vi "Main.vi"() -> ()   [LabVIEW 2018]
uses:
  <vilib>/picture/picture.llb/imagedata.ctl
  <vilib>/Utility/miscctls.llb/LVPoint32TypeDef.ctl
  <vilib>/Utility/miscctls.llb/LVMouseTypeDef.ctl
  <vilib>/Utility/miscctls.llb/LVPositionTypeDef.ctl
  <vilib>/Utility/miscctls.llb/LVPointTypeDef.ctl
  <vilib>/Utility/miscctls.llb/LVRectTypeDef.ctl
  Shared Variables/Alarm Cluster (UI).ctl
  Shared Variables/Alarm Cluster.ctl
  Drag and Drop/State Cluster.ctl
  support/Message Queue/Message Cluster.ctl
  Drag and Drop/Thumbnail Cluster.ctl
  Drag and Drop/Object Cluster.ctl
  Drag and Drop/Object Type Enum.ctl
  Config Module/Controls/Main Config Cluster.ctl
  OPC/OPC Module Config.ctl
  Scale Module Folder/Measure Instrument/State Enum.ctl
  OPC/OPC Settings.ctl
  OPC/Variable Data Cluster.ctl
  <vilib>/OPCUA/controls/NodeId.ctl
  <vilib>/OPCUA/controls/OPC UA StatusCode.ctl
  <vilib>/OPCUA/controls/Subscription ID.ctl
  <vilib>/OPCUA/controls/OPC UA Client Refnum.ctl
  <vilib>/OPCUA/controls/Subscription Data Change.ctl
  <vilib>/OPCUA/controls/Data Type.ctl
  OPC/OPC Tag Data.ctl
  Feed Module/Controls/Feed Module Config Cluster.ctl
  Feed Module/Controls/Feed Module Settings Cluster.ctl
  Ismatec ISM 831C/Controls/Ismatech ISM831C Settings Cluster.ctl
  Masterflex 7550-30/Controls/Settings Cluster.ctl
  Mettler Toledo/Controls/Settings Cluster.ctl
  Bronkhorst M13 Flow Meter/Settings Cluster.ctl
  Measure Instrument/PID 2 Parameters Cluster.ctl
  Measure Instrument/PID Input Enum.ctl
  Measure Instrument/PID 2 Output Enum.ctl
  Tacmina QI/Tacmina QI DAQ Setting.ctl
  KNF Pump/Settings Cluster plus SIMDOS.ctl
  ASIA Pump/Pump Settings.ctl
  VICI M50 Party Mode/Settings Cluster.ctl
  FLOM Pump/Settings Cluster.ctl
  SSI PR Class/SSI PR or LD Settings Cluster.ctl
  Masterflex 75211/Masterflex 75211 DAQ Setting.ctl
  SSI PR Class/SSI P40 Settings Cluster.ctl
  Ismatec 78001/Ismatec 4083.ctl
  Bronkhorst M14 Flow Meter/Settings Cluster.ctl
  TT Module/Controls/TT Module Config Cluster.ctl
  Tag VIs/Numeric Alarm Settings Cluster.ctl
  Acquisition/Hardware Configuration.ctl
  Acquisition/Task Cluster.ctl
  PT Module/Controls/PT Module Config Cluster.ctl
  Scale Module Folder/Feed Module/Controls/Scale Module Config Cluster.ctl
  Scale Module Folder/Feed Module/Controls/Scale Module Settings Cluster.ctl
  Pump Module Folder/Pump Module Config Cluster.ctl
  Pump Module Folder/Pump Module Settings Cluster.ctl
  LabJack Module/Controls/U3 Module Config Cluster.ctl
  Decoration Module/Decoration Module Config Cluster.ctl
  Flow Module Folder/Feed Module/Controls/Flow Module Config Cluster.ctl
  Flow Module Folder/Feed Module/Controls/Flow Module Settings Cluster.ctl
  TCU Module/TCU Module Folder/TCU Module Config Cluster.ctl
  TCU Module/TCU Module Folder/TCU Module Settings Cluster.ctl
  TCU Module/TCU Module Folder/Measure Instrument/Output Devices.ctl
  Huber TCU/Huber Settings.ctl
  Lauda Integral XT-150 TCU/Lauda Settings.ctl
  Julabo Type 1 TCU/Julabo Type 1 TCU Folder/Julabo FP-50 Settings.ctl
  Huber Unistat 410 TCU/Huber Unistat 410 RS485 Settings.ctl
  D-O Module Folder/Not Sure Where this is Used.ctl
  Sequencing/Squence Control.ctl
  D-O Module Folder/D-O Module Config Cluster.ctl
  D-O Module Folder/Valve Clusters.ctl
  D-O Module Folder/D-O Module Settings Cluster.ctl
  D-O Module Folder/D-O Device Settings Cluster.ctl
  VICI Electronic Actuator/VICI Electronic Actuator Settings.ctl
  Pressure Regulator Control Module/Pressure Regulator/Controls/4-20mA Module Config Cluster.ctl
  Pressure Regulator Control Module/Pressure Regulator/Controls/4-20mA Module Settings Cluster.ctl
  Pressure Transmitter/Pressure Transmitter Device Settings.ctl
  Pressure Reg Module/Pressure Regulator Device Settings.ctl
  Sonicator Module Folder/Feed Module/Controls/Sonicator Module Config Cluster.ctl
  Sonicator Module Folder/Feed Module/Controls/Sonicator Module Settings Cluster.ctl
  Tag VIs/Tag FGV Operation Enum.ctl
  Shared Variables/Alarm Log Operation Enum.ctl
  Drag and Drop/Drop Parameters Cluster.ctl
  Drag and Drop/Module Instance Number Operation Enum.ctl
  Drag and Drop/Module Type Enum.ctl
  <vilib>/Utility/error.llb/DialogType.ctl
  Config Module/Controls/Config File Operation Enum.ctl
  Waveform Loop/Start Params Cluster.ctl
  Ismatec 78001/Ismatec 4083 Global.ctl
  Ismatec 78001/Ismatec 4083 Global Element.ctl
  Pump Calibration Program/Pump Calibration Config.ctl
  support/Message Queue/Enqueue Message (Single).vi
  <vilib>/Utility/cursorutil.llb/Set Cursor (Icon Pict).vi
  Main/Main Globals.vi
  LabJack Module/U3 (Main).vit
  D-O Module Folder/D-O Module (Main).vi
  TCU Module/TCU Module Folder/TCU Module (Main).vi
  Flow Module Folder/Flow Module (Main).vi
  Sonicator Module Folder/Sonicator Module (Main).vi
  <vilib>/Utility/cursorutil.llb/Set Cursor (Cursor ID).vi
  support/Message Queue/Message Queue.lvlib
  support/User Event - Stop/User Event - Stop.lvlib
  support/Support Library.lvlib
  Drag and Drop/Drag and Drop.lvlib
  Feed Module/Feed Module.lvlib
  TT Module/TT Module.lvlib
  History Graph/History Graph.lvlib
  Waveform Loop/Waveform Loop.lvlib
  CSV Log/CSV Log.lvlib
  TDMS Log/TDMS Log.lvlib
  Shared Variables/Dynamic Shared Variables.lvlib
  DAQ/DAQ.lvlib
  Config Module/Config Module.lvlib
  Bronkhorst M13 Flow Meter/Bronkhorst M13 Flow Meter.lvlib
  Mettler Toledo/Mettler Toledo.lvlib
  Masterflex 7550-30/Masterflex 7550-30.lvlib
  Ismatec ISM 831C/Ismatec ISM 831C.lvlib
  PT Module/PT Module.lvlib
  Scale Module Folder/Scale Module.lvlib
  Pump Module Folder/Pump Module.lvlib
  <vilib>/lvdsc/NI_DSC.lvlib
  LabJack Module/U3 Module.lvlib
  Flow Module Folder/Flow Module.lvlib
  Tacmina QI/Tacmina QI.lvlib
  KNF Pump/KNF SIMDOS.lvlib
  Huber TCU/Huber Ministat 230 TCU.lvlib
  TCU Module/TCU Module Folder/TCU Module.lvlib
  Lauda Integral XT-150 TCU/Lauda TCU.lvlib
  Julabo Type 1 TCU/Julabo Type 1 TCU Folder/Julabo Type FP-50 TCU.lvlib
  ASIA Pump.lvlib
  Sequencing/Sequencing Library.lvlib
  VICI M50 Party Mode/VICI M6 M50 Party Mode.lvlib
  D-O Module Folder/D-O Module.lvlib
  Pressure Regulator Control Module/Pressure Regulator/4-20mA Module.lvlib
  Pressure Reg Module/Pressure Regulator Library.lvlib
  Pressure Transmitter/Pressure Transmitter Library.lvlib
  FLOM Pump/FLOM Pump.lvlib
  support/Command Log VIs/Command Logging.lvlib
  Calibration VIs/Calibration.lvlib
  Lauda Integral XT-150 TCU/TCP Library.lvlib
  SSI PR Class/SSI PR or LD Pump.lvlib
  Scale Module Folder/Measure Instrument/Scale Module Engine.lvlib
  OPC/OPC UA.lvlib
  D-O Module Folder/DIO Valve/VICI Electronic Actuator.lvlib
  subVIs/Main SubVIs.lvlib
  Masterflex 75211/Masterflex 75211.lvlib
  SSI PR Class/SSI P40 Pump.lvlib
  Huber Unistat 410 TCU/Huber Unistat 410 TCU.lvlib
  Ismatec 78001/Ismatec 4308.lvlib
  Bronkhorst M14 Flow Meter/Bronkhorst M14 Flow Meter.lvlib
  Sonicator Module Folder/Sonicator Module.lvlib
panel:
  out "Cluster":T1 {"Main Config"."PR Module Configs"."Settings"."PID 2 Parameters"."output range"."output low" format="%.2f"; "Main Config"."PR Module Configs"."Settings"."PID 2 Parameters"."output range"."output high" min=0.0 max=100.0 format="%.2f"; "Main Config"."PR Module Configs"."Settings"."PID 2 Parameters"."PID gains"."derivative time (Td, min)" format="%.3f"; "Main Config"."PR Module Configs"."Settings"."PID 2 Parameters"."PID gains"."integral time (Ti, min)" format="%.3f"; "Main Config"."PR Module Configs"."Settings"."PID 2 Parameters"."PID gains"."proportional gain (Kc)" format="%.3f"; "Main Config"."Steps"."Control" items=["Pump %", "Setpoint"]; "Main Config"."TCU Module Configs"."Settings"."Huber Unistat 410 Settings"."Address" min=0 max=99 format="%02.0f"; "Main Config"."TCU Module Configs"."Settings"."Julabo FP-50 Settings"."Pump Power" min=0 max=8 step=1; "Main Config"."TCU Module Configs"."Settings"."Lauda Settings"."Pump Power" min=0 max=8 step=1; "Main Config"."Flow Module Configs"."Settings"."Bronkhorst M14 Settings"."Smoothing Steps" min=1 step=1; "Main Config"."Flow Module Configs"."Settings"."Bronkhorst M13 Settings"."Smoothing Steps" min=1 step=1; "Main Config"."Pump Module Configs"."Settings"."Ismatech 3 Channel Settings"."Channel Number" min=0 max=3; "Main Config"."Pump Module Configs"."Settings"."Ismatech 3 Channel Settings"."Pump Number" min=1; "Main Config"."Pump Module Configs"."Settings"."ASIA Pump C"."channel" min=0 max=1 step=1; "Main Config"."Pump Module Configs"."Settings"."Masterflex"."Pump Number" min=1.0 max=20.0 step=1.0; "Main Config"."Pump Module Configs"."Settings"."Ismatech"."Pump Number" min=1.0 max=20.0 step=1.0; "Main Config"."Feed Module Configs"."Settings"."Bronkhorst M14 Settings"."Smoothing Steps" min=1 step=1; "Main Config"."Feed Module Configs"."Settings"."Ismatech 3 Channel Settings"."Channel Number" min=0 max=3; "Main Config"."Feed Module Configs"."Settings"."Ismatech 3 Channel Settings"."Pump Number" min=1; "Main Config"."Feed Module Configs"."Settings"."output range"."output low" min=0.0 max=100.0 format="%.2f"; "Main Config"."Feed Module Configs"."Settings"."output range"."output high" format="%.2f"; "Main Config"."Feed Module Configs"."Settings"."PID 2 Parameters"."PID gains"."derivative time (Td, min)" format="%.3f"; "Main Config"."Feed Module Configs"."Settings"."PID 2 Parameters"."PID gains"."integral time (Ti, min)" format="%.3f"; "Main Config"."Feed Module Configs"."Settings"."PID 2 Parameters"."PID gains"."proportional gain (Kc)" format="%.3f"; "Main Config"."Feed Module Configs"."Settings"."Bronkhorst M13 Flow Meter"."Smoothing Steps" min=1 step=1; "Main Config"."Feed Module Configs"."Settings"."ASIA Pump C"."channel" min=0 max=1 step=1; "Main Config"."Feed Module Configs"."Settings"."Ismatech"."Pump Number" min=1.0 max=20.0 step=1.0; "Main Config"."Feed Module Configs"."Settings"."Masterflex"."Pump Number" min=1.0 max=20.0 step=1.0}
  in  "Alarm History Button":bool
  out "Alarm Model":T70[](array[typedef]) {"Alarm"."value" format="%.2f"; "Alarm"."setpoint" format="%.2f"; "Alarm"."clear time" format="%<%X\n%x>T"; "Alarm"."ack time" format="%<%X\n%x>T"; "Alarm"."set time" format="%<%X\n%x>T"}
  in  "UI Alarms":T71[](array[typedef])
  out "Message Data":variant
  out "data":errorcluster
  in  "End Program":bool
  out "CSV Log File":path
  out "error out":errorcluster
  in  "E-Stop":bool
  out "x-y":T4
  out "Front Panel Window:Panel Bounds":T4
  out "Drop Offset":T6
  out "Origin":T72
  out "Position":T6
  out "output cluster":cluster{"Coords":T10, "Mouse":T73}
  out "Mouse Position":cluster{"X":i32, "Y":i32}
  out "Path":path
  out "index of element":i32
  out "image data":T74
  in  "Notebook":string="Test"
  in  "Exit":bool
  in  "Settings":bool
  in  "Pause Log Button":bool
  in  "Force Trigger":bool
  in  "Start Log":bool
  out "Canvas":picture
  out "Palette":picture
  in  "?":T1 {"Main Config"."PR Module Configs"."Settings"."PID 2 Parameters"."output range"."output low" format="%.2f"; "Main Config"."PR Module Configs"."Settings"."PID 2 Parameters"."output range"."output high" min=0.0 max=100.0 format="%.2f"; "Main Config"."PR Module Configs"."Settings"."PID 2 Parameters"."PID gains"."derivative time (Td, min)" format="%.3f"; "Main Config"."PR Module Configs"."Settings"."PID 2 Parameters"."PID gains"."integral time (Ti, min)" format="%.3f"; "Main Config"."PR Module Configs"."Settings"."PID 2 Parameters"."PID gains"."proportional gain (Kc)" format="%.3f"; "Main Config"."Steps"."Control" items=["Pump %", "Setpoint"]; "Main Config"."TCU Module Configs"."Settings"."Huber Unistat 410 Settings"."Address" min=0 max=99 format="%02.0f"; "Main Config"."TCU Module Configs"."Settings"."Julabo FP-50 Settings"."Pump Power" min=0 max=8 step=1; "Main Config"."TCU Module Configs"."Settings"."Lauda Settings"."Pump Power" min=0 max=8 step=1; "Main Config"."Flow Module Configs"."Settings"."Bronkhorst M14 Settings"."Smoothing Steps" min=1 step=1; "Main Config"."Flow Module Configs"."Settings"."Bronkhorst M13 Settings"."Smoothing Steps" min=1 step=1; "Main Config"."Pump Module Configs"."Settings"."Ismatech 3 Channel Settings"."Channel Number" min=0 max=3; "Main Config"."Pump Module Configs"."Settings"."Ismatech 3 Channel Settings"."Pump Number" min=1; "Main Config"."Pump Module Configs"."Settings"."ASIA Pump C"."channel" min=0 max=1 step=1; "Main Config"."Pump Module Configs"."Settings"."Masterflex"."Pump Number" min=1.0 max=20.0 step=1.0; "Main Config"."Pump Module Configs"."Settings"."Ismatech"."Pump Number" min=1.0 max=20.0 step=1.0; "Main Config"."Feed Module Configs"."Settings"."Bronkhorst M14 Settings"."Smoothing Steps" min=1 step=1; "Main Config"."Feed Module Configs"."Settings"."Ismatech 3 Channel Settings"."Channel Number" min=0 max=3; "Main Config"."Feed Module Configs"."Settings"."Ismatech 3 Channel Settings"."Pump Number" min=1; "Main Config"."Feed Module Configs"."Settings"."output range"."output low" min=0.0 max=100.0 format="%.2f"; "Main Config"."Feed Module Configs"."Settings"."output range"."output high" format="%.2f"; "Main Config"."Feed Module Configs"."Settings"."PID 2 Parameters"."PID gains"."derivative time (Td, min)" format="%.3f"; "Main Config"."Feed Module Configs"."Settings"."PID 2 Parameters"."PID gains"."integral time (Ti, min)" format="%.3f"; "Main Config"."Feed Module Configs"."Settings"."PID 2 Parameters"."PID gains"."proportional gain (Kc)" format="%.3f"; "Main Config"."Feed Module Configs"."Settings"."Bronkhorst M13 Flow Meter"."Smoothing Steps" min=1 step=1; "Main Config"."Feed Module Configs"."Settings"."ASIA Pump C"."channel" min=0 max=1 step=1; "Main Config"."Feed Module Configs"."Settings"."Ismatech"."Pump Number" min=1.0 max=20.0 step=1.0; "Main Config"."Feed Module Configs"."Settings"."Masterflex"."Pump Number" min=1.0 max=20.0 step=1.0}
  # "little pump\ncentrifigual pump\nflow rate\npressure\nS or P to the left\nsolvent or process"
  # "Question: how do we make the live VI, such as the feed module graphic\nsized right for the picture that is loaded?\n\nProbably should standarize each module size. Then the  flow sheet\ndrawings will all just match the size and we don't have to worry about\nscale."
  # "Tasks\n1. Load graphic\n2. Drag and drop onto picture control\n3. Picture control draws hot spot\n4. If drag and drop on picture control, then resize and redraw the nearest hotspot\n5. When operator turns \"ON\" the system, then the hotspots are replaced with actual VIs."
  # "vertical or horizontal lines\nextendable"
  # "as much drawing room as possible"
  # "Scale Settings"
  # "Instrument Settings"
  # "Instrument Settings"
  # "Output Instruments"
  # "Flow Meter Settings"
  # "Output Instruments"
  # "Scale Settings"
  # "Output Instruments"
  # "Input Instruments"
  # "Scale Settings"
  # "Instrument Settings"
  # "Instrument Settings"
  # "Output Instruments"
  # "Flow Meter Settings"
  # "Output Instruments"
  # "Scale Settings"
  # "Output Instruments"
  # "Input Instruments"
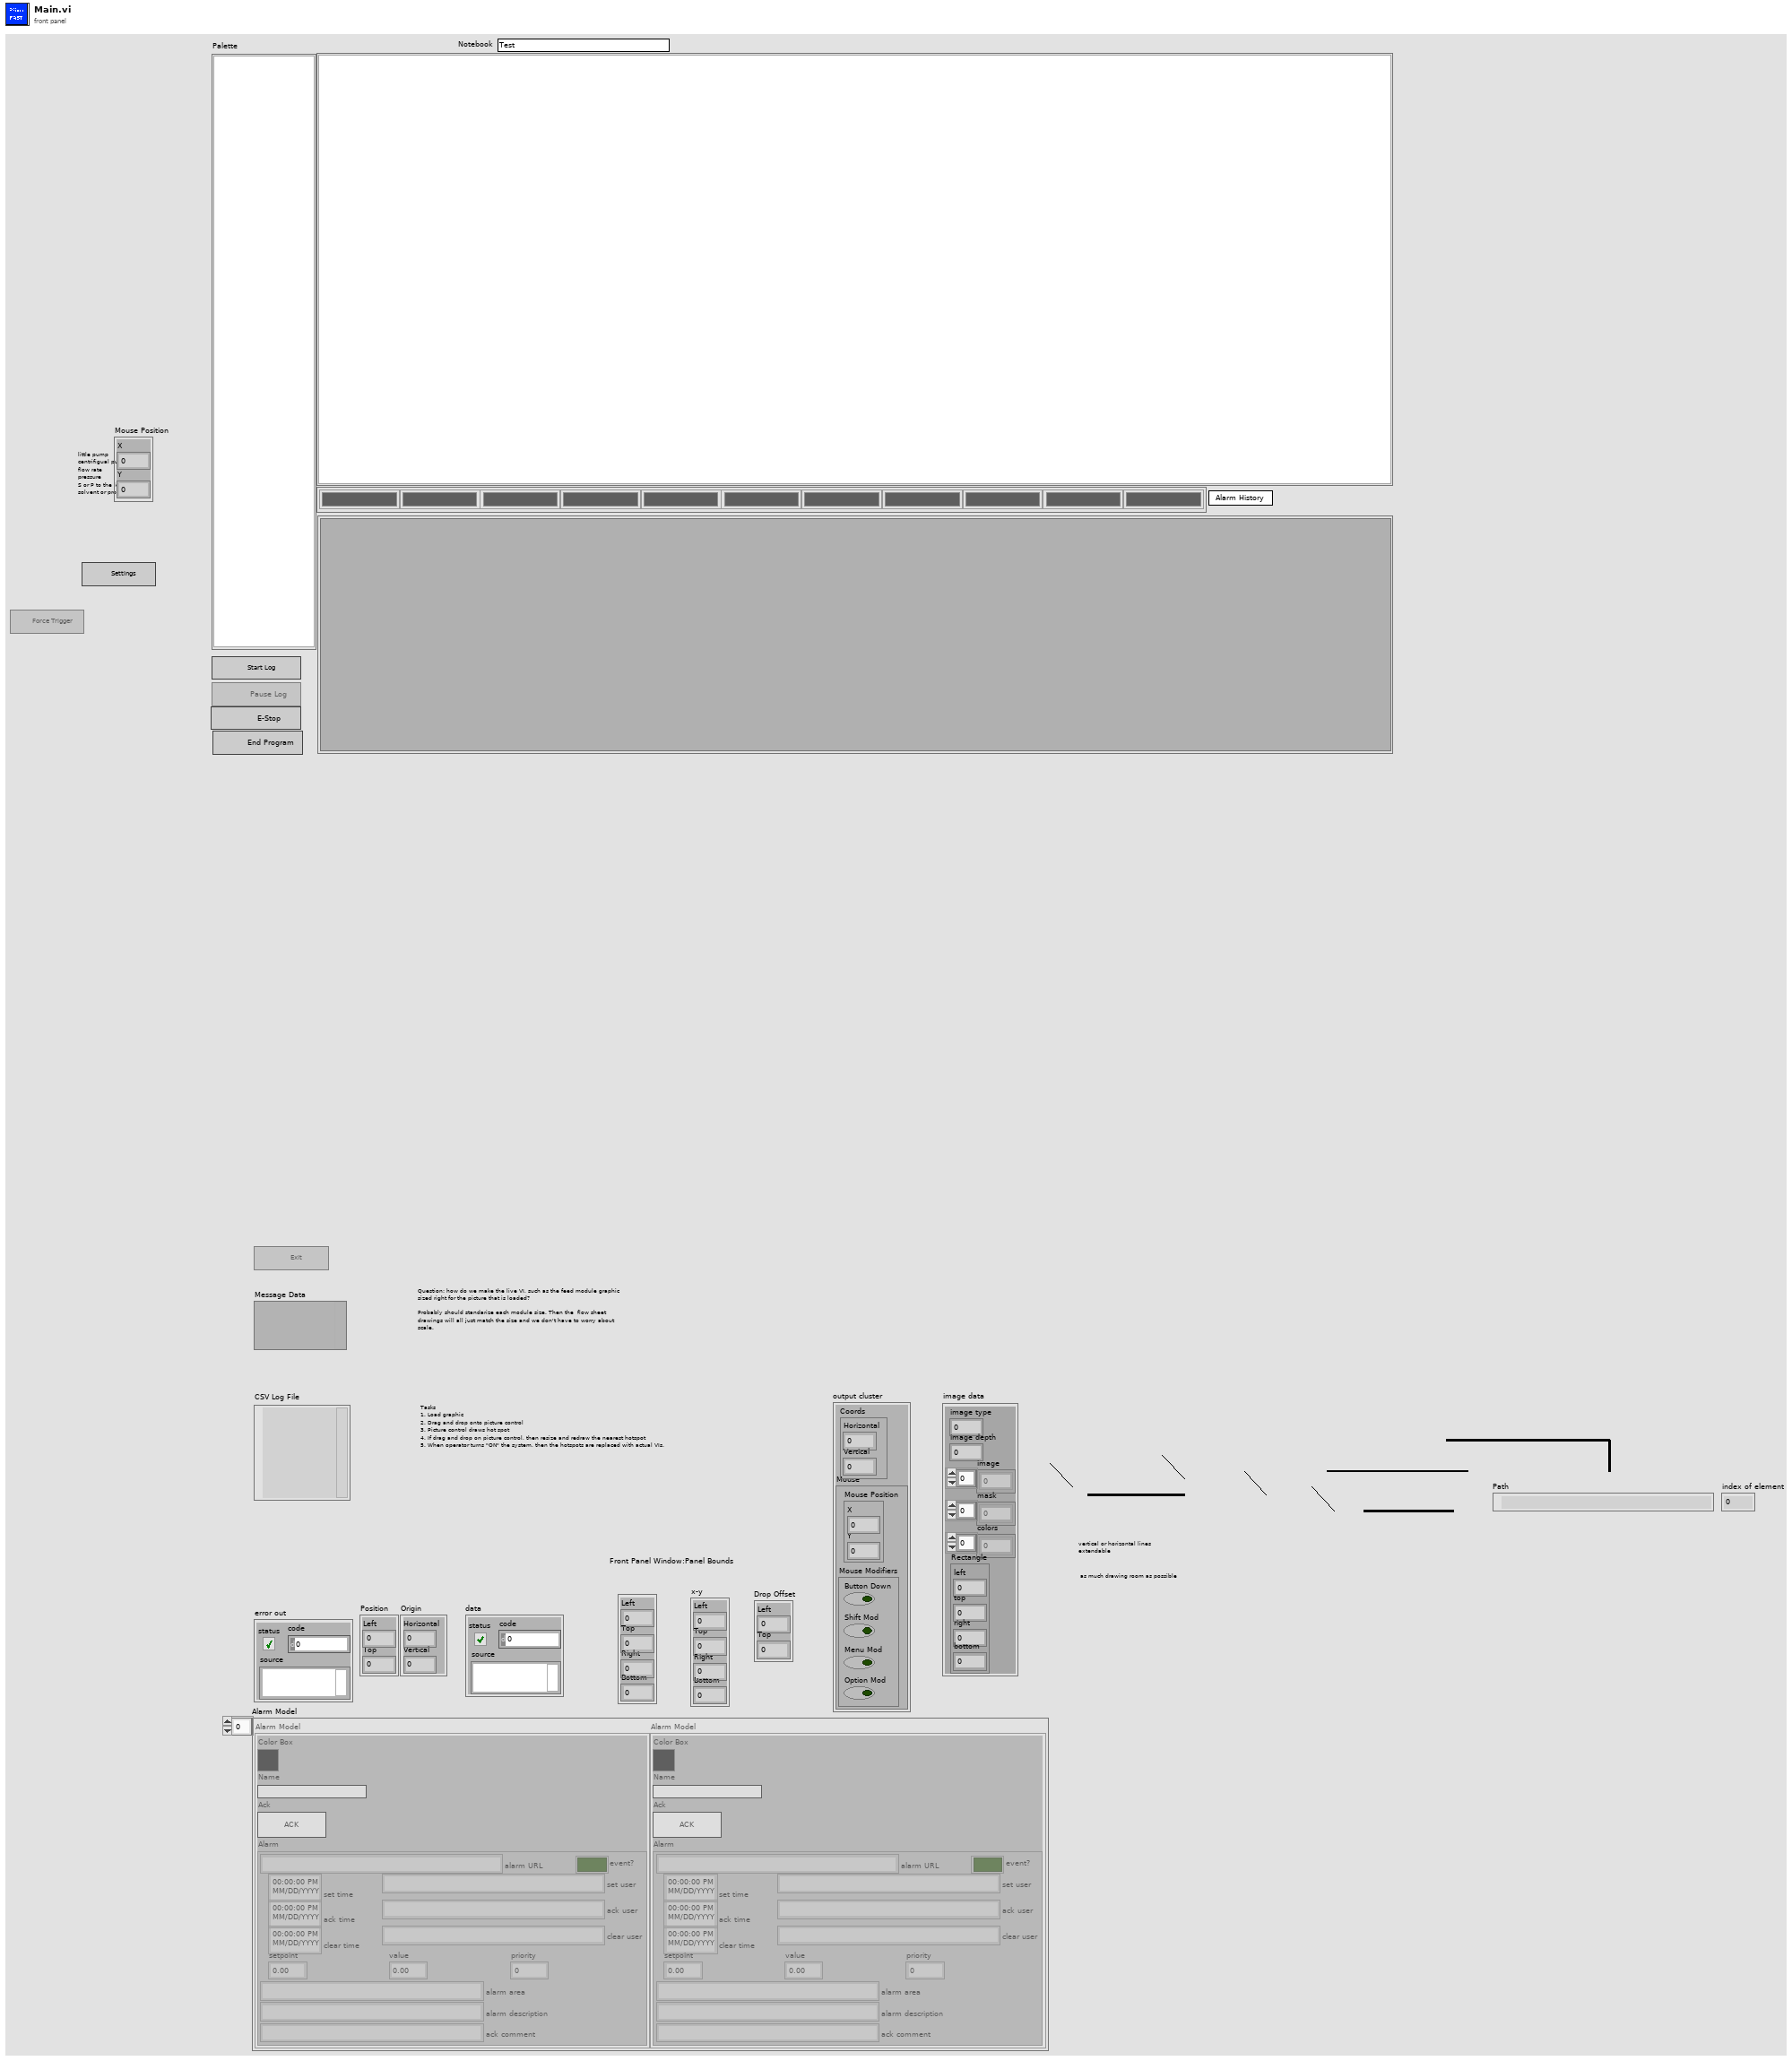
[diagram p1: front panel]
types:
  T1 = typedef "Drag and Drop.lvlib/State Cluster.ctl" = cluster{"VI refs":refnum<vi>[], "Queues":refnum<queue>[], "[Thumbnails]":T2[], "Drag Object Idx":i32, "[Objects]":T3[], "Active Object":i32, "Drop Offset":T6, "Process Name":string, "Main Config":T7, "Campaign Filepath":path, "Config Changed?":bool}
  T2 = typedef "Thumbnail Cluster.ctl" = cluster{"Path":path, "Rectangle":cluster{"left":i16, "top":i16, "right":i16, "bottom":i16}}
  T3 = typedef "Object Cluster.ctl" = cluster{"BMP Path":path, "Anchor Position":cluster{"X":i32, "Y":i32}, "Hot Spot":T4, "Type":T5, "Parameters":variant}
  T4 = typedef "LVRectTypeDef.ctl" = cluster{"Left":i16, "Top":i16, "Right":i16, "Bottom":i16}
  T5 = typedef "Object Type Enum.ctl" = enum16{"Icon", "Line", "Text", "Feed Module"}
  T6 = typedef "LVPositionTypeDef.ctl" = cluster{"Left":i32, "Top":i32}
  T7 = typedef "Config Module.lvlib/Main Config Cluster.ctl" = cluster{"Notebook":string, "OPC Module Configs":T8[], "Feed Module Configs":T18[], "Log File Path":path, "TT Module Configs":T37[], "DAQ Config":T39, "PT Module Configs":T41[], "Scale Module Configs":T42[], "Pump Module Configs":T44[], "U3 Module Configs":T46[], "Decoration Module Configs":T47[], "Flow Module Configs":T48[], "TCU Module Configs":T50[], "Steps":T57, "Abort":bool, "DO Module Configs":T59[], "PR Module Configs":T64[], "SC Module Configs":T68[], "Cycle Period":dbl}
  T8 = typedef "OPC UA.lvlib/OPC Module Config.ctl" = cluster{"State":T9, "GUID":string, "Drop Coords":T10, "Configuration":T11, "First Iteration":bool, "Data":cluster{"Object Name":string, "Variable Array":T12[]}[], "Process Name":string, "Load Count":i32, "Log Started":bool, "subscription ID out":T15, "OPC UA client refnum out":T16, "Event Registration Refnum":refnum<event-registration>, "Start Time":timestamp, "Current Time":timestamp, "Tag Data":T17[]}
  T9 = typedef "Scale Module.lvlib/Scale Module Engine.lvlib/State Enum.ctl" = enum16{"Measuring", "Idle"}
  T10 = typedef "LVPoint32TypeDef.ctl" = cluster{"Horizontal":i32, "Vertical":i32}
  T11 = typedef "OPC UA.lvlib/OPC Settings.ctl" = cluster{"Cycle Period":dbl, "server endpoint URL":string, "security policy":cluster{"message mode":enum16{"None", "Sign", "Sign and Encrypt"}, "security":enum16{"Basic256", "Basic128Rsa15"}}, "Trust Any Server":bool}
  T12 = typedef "OPC UA.lvlib/Variable Data Cluster.ctl" = cluster{"node ID":T13, "browse name":string, "status":T14, "timestamp":timestamp, "value ":variant}
  T13 = typedef "NodeId.ctl" = string
  T14 = typedef "OPC UA StatusCode.ctl" = u32
  T15 = typedef "Subscription ID.ctl" = u32
  T16 = typedef "OPC UA Client Refnum.ctl" = refnum<k21>
  T17 = typedef "OPC UA.lvlib/OPC Tag Data.ctl" = cluster{"Include this Device":bool, "Device Name":string, "OPC Tag Data":cluster{"Tag":string, "Value":variant, "Time Stamp":timestamp}[]}
  T18 = typedef "Feed Module.lvlib/Feed Module Config Cluster.ctl" = cluster{"GUID":string, "Drop Coords":T10, "Process Name":string, "Queue Name":string, "Settings":T19, "Settings Load Count":i32, "OP Load Count":i32}
  T19 = typedef "Feed Module.lvlib/Feed Module Settings Cluster.ctl" = cluster{"Cycle Period":dbl, "Ismatech":T20, "Masterflex":T21, "Mettler":T22, "Bronkhorst M13 Flow Meter":T23, "PID 2 Parameters":T24, "Manual Entry":dbl, "Auto?":bool, "output range":cluster{"output high":dbl, "output low":dbl}, "Tacmina Settings":T27, "KNF SIMDOS Settings":T28, "ASIA Pump C":T29, "VICI Settings":T30, "FLOM Settings":T31, "SSI PR/LD Settings":T32, "Masterflex 75211 Settings":T33, "SSI P40 Settings":T34, "Ismatech 3 Channel Settings":T35, "Bronkhorst M14 Settings":T36}
  T20 = typedef "Ismatec ISM 831C.lvlib/Ismatech ISM831C Settings Cluster.ctl" = cluster{"VISA resource name":refnum<visa-resource-name>, "Simulated?":bool, "Pump Number":dbl, "Reverse?":bool}
  T21 = typedef "Masterflex 7550-30.lvlib/Settings Cluster.ctl" = cluster{"VISA resource name":refnum<visa-resource-name>, "Simulated?":bool, "Pump Number":dbl, "Reverse?":bool}
  T22 = typedef "Mettler Toledo.lvlib/Settings Cluster.ctl" = cluster{"VISA resource name":refnum<visa-resource-name>, "Simulated?":bool}
  T23 = typedef "Bronkhorst M13 Flow Meter.lvlib/Settings Cluster.ctl" = cluster{"VISA resource name":refnum<visa-resource-name>, "Simulated?":bool, "Smoothing Steps":i32}
  T24 = typedef "PID 2 Parameters Cluster.ctl" = cluster{"Input Device":T25, "Output Device":T26, "Setpoint":dbl, "PID gains":cluster{"proportional gain (Kc)":dbl, "integral time (Ti, min)":dbl, "derivative time (Td, min)":dbl}}
  T25 = typedef "PID Input Enum.ctl" = enum16{"Default", "Bronkhorst M13", "Bronkhorst M14", "Scale Rate of Change"}
  T26 = typedef "PID 2 Output Enum.ctl" = enum16{"Default", "Ismatec ISM 4308", "Ismatec ISM 831C", "Masterflex 7550-30", "VICI", "Tacmina QI", "KNF SIMDOS", "ASIA Type C", "FLOM UI-22-11", "SSI PR/LD", "SSI P40", "Masterflex 75211-70"}
  T27 = typedef "Tacmina QI.lvlib/Tacmina QI DAQ Setting.ctl" = cluster{"Analog DAQ Task":refnum<k21>, "Digital DAQ Task":refnum<k21>}
  T28 = typedef "KNF SIMDOS.lvlib/Settings Cluster plus SIMDOS.ctl" = cluster{"VISA resource name":refnum<visa-resource-name>, "Simulated?":bool}
  T29 = typedef "ASIA Pump.lvlib/Pump Settings.ctl" = cluster{"ASIA Pump #":i32, "channel":i32, "Simulated":bool}
  T30 = typedef "VICI M6 M50 Party Mode.lvlib/Settings Cluster.ctl" = cluster{"VISA resource name":refnum<visa-resource-name>, "Simulated?":bool, "Pump Letter":string, "Reverse?":bool}
  T31 = typedef "FLOM Pump.lvlib/Settings Cluster.ctl" = cluster{"VISA resource name":refnum<visa-resource-name>, "Simulated?":bool, "Pump Number":dbl}
  T32 = typedef "SSI PR or LD Pump.lvlib/SSI PR or LD Settings Cluster.ctl" = cluster{"VISA resource name":refnum<visa-resource-name>, "Simulated?":bool}
  T33 = typedef "Masterflex 75211.lvlib/Masterflex 75211 DAQ Setting.ctl" = cluster{"Analog DAQ Task":refnum<k21>, "Digital DAQ Task":refnum<k21>}
  T34 = typedef "SSI P40 Pump.lvlib/SSI P40 Settings Cluster.ctl" = cluster{"VISA resource name":refnum<visa-resource-name>, "Simulated?":bool}
  T35 = typedef "Ismatec 4308.lvlib/Ismatec 4083.ctl" = cluster{"VISA resource name":refnum<visa-resource-name>, "Pump Number":i16, "Channel Number":i16, "Simulated?":bool, "Reverse?":bool}
  T36 = typedef "Bronkhorst M14 Flow Meter.lvlib/Settings Cluster.ctl" = cluster{"VISA resource name":refnum<visa-resource-name>, "Simulated?":bool, "Smoothing Steps":i32}
  T37 = typedef "TT Module.lvlib/TT Module Config Cluster.ctl" = cluster{"GUID":string, "Drop Coords":T10, "Input Channel Tag Name ":string, "Process Name":string, "Queue Name":string, "Input Channel Numeric Alarm Settings":T38[]}
  T38 = typedef "Numeric Alarm Settings Cluster.ctl" = cluster{"enable? (F)":bool, "name":string, "alarm type":enum16{"HI_HI", "HI", "LO", "LO_LO"}, "level/change":dbl, "deadband/time":dbl, "alarm delay":dbl, "priority":u32, "ack type":enum16{"Auto", "User", "None", "Each Occurrence"}, "area":string, "description":string, "log? (T)":bool}
  T39 = typedef "DAQ.lvlib/Hardware Configuration.ctl" = cluster{"Tasks":T40[]}
  T40 = typedef "Task Cluster.ctl" = cluster{"DAQmx Task":refnum<k21>, "Read-Write Radio":enum32{"Read", "Write"}}
  T41 = typedef "PT Module.lvlib/PT Module Config Cluster.ctl" = cluster{"GUID":string, "Drop Coords":T10, "Input Channel Tag Name ":string, "Process Name":string, "Queue Name":string, "Input Channel Numeric Alarm Settings":T38[]}
  T42 = typedef "Scale Module.lvlib/Scale Module Config Cluster.ctl" = cluster{"GUID":string, "Drop Coords":T10, "Process Name":string, "Queue Name":string, "Settings":T43, "Load Count":i32}
  T43 = typedef "Scale Module.lvlib/Scale Module Settings Cluster.ctl" = cluster{"Cycle Period":dbl, "Mettler":T22, "Scale Type":string}
  T44 = typedef "Pump Module.lvlib/Pump Module Config Cluster.ctl" = cluster{"GUID":string, "Drop Coords":T10, "Process Name":string, "Queue Name":string, "Settings":T45, "Load Count":i32}
  T45 = typedef "Pump Module.lvlib/Pump Module Settings Cluster.ctl" = cluster{"Cycle Period":dbl, "Manual Entry":dbl, "Output Device":T26, "Ismatech":T20, "Ismatech 3 Channel Settings":T35, "Masterflex":T21, "VICI Settings":T30, "Tacmina Settings":T27, "KNF SIMDOS Settings":T28, "ASIA Pump C":T29, "FLOM Settings":T31, "SSI PR/LD Settings":T32, "SSI P40 Settings":T32, "Masterflex 75211 Settings":T33, "Pump Calibration File":path, "Calibration Slope":dbl, "Calibration Y Intercept":dbl, "Pump Cal Enum":u16}
  T46 = typedef "U3 Module.lvlib/U3 Module Config Cluster.ctl" = cluster{"GUID":string, "Drop Coords":T10, "AI Channel Number":enum16{"Default", "AI0", "AI1", "AI2", "AI3", "AI4", "AI5", "AI6", "AI7"}, "Process Name":string, "Queue Name":string, "Input Channel Numeric Alarm Settings":T38[]}
  T47 = typedef "Decoration Module Config Cluster.ctl" = cluster{"GUID":string, "Drop Coords":T10, "Decoration Filepath":path}
  T48 = typedef "Flow Module.lvlib/Flow Module Config Cluster.ctl" = cluster{"GUID":string, "Drop Coords":T10, "Process Name":string, "Queue Name":string, "Settings":T49, "Load Count":i32}
  T49 = typedef "Flow Module.lvlib/Flow Module Settings Cluster.ctl" = cluster{"Cycle Period":dbl, "Flow Meter Type":string, "Bronkhorst M13 Settings":T23, "Bronkhorst M14 Settings":T36}
  T50 = typedef "TCU Module.lvlib/TCU Module Config Cluster.ctl" = cluster{"GUID":string, "Drop Coords":T10, "Process Name":string, "Queue Name":string, "Settings":T51, "Load Count":i32, "Power Level Changed":bool}
  T51 = typedef "TCU Module.lvlib/TCU Module Settings Cluster.ctl" = cluster{"Cycle Period":dbl, "Setpoint Entry":dbl, "Output Device":T52, "Huber Ministat 230 Settings":T53, "Lauda Settings":T54, "Julabo FP-50 Settings":T55, "Internal Control?":bool, "Huber Unistat 410 Settings":T56}
  T52 = typedef "Output Devices.ctl" = enum16{"Default", "Huber Ministat 230", "Huber Unistat 410", "Lauda XT-150", "Julabo FP-50"}
  T53 = typedef "Huber Ministat 230 TCU.lvlib/Huber Settings.ctl" = cluster{"VISA resource name":refnum<visa-resource-name>, "Simulated?":bool}
  T54 = typedef "Lauda TCU.lvlib/Lauda Settings.ctl" = cluster{"VISA resource name":refnum<visa-resource-name>, "Simulated?":bool, "Pump Power":i32}
  T55 = typedef "Julabo Type FP-50 TCU.lvlib/Julabo FP-50 Settings.ctl" = cluster{"VISA resource name":refnum<visa-resource-name>, "Simulated?":bool, "Pump Power":i32}
  T56 = typedef "Huber Unistat 410 TCU.lvlib/Huber Unistat 410 RS485 Settings.ctl" = cluster{"VISA resource name":refnum<visa-resource-name>, "Address":i8, "Simulated?":bool}
  T57 = typedef "Not Sure Where this is Used.ctl" = T58[]
  T58 = typedef "Sequencing Library.lvlib/Squence Control.ctl" = cluster{"Module":string, "Control":u16, "Value":dbl, "Wait (sec)":dbl}
  T59 = typedef "D-O Module.lvlib/D-O Module Config Cluster.ctl" = cluster{"GUID":string, "Drop Coords":T10, "Process Name":string, "Queue Name":string, "Settings":T60, "Load Count":i32}
  T60 = typedef "D-O Module.lvlib/Valve Clusters.ctl" = cluster{"Valve Settings":T61, "Valve Type":enum16{"Default", "Digital Output Valve", "VICI Electronic Actuator"}, "Time On (Sec)":dbl, "Time Off (Sec)":dbl, "Run?":bool}
  T61 = typedef "D-O Module.lvlib/D-O Module Settings Cluster.ctl" = cluster{"D-O Settings":T62, "VICI Electronic Actuator":T63}
  T62 = typedef "D-O Module.lvlib/D-O Device Settings Cluster.ctl" = cluster{"DAQmx Task Name":refnum<k21>, "Output Channel":u16, "Output Channel Names":string[]}
  T63 = typedef "VICI Electronic Actuator.lvlib/VICI Electronic Actuator Settings.ctl" = cluster{"VISA resource name":refnum<visa-resource-name>, "Mode":enum16{"Two Positions With Stops", "Two Positions Without Stops", "Mutiposition"}, "Simulated":bool}
  T64 = typedef "4-20mA Module.lvlib/4-20mA Module Config Cluster.ctl" = cluster{"GUID":string, "Drop Coords":T10, "Process Name":string, "Queue Name":string, "Settings":T65, "Settings Load Count":i32}
  T65 = typedef "4-20mA Module.lvlib/4-20mA Module Settings Cluster.ctl" = cluster{"Cycle Period":dbl, "PID 2 Parameters":cluster{"Input Device":enum16{"Default", "4-20mA"}, "Output Device":enum16{"Default", "Equilibar Pressure Reg", "Flow Regulator"}, "Setpoint":dbl, "PID gains":cluster{"proportional gain (Kc)":dbl, "integral time (Ti, min)":dbl, "derivative time (Td, min)":dbl}, "output range":cluster{"output low":dbl, "output high":dbl}}, "Manual Entry":dbl, "Auto?":bool, "4-20mA Input Settings":T66, "4-20mA Out Settings":T67, "Input Channel Tag Name ":string}
  T66 = typedef "Pressure Transmitter Library.lvlib/Pressure Transmitter Device Settings.ctl" = cluster{"Input Channel ":u16}
  T67 = typedef "Pressure Regulator Library.lvlib/Pressure Regulator Device Settings.ctl" = cluster{"Output DAQ Task":refnum<k21>}
  T68 = typedef "Sonicator Module.lvlib/Sonicator Module Config Cluster.ctl" = cluster{"GUID":string, "Drop Coords":T10, "Process Name":string, "Queue Name":string, "Settings":T69, "Load Count":i32}
  T69 = typedef "Sonicator Module.lvlib/Sonicator Module Settings Cluster.ctl" = cluster{"Cycle Period":dbl, "Mettler":T22, "Scale Type":string}
  T70 = typedef "Dynamic Shared Variables.lvlib/Alarm Cluster.ctl" = cluster{"Color Box":u32, "Name":string, "Ack":bool, "Alarm":cluster{"alarm URL":string, "set time":timestamp, "set user":string, "ack time":timestamp, "ack user":string, "clear time":timestamp, "clear user":string, "setpoint":dbl, "value":dbl, "priority":u32, "alarm area":string, "alarm description":string, "ack comment":string, "event?":bool, "Refnum":u64}}
  T71 = typedef "Dynamic Shared Variables.lvlib/Alarm Cluster (UI).ctl" = cluster{"Color Box":u32, "Name":string, "Ack":bool}
  T72 = typedef "LVPointTypeDef.ctl" = cluster{"Horizontal":i16, "Vertical":i16}
  T73 = typedef "LVMouseTypeDef.ctl" = cluster{"Mouse Position":cluster{"X":i32, "Y":i32}, "Mouse Modifiers":cluster{"Button Down":bool, "Shift Mod":bool, "Menu Mod":bool, "Option Mod":bool}}
  T74 = typedef "imagedata.ctl" = cluster{"image type":i32, "image depth":i32, "image":u8[], "mask":u8[], "colors":u32[], "Rectangle":cluster{"left":i16, "top":i16, "right":i16, "bottom":i16}}
  T75 = typedef "Tag FGV Operation Enum.ctl" = enum16{"Init", "Set Notification Queue", "Create Tag", "Commit", "Write Tag (Numeric)", "Write Tag (Boolean)", "Read All Tags", "Read One Tag", "Delete Tag Category", "Set Alarm Parameters (Numeric)", "Set Alarm Parameters (Boolean)", "Enable All Alarms", "Disable All Alarms", "Delete All Tags", "Read Alarms", "Ack Alarm", "Read Alarm Parameters (Numeric)", "Read Alarm Parameters (Boolean)"}
  T76 = cluster{"Down":bool, "Mouse":T73, "Drag":bool, "Canvas":bool}
  T77 = cluster{"Busy":bool, "PumpCnt":dbl, "RemoteEntered":bool, "OverpressureSet":bool}[]
  T78 = typedef "Main Queue Cluster.ctl" = cluster{"UI":refnum<queue>, "Waveform Loop":refnum<queue>, "CSV Log":refnum<queue>, "TDMS Log":refnum<queue>, "Graphs":refnum<queue>[], "DAQ":refnum<queue>, "Sequence":refnum<queue>, "TCP Write":refnum<queue>, "Sequence UI":refnum<queue>, "OPC UA Log":refnum<queue>, "TCP Read":refnum<queue>}
  T79 = cluster{"Event Registration Refnum":refnum<event-registration>, "Stop Event Registration Refnum":refnum<event-registration>}
  T80 = typedef "Drag and Drop.lvlib/Module Type Enum.ctl" = enum16{"<unknown module>", "Feed", "TT", "PT", "Scale", "Flow", "Pump", "U3", "TCU", "DO", "PR", "OPC", "SC"}
  T81 = typedef "Module Instance Number Operation Enum.ctl" = enum16{"Init", "Next Instance Number"}
  T82 = typedef "Drop Parameters Cluster.ctl" = cluster{"Module VI Filepath":path, "Process Name":string, "Main UI Message Queue":refnum<queue>, "Drop Coords":T10, "Module Parameters":variant, "Name of Parent Window":string}
  T83 = enum8{"Enabled", "Disabled", "Disabled and Grayed Out"}
  T84 = typedef "Config Module.lvlib/Config File Operation Enum.ctl" = enum16{"Read", "Write"}
  T85 = typedef "Alarm Log Operation Enum.ctl" = enum16{"Create Log", "Log Alarm", "Close Log"}
  T86 = typedef "Waveform Loop.lvlib/Start Params Cluster.ctl" = cluster{"dt (seconds)":dbl, "CSV Logfile path":path, "TDMS Logfile path":path}
  T87 = typedef "Ismatec 4308.lvlib/Ismatec 4083 Global.ctl" = T88[]
  T88 = typedef "Ismatec 4308.lvlib/Ismatec 4083 Global Element.ctl" = cluster{"Busy":bool, "ChannelCnt":dbl, "Initialized":bool, "Current Channel":dbl, "Initialized Channels":dbl[]}
  T89 = typedef "Calibration.lvlib/Pump Calibration Config.ctl" = cluster{"Settings":cluster{"Cycle Period":dbl, "Ismatech":T20, "Masterflex":T21, "Bronkhorst M13 Settings":T23, "PID 2 Parameters":cluster{"Input Device":T25, "Output Device":T26}, "Tacmina Settings":T27, "KNF SIMDOS Settings":T28, "VICI M50 Settings":T30, "FLOM Settings":T31, "Calibration Limits":cluster{"Minimum (ml/min)":dbl, "Maximum (ml/min)":dbl, "Steps":dbl}, "SSI PR Settings":T32, "Ismatech 4308 Settings":T35, "Bronkhorst M14 Settings":T36}, "Flowmeter Output":dbl, "Density":dbl, "FL Temp":dbl, "Speed %":dbl, "File Refnum":refnum<file>, "Pump On?":enum16{"Off", "On", "Not Initialized"}}
  T90 = typedef "DialogType.ctl" = u16
  T91 = enum32{"Invalid", "Standard", "Closed", "Hidden", "Minimized", "Maximized"}
  T92 = cluster{"alarm URL":string, "set time":timestamp, "set user":string, "ack time":timestamp, "ack user":string, "clear time":timestamp, "clear user":string, "setpoint":dbl, "value":dbl, "priority":u32, "alarm area":string, "alarm description":string, "ack comment":string, "event?":bool, "Refnum":u64}[]
  T93 = cluster{"alarm URL":string, "set time":timestamp, "set user":string, "ack time":timestamp, "ack user":string, "clear time":timestamp, "clear user":string, "setpoint":dbl, "value":dbl, "priority":u32, "alarm area":string, "alarm description":string, "ack comment":string, "event?":bool, "Refnum":u64}
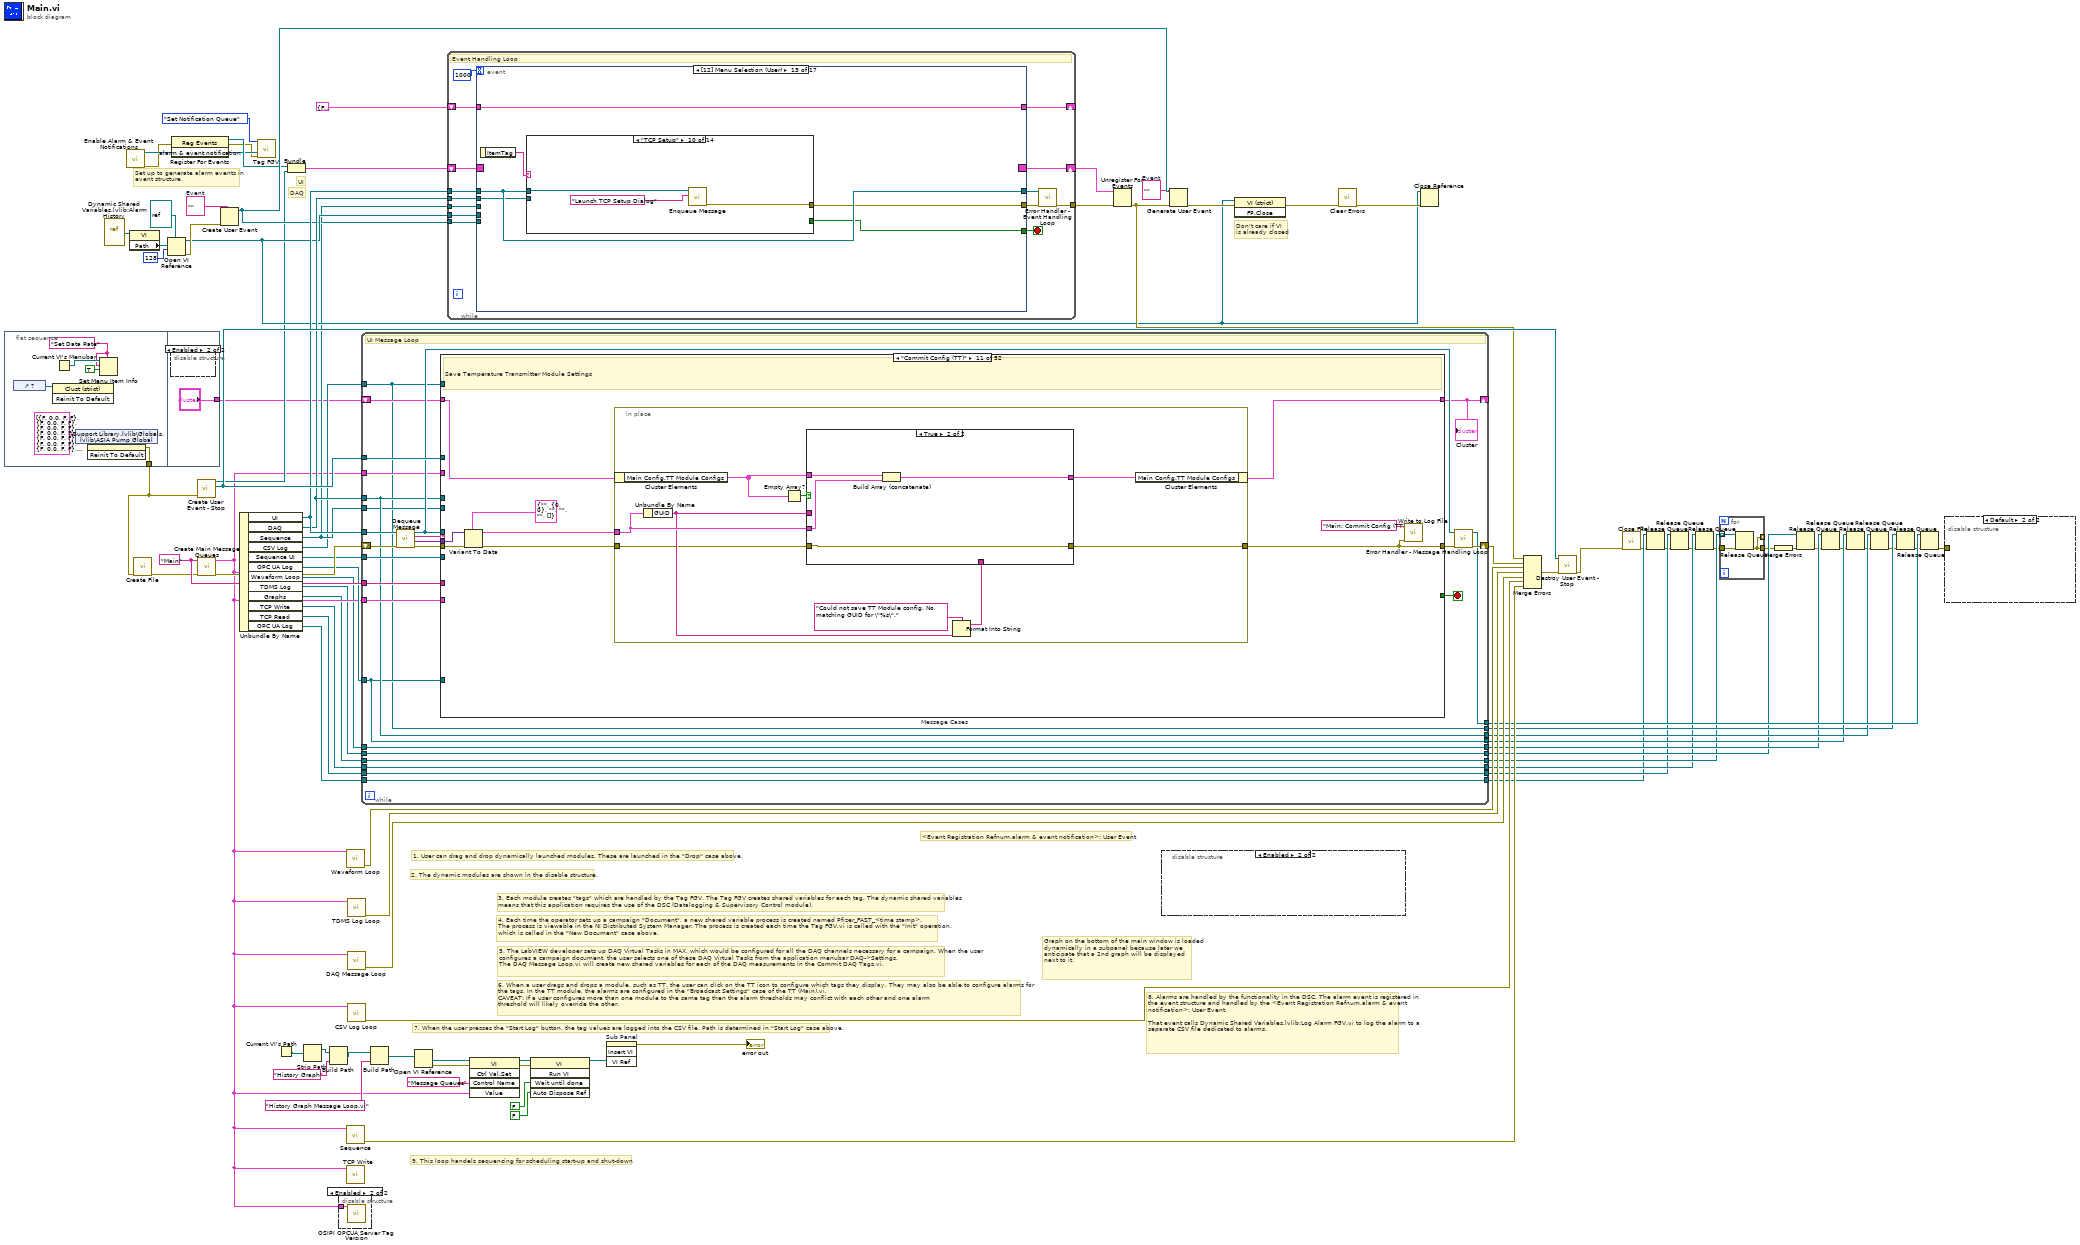
[diagram p0: block diagram]
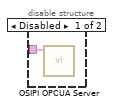
[diagram p2: hidden frame]
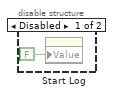
[diagram p3: hidden frame]
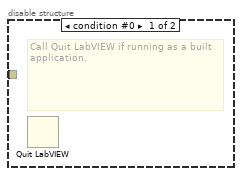
[diagram p4: hidden frame]
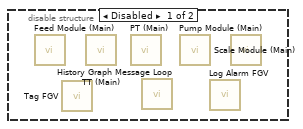
[diagram p5: hidden frame]
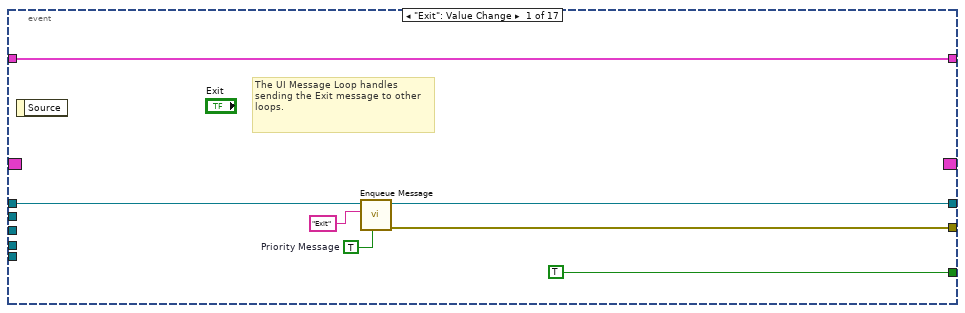
[diagram p6: hidden frame]
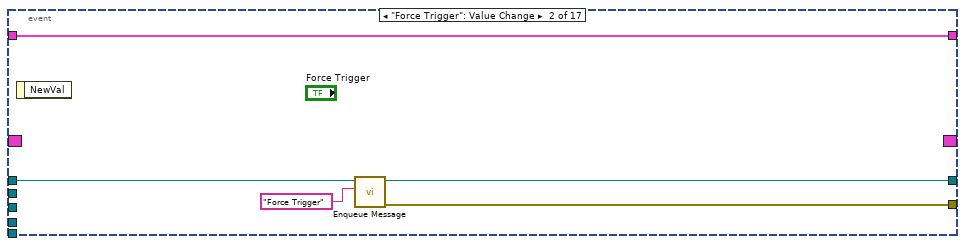
[diagram p7: hidden frame]
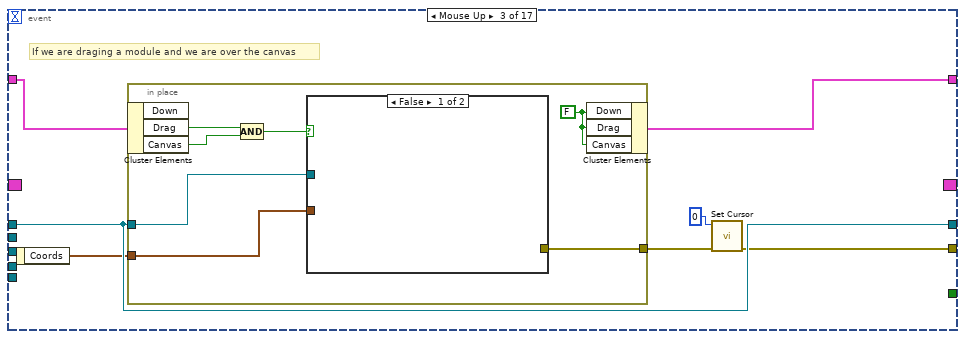
[diagram p8: hidden frame]
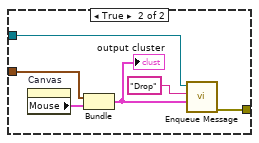
[diagram p9: hidden frame]
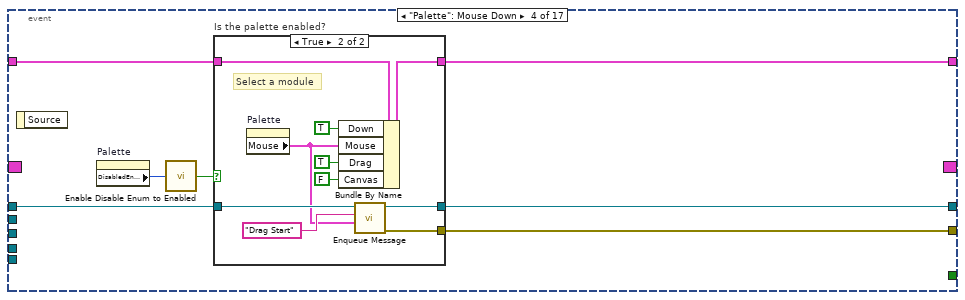
[diagram p10: hidden frame]
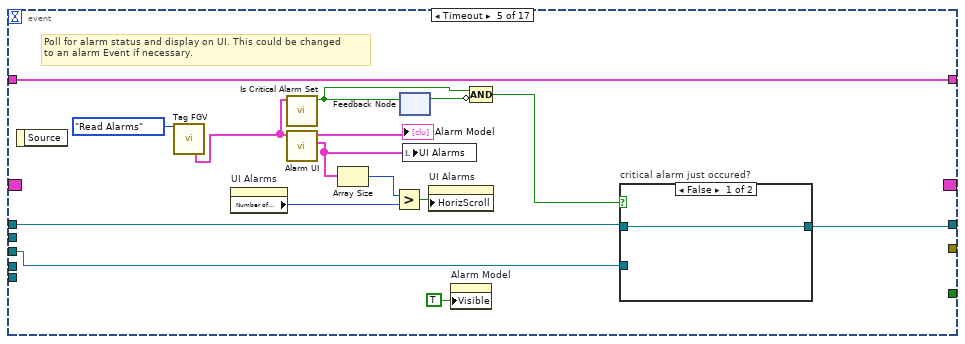
[diagram p12: hidden frame]
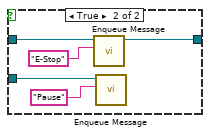
[diagram p13: hidden frame]
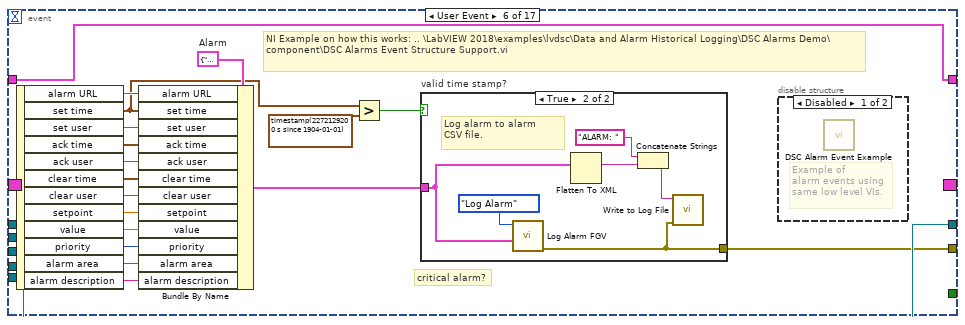
[diagram p14: hidden frame]
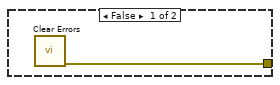
[diagram p16: hidden frame]
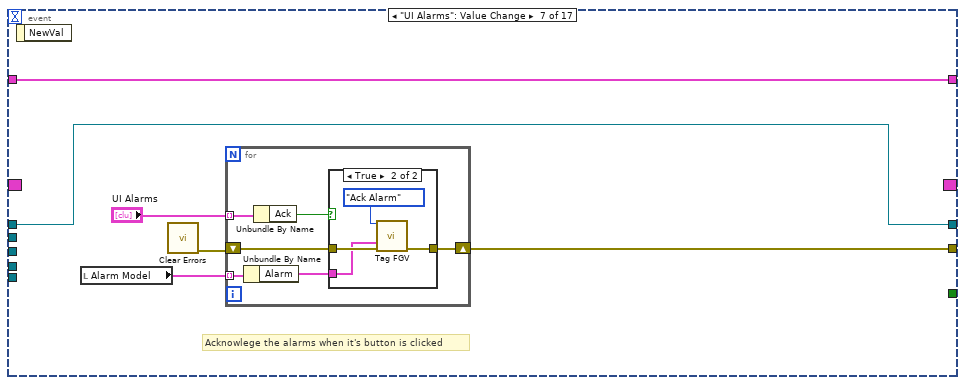
[diagram p17: hidden frame]
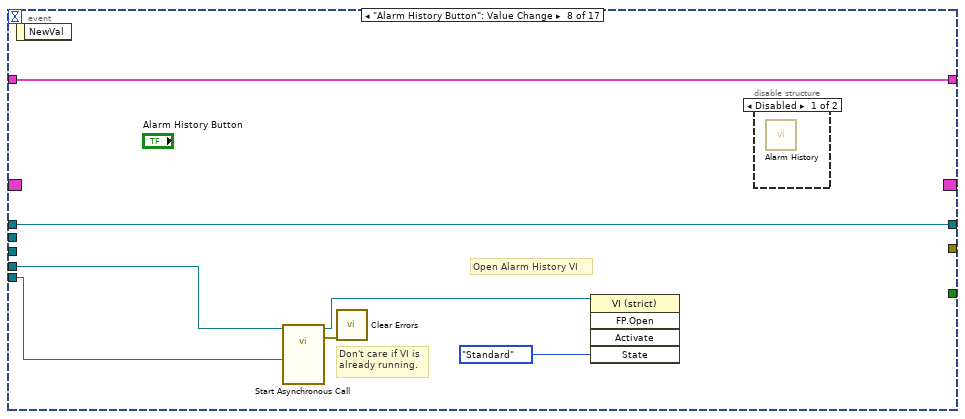
[diagram p19: hidden frame]
diagram:
  w50 = ""  # Event
  w57 = ""  # Event
  w80 = "Main" ("Process Name")
  # "<Event Registration Refnum.alarm & event notification>: User Event"
  # "9. This loop handels sequencing for scheduling start-up and shut-down"
  # "6. When a user drags and drops a module, such as TT, the user can click on the TT icon to configure which tags they display. They may also be able to configure alarms for\nthe tags. In the TT module, the alarms are configured in the \"Broadcast Settings\" case of the TT (Main).vi.\nCAVEAT: If a user configures more than one module to the same tag then the alarm thresholds may conflict with each other and one alarm\nthreshold will likely override the other."
  # "8. Alarms are handled by the functionality in the DSC. The alarm event is registered in the event structure and handled by the <Event Registration Refnum.alarm & event notification>: User Event.\n\nThat event calls Dynamic Shared Variables.lvlib:Log Alarm FGV.vi to log the alarm to a separate CSV file dedicated to alarms."
  # "Graph on the bottom of the main window is loaded dynamically in a subpanel because later we anticipate that a 2nd graph will be displayed\nnext to it."
  # "7. When the user presses the \"Start Log\" button, the tag values are logged into the CSV file. Path is determined in \"Start Log\" case above."
  # "5. The LabVIEW developer sets up DAQ Virtual Tasks in MAX, which would be configured for all the DAQ channels necessary for a campaign. When the user configures a campaign document, the user selects one of these DAQ Virtual Tasks from the application menubar DAQ->Settings.\nThe DAQ Message Loop.vi will create new shared variables for each of the DAQ measurements in the Commit DAQ Tags.vi."
  # "4. Each time the operator sets up a campaign \"Document\", a new shared variable process is created named Pfizer_FAST_<time stamp>.\nThe process is viewable in the NI Distributed System Manager. The process is created each time the Tag FGV.vi is called with the \"Init\" operation,\nwhich is called in the \"New Document\" case above."
  # "3. Each module creates \"tags\" which are handled by the Tag FGV. The Tag FGV creates shared variables for each tag. The dynamic shared variables\nmeans that this application requires the use of the DSC (Datalogging & Supervisory Control module)."
  # "2. The dynamic modules are shown in the disable structure."
  # "1. User can drag and drop dynamically launched modules. These are launched in the \"Drop\" case above."
  # "Set up to generate alarm events in\nevent structure."
  # "Don't care if VI\nis already closed"
  # "DAQ"
  # "UI"
  n1 = flat-sequence {
    tunnel: [w91] -> w39
    tunnel: ["?"] -> w40
    frame #0 {
      w89 = "Set Data Rate" ("item tag")
      n2 = control-ref of="?"() -> (w93:refnum<vi>)
      n3 = invoke class="Clust (strict)" method="Reinit To Default"(reference=w93) -> ()  [unwired: 2 in, 3 out]
      n4 = Current VI's Menubar() -> (w90:refnum<k9>)
      n5 = shared-variable ".\\Support Library.lvlib\\Globals.lvlib\\ASIA Pump Global"(T77 [{"Busy"=FALSE, "PumpCnt"=0.0, "RemoteEntered"=FALSE, "OverpressureSet"=FALSE}, {"Busy"=FALSE, "PumpCnt"=0.0, "RemoteEntered"=FALSE, "OverpressureSet"=FALSE}, {"Busy"=FALSE, "PumpCnt"=0.0, "RemoteEntered"=FALSE, "OverpressureSet"=FALSE}, {"Busy"=FALSE, "PumpCnt"=0.0, "RemoteEntered"=FALSE, "OverpressureSet"=FALSE}, {"Busy"=FALSE, "PumpCnt"=0.0, "RemoteEntered"=FALSE, "OverpressureSet"=FALSE}, {"Busy"=FALSE, "PumpCnt"=0.0, "RemoteEntered"=FALSE, "OverpressureSet"=FALSE}, {"Busy"=FALSE, "PumpCnt"=0.0, "RemoteEntered"=FALSE, "OverpressureSet"=FALSE}, {"Busy"=FALSE, "PumpCnt"=0.0, "RemoteEntered"=FALSE, "OverpressureSet"=FALSE}, {"Busy"=FALSE, "PumpCnt"=0.0, "RemoteEntered"=FALSE, "OverpressureSet"=FALSE}, {"Busy"=FALSE, "PumpCnt"=0.0, "RemoteEntered"=FALSE, "OverpressureSet"=FALSE}, {"Busy"=FALSE, "PumpCnt"=0.0, "RemoteEntered"=FALSE, "OverpressureSet"=FALSE}] ("ASIA Pump Global")) -> ()  [unwired: 1 in, 1 out]
      n6 = invoke class="Clust (strict)" method="Reinit To Default"() -> (error out=w91:errorcluster)  [unwired: 3 in, 2 out]
      n7 = Set Menu Item Info(7:w89, 9:TRUE ("enabled"), 10:w89, 11:w90) -> ()  [unwired: 3 in, 2 out]
    }
    frame #1 {
      n8 = disable-structure shown="Enabled" {
        frame Disabled {
          n9 = property on="Start Log" class="Bool"("Value"=FALSE) -> ()  [unwired: 2 in, 2 out]
        }
        frame Enabled {
        }
      }
    }
  }
  n10 = vi-ref "Dynamic Shared Variables.lvlib:Alarm History.vi"() -> (w61:refnum<vi>)
  n11 = call <vilib>:"Enable Alarm & Event Notifications.vi"() -> ("error out"=w44:errorcluster, "alarm & event notification"=w45:refnum<user-event>)  [unwired: 10 in]
  n12 = property class="VI"(reference=w61) -> ("Path"=w62:path)  [unwired: 1 in, 2 out]
  n13 = call "Create File.vi"("error in"=w39) -> ("error out"=w37:errorcluster)  [unwired: 10 in]
  n14 = Open VI Reference(type specifier VI Refnum (for type only)=refnum<vi> refnum, vi path=w62, options=128) -> (vi reference=w52:refnum<vi>, error out=w58:errorcluster)  [unwired: 3 in]
  n15 = register-events(error in=w44, w45) -> (reference out=w49:refnum<event-registration>, error out=w43:errorcluster)  [unwired: 1 in]
  n16 = call "Create User Event - Stop.vi"("error in (no error)"=w39) -> ("User Event - Stop"=w84:refnum<user-event>, "Stop Event Registration Refnum"=w48:refnum<event-registration>)  [unwired: 8 in, 1 out]
  n17 = call "Create Main Message Queues.vi"("error in (no error)"=w37, "Process Name"=w80) -> ("error out"=w81:errorcluster, "Message Queues out"=w29:T78)  [unwired: 8 in]
  n18 = Create User Event(user event datatype=w57, error in=w58) -> (user event=w51:refnum<user-event>)  [unwired: 1 out]
  n19 = Unbundle By Name(w29) -> ("UI"=w82:refnum<queue>, "DAQ"=w64:refnum<queue>, "Sequence"=w42:refnum<queue>, "CSV Log"=w41:refnum<queue>, "Sequence UI"=w31:refnum<queue>, "OPC UA Log"=w30:refnum<queue>, "Waveform Loop"=w24:refnum<queue>, "TDMS Log"=w23:refnum<queue>, "Graphs"=w22:refnum<queue>[], "TCP Write"=w21:refnum<queue>, "TCP Read"=w20:refnum<queue>, "OPC UA Log"=w19:refnum<queue>)
  n20 = call "Tag FGV.vi"("Operation"=Tag_FGV_Operation_Enum."Set Notification Queue", "Data"=w45, "error in (no error)"=w43) -> ()  [unwired: 5 in, 8 out]
  n21 = Current VI's Path() -> (path=w78:path)
  n22 = Bundle("Event Registration Refnum"=w49, "Stop Event Registration Refnum"=w48) -> (w47:T79)  [unwired: 1 in]
  n23 = Strip Path(path=w78) -> (stripped path=w68:path)  [unwired: 1 out]
  n24 = Build Path(base path=w68, name or relative path="History Graph") -> (appended path=w66:path)
  n25 = disable-structure shown="Enabled" {
    disable-tunnel: w29 -> [w96 w97]
    frame Disabled {
      n26 = call "OSIPI OPCUA Server.vi"("Main Queue Cluster"=w96) -> ()  [unwired: 11 in]
    }
    frame Enabled {
      n27 = call "OSIPI OPCUA Server Tag Version.vi"("Main Queue Cluster"=w97) -> ()  [unwired: 11 in]
    }
  }
  n28 = call "Sequence.vi"("Message Queues in"=w29) -> ("error out"=w32:errorcluster)  [unwired: 10 in]
  n29 = call "Waveform Loop.vi"("Message Queues out"=w29) -> ("error out"=w36:errorcluster)  [unwired: 10 in]
  n30 = call "TCP Write.vi"("Message Queues out"=w29) -> ()  [unwired: 11 in]
  n31 = call "TDMS Log Loop.vi"("Message Queues"=w29) -> ("error out"=w35:errorcluster)  [unwired: 10 in]
  n32 = call "DAQ Message Loop.vi"("Message Queues"=w29) -> ("error out"=w34:errorcluster)  [unwired: 10 in]
  n33 = call "CSV Log Loop.vi"("Message Queues"=w29) -> ("error out"=w33:errorcluster)  [unwired: 10 in]
  n34 = while {
    tunnel: w82 -> [w118]
    tunnel: w84 -> [w123]
    shift-right: [w116] -> w87
    shift-left: w81 -> [w122]
    tunnel: w80 -> [w114]
    tunnel: w29 -> [w113]
    shift-right: [w111] -> _
    shift-left: w40 -> [w112]
    tunnel: w29 -> [w110]
    tunnel: w64 -> [w107]
    tunnel: w42 -> [w106]
    tunnel: w41 -> [w104]
    tunnel: w31 -> [w108]
    tunnel: w30 -> [w105]
    tunnel: [w109] -> w28
    tunnel: [w107] -> w27
    tunnel: [w105] -> w26
    tunnel: [w104] -> w25
    tunnel: w24 -> [w103]
    tunnel: w23 -> [w102]
    tunnel: w22 -> [w101]
    tunnel: w21 -> [w100]
    tunnel: w20 -> [w99]
    tunnel: w19 -> [w98]
    tunnel: [w103] -> w18
    tunnel: [w102] -> w17
    tunnel: [w101] -> w16
    tunnel: [w100] -> w15
    tunnel: [w99] -> w14
    tunnel: [w98] -> w13
    stop <- w124 stop-if-true
    # "UI Message Loop"
    n35 = call "Dequeue Message.vi"("error in (no error)"=w122, "Message Queue"=w118) -> ("error out"=w121:errorcluster, "Message Data"=w119:variant, "Message"=w120:string, "dup Message Queue"=w115:refnum<queue>)  [unwired: 6 in]
    n36 = case "Message Cases" shown="\"Commit Config (TT)\"" w120 {
      selector: w120 -> [_ _ _ _ _ _ _ _ _ _ _ _ _ _ _ _ _ _ _ _ _ _ _ _ _ _ _ _ _ _ _ _ _ _ _ _ _ _ _ _ w1269 _ _ _ _ _ _ _ _ _ w1483 _]
      tunnel: w115 -> [_ _ _ _ _ _ _ _ _ _ _ _ _ _ _ _ w694 w718 w742 w766 w790 w814 w838 w862 w886 w910 w934 w958 _ _ w1020 _ w1085 _ _ w1155 _ w1202 w1249 _ _ w1309 _ _ _ _ _ _ _ _ _ _]
      tunnel: w121 -> [w127 w135 w154 w199 w244 w289 w331 w374 w417 w460 w502 w545 w588 w632 w676 w686 w693 w717 w741 w765 w789 w813 w837 w861 w885 w909 w933 w957 w981 w1012 w1027 w1068 _ w1107 w1142 w1154 w1191 w1215 _ w1259 w1275 w1312 w1390 w1396 w1408 w1440 w1444 w1449 w1474 w1480 _ w1492]
      tunnel: [w126 w128 w146 w191 w236 w281 w326 w369 w412 w455 w498 w541 w584 w628 w670 w684 w691 w715 w739 w763 w787 w811 w835 w859 w883 w907 w931 w955 w979 w998 w1019 w1066 w1077 w1099 w1138 w1146 w1185 w1200 w1245 w1254 w1263 w1303 w1382 w1396 w1398 w1439 w1443 w1447 w1472 w1476 w1482 w1492] -> w117
      tunnel: [_ _ _ _ _ _ _ _ _ _ _ _ _ _ _ _ _ _ _ _ _ _ _ _ _ _ _ _ _ _ _ FALSE _ TRUE _ _ _ _ _ _ _ _ _ _ _ _ _ _ _ _ _ _] -> w124
      tunnel: w119 -> [_ w136 w155 w200 w245 w290 w332 w375 w418 w461 w503 w546 w589 w633 w677 _ _ _ _ _ _ _ _ _ _ _ _ _ _ w1011 w1029 _ w1087 _ _ _ _ _ _ _ _ _ _ _ _ _ _ _ _ _ _ _]
      tunnel: w123 -> [_ _ _ _ _ _ _ _ _ _ _ _ _ _ _ _ _ _ _ _ _ _ _ _ _ _ _ _ _ _ _ _ _ w1123 _ _ _ _ _ _ _ _ _ _ _ _ _ _ _ _ _ _]
      tunnel: w114 -> [_ _ _ _ _ _ _ _ _ _ _ _ _ _ _ _ _ _ _ _ _ _ _ _ _ _ _ _ _ _ _ _ _ _ _ _ _ _ _ _ _ _ _ _ _ _ _ _ _ _ _ _]
      tunnel: w113 -> [_ _ _ _ _ _ _ _ _ _ _ _ _ _ _ _ _ _ _ _ _ _ _ _ _ _ _ _ _ _ _ _ _ _ _ _ _ _ _ _ _ _ _ _ _ _ _ _ _ _ _ _]
      tunnel: w112 -> [w125 w133 w145 w190 w235 w280 w325 w368 w411 w454 w497 w540 w583 w627 w669 w688 w697 w721 w745 w769 w793 w817 w841 w865 w889 w913 w937 w961 w982 w1003 w1026 w1071 w1083 w1111 w1141 w1143 w1199 w1205 w1248 w1257 w1262 w1301 w1391 w1395 w1401 w1437 w1442 w1455 w1471 w1479 w1491 w1494]
      tunnel: [w125 w134 w144 w189 w234 w279 w324 w367 w410 w453 w496 w539 w582 w626 w668 w688 w698 w722 w746 w770 w794 w818 w842 w866 w890 w914 w938 w962 w982 w1004 w1014 w1070 w1083 w1093 w1137 w1177 w1199 w1206 w1248 w1258 w1270 w1301 w1391 w1395 w1405 w1438 w1442 w1455 w1471 w1479 w1491 w1494] -> w111
      tunnel: w110 -> [_ _ _ _ _ _ _ _ _ _ _ _ _ _ _ _ _ _ _ _ _ _ _ _ _ _ _ _ _ _ _ _ _ w1122 _ _ _ _ _ _ _ w1315 w1393 _ _ _ w1445 _ _ _ _ _]
      tunnel: w107 -> [_ _ _ _ _ _ _ _ _ _ _ _ _ _ _ w689 _ _ _ _ _ _ _ _ _ _ _ _ _ _ _ _ _ _ _ _ w1195 w1201 _ _ _ _ _ _ _ _ _ _ _ _ _ _]
      tunnel: w106 -> [_ _ _ _ _ _ _ _ _ _ _ _ _ _ _ _ _ _ _ _ _ _ _ _ _ _ _ _ _ _ _ _ _ _ _ _ _ _ _ _ _ _ _ _ w1403 _ _ _ _ _ _ _]
      tunnel: w104 -> [_ _ _ _ _ _ _ _ _ _ _ _ _ _ _ _ _ _ _ _ _ _ _ _ _ _ _ _ _ _ _ _ _ _ _ _ _ _ _ _ _ w1308 _ _ _ _ _ _ _ w1481 _ _]
      tunnel: w108 -> [_ _ _ _ _ _ _ _ _ _ _ _ _ _ _ _ _ _ _ _ _ _ _ _ _ _ _ _ _ _ _ _ _ _ _ _ _ _ _ _ _ _ _ _ w1397 _ _ _ _ _ _ _]
      tunnel: w105 -> [_ _ _ _ _ _ _ _ _ _ _ _ _ _ _ _ _ _ _ _ _ _ _ _ _ _ _ _ _ _ _ _ _ _ _ _ _ _ _ _ _ w1302 _ _ _ _ _ _ _ _ _ _]
      frame "---Copy This Frame---" {
        # "Duplicate this frame when creating new messages.  Change this comment in the duplicated frame to describe this message."
        n37 = Merge Errors(w127) -> (w126:errorcluster)
      }
      frame "Commit Config (DAQ)" {
        # "Save DAQ Settings"
        n38 = Unbundle By Name(w133) -> ("Main Config.DAQ Config"=w132:T39)
        n39 = Variant To Data(error in=w135, type=w132, Variant=w136) -> (data=w130:T39, error out=w131:errorcluster)
        n40 = case shown="No Error" w131 {
          selector: w131 -> [w137 w142]
          tunnel: [w141 w143] -> w134
          tunnel: w133 -> [w140 w143]
          tunnel: w130 -> [w139 _]
          tunnel: [w137 w142] -> w128
          frame No Error {
            n41 = Bundle By Name(cluster=w140, "Main Config.DAQ Config"=w139, "Config Changed?"=TRUE) -> (w141:T1)
          }
          frame Error {
          }
        }
        n42 = call "Write to Log File.vi"("error in"=w128, "text"="Main: Commit Config (DAQ)") -> ()  [unwired: 9 in, 1 out]
      }
      frame "Commit Config (Feed Module)" {
        # "Save Feed Module Settings"
        n43 = Variant To Data(error in=w154, type=T18 {"GUID"="", "Drop Coords"={"Horizontal"=0, "Vertical"=0}, "Process Name"="", "Queue Name"="", "Settings"={"Cycle Period"=500.0, "Ismatech"={"VISA resource name"="", "Simulated?"=TRUE, "Pump Number"=1.0, "Reverse?"=FALSE}, "Masterflex"={"VISA resource name"="", "Simulated?"=TRUE, "Pump Number"=1.0, "Reverse?"=FALSE}, "Mettler"={"VISA resource name"="", "Simulated?"=FALSE}, "Bronkhorst M13 Flow Meter"={"VISA resource name"="", "Simulated?"=TRUE, "Smoothing Steps"=1}, "PID 2 Parameters"={"Input Device"=enum."Default", "Output Device"=enum."Default", "Setpoint"=0.0, "PID gains"={"proportional gain (Kc)"=1.0, "integral time (Ti, min)"=0.01, "derivative time (Td, min)"=0.0}}, "Manual Entry"=0.0, "Auto?"=TRUE, "output range"={"output high"=100.0, "output low"=0.0}, "Tacmina Settings"={"Analog DAQ Task"="", "Digital DAQ Task"=""}, "KNF SIMDOS Settings"={"VISA resource name"="", "Simulated?"=TRUE}, "ASIA Pump C"={"ASIA Pump #"=0, "channel"=0, "Simulated"=FALSE}, "VICI Settings"={"VISA resource name"="", "Simulated?"=TRUE, "Pump Letter"="", "Reverse?"=FALSE}, "FLOM Settings"={"VISA resource name"="", "Simulated?"=TRUE, "Pump Number"=0.0}, "SSI PR/LD Settings"={"VISA resource name"="", "Simulated?"=FALSE}, "Masterflex 75211 Settings"={"Analog DAQ Task"="", "Digital DAQ Task"=""}, "SSI P40 Settings"={"VISA resource name"="", "Simulated?"=TRUE}, "Ismatech 3 Channel Settings"={"VISA resource name"="", "Pump Number"=1, "Channel Number"=0, "Simulated?"=TRUE, "Reverse?"=FALSE}, "Bronkhorst M14 Settings"={"VISA resource name"="", "Simulated?"=FALSE, "Smoothing Steps"=1}}, "Settings Load Count"=0, "OP Load Count"=0} ("Feed Module Config"), Variant=w155) -> (data=w153:T18, error out=w149:errorcluster)
        n44 = Unbundle By Name(w153) -> ("GUID"=w150:string)
        n45 = Format Into String(format string="Could not save Feed Module config. No matching GUID for \"%s\"." ("error message (\"\")"), w150) -> (resulting string=w151:string)  [unwired: 2 in, 1 out]
        n46 = in-place {
          in-place-border: w153 -> [w162]
          in-place-border: w151 -> [w161]
          in-place-border: w150 -> [w160]
          in-place-border: w149 -> [w159]
          in-place-border: [w158] -> w146
          n47 = in-place-cluster #1(w145) -> ("Main Config.Feed Module Configs"=w157:T18[])
          n48 = Empty Array?(array=w157) -> (empty?=w163:bool)
          n49 = case shown="True" w163 {
            tunnel: w160 -> [w171 _]
            tunnel: w157 -> [w169 w188]
            tunnel: w162 -> [w168 w187]
            tunnel: [w167 w186] -> w156
            tunnel: w161 -> [w166 _]
            tunnel: w159 -> [w165 w185]
            tunnel: [w164 w185] -> w158
            frame False {
              n50 = for {
                tunnel: w169 -> [w184] mode=indexing
                tunnel: [w183] -> w172 mode=indexing
                workers-P: _ -> [_]
                n51 = Unbundle By Name(w184) -> ("GUID"=w183:string)
              }
              n52 = Search 1D Array(1D array=w172, element=w171) -> (index of element=w170:i32)  [unwired: 1 in]
              n53 = case shown="0, Default" w170 {
                selector: w170 -> [w176 _]
                tunnel: w169 -> [w177 w182]
                tunnel: w168 -> [w175 _]
                tunnel: [w174 w182] -> w167
                tunnel: w166 -> [_ w180]
                tunnel: w165 -> [w173 w179]
                tunnel: [w173 w178] -> w164
                frame 0, Default {
                  n54 = Replace Array Subset(array=w177, new element=w175, index=w176) -> (w174:T18[])
                }
                frame -1 {
                  n55 = call <vilib>:"Error Cluster From Error Code.vi"("error in (no error)"=w179, "error message (\"\")"=w180, "error code (0)"=7004) -> ("error out"=w178:errorcluster)  [unwired: 6 in]
                }
              }
            }
            frame True {
              n56 = Build Array (concatenate)(w188, w187) -> (w186:T18[])
            }
          }
          n57 = in-place-cluster #1("Main Config.Feed Module Configs"=w156) -> (w144:T1)
        }
        n58 = call "Write to Log File.vi"("error in"=w146, "text"="Main: Commit Config (Feed Module)") -> ()  [unwired: 9 in, 1 out]
      }
      frame "Commit Config (OPC Module)" {
        # "Save Feed Module Settings"
        n59 = Variant To Data(error in=w199, type=T8 {"State"=enum."Idle", "GUID"="", "Drop Coords"={"Horizontal"=0, "Vertical"=0}, "Configuration"={"Cycle Period"=500.0, "server endpoint URL"="opc.tcp://10.131.1.22:4840", "security policy"={"message mode"=enum."Sign", "security"=enum."Basic256"}, "Trust Any Server"=FALSE}, "First Iteration"=FALSE, "Data"=[], "Process Name"="", "Load Count"=0, "Log Started"=FALSE, "subscription ID out"=0, "OPC UA client refnum out"="", "Event Registration Refnum"=refnum, "Start Time"=timestamp(0 s since 1904-01-01), "Current Time"=timestamp(0 s since 1904-01-01), "Tag Data"=[]} ("OPC Module Config"), Variant=w200) -> (data=w198:T8, error out=w194:errorcluster)
        n60 = Unbundle By Name(w198) -> ("GUID"=w195:string)
        n61 = Format Into String(format string="Could not save OPCUA Module config. No matching GUID for \"%s\"." ("error message (\"\")"), w195) -> (resulting string=w196:string)  [unwired: 2 in, 1 out]
        n62 = in-place {
          in-place-border: w198 -> [w207]
          in-place-border: w196 -> [w206]
          in-place-border: w195 -> [w205]
          in-place-border: w194 -> [w204]
          in-place-border: [w203] -> w191
          n63 = in-place-cluster #2(w190) -> ("Main Config.OPC Module Configs"=w202:T8[])
          n64 = Empty Array?(array=w202) -> (empty?=w208:bool)
          n65 = case shown="False" w208 {
            tunnel: w205 -> [w216 _]
            tunnel: w202 -> [w214 w233]
            tunnel: w207 -> [w213 w232]
            tunnel: [w212 w231] -> w201
            tunnel: w206 -> [w211 _]
            tunnel: w204 -> [w210 w230]
            tunnel: [w209 w230] -> w203
            frame False {
              n66 = for {
                tunnel: w214 -> [w229] mode=indexing
                tunnel: [w228] -> w217 mode=indexing
                workers-P: _ -> [_]
                n67 = Unbundle By Name(w229) -> ("GUID"=w228:string)
              }
              n68 = Search 1D Array(1D array=w217, element=w216) -> (index of element=w215:i32)  [unwired: 1 in]
              n69 = case shown="0, Default" w215 {
                selector: w215 -> [w221 _]
                tunnel: w214 -> [w222 w227]
                tunnel: w213 -> [w220 _]
                tunnel: [w219 w227] -> w212
                tunnel: w211 -> [_ w225]
                tunnel: w210 -> [w218 w224]
                tunnel: [w218 w223] -> w209
                frame 0, Default {
                  n70 = Replace Array Subset(array=w222, new element=w220, index=w221) -> (w219:T8[])
                }
                frame -1 {
                  n71 = call <vilib>:"Error Cluster From Error Code.vi"("error in (no error)"=w224, "error message (\"\")"=w225, "error code (0)"=7004) -> ("error out"=w223:errorcluster)  [unwired: 6 in]
                }
              }
            }
            frame True {
              n72 = Build Array (concatenate)(w233, w232) -> (w231:T8[])
            }
          }
          n73 = in-place-cluster #2("Main Config.OPC Module Configs"=w201) -> (w189:T1)
        }
        n74 = call "Write to Log File.vi"("error in"=w191, "text"="Main: Commit Config (Feed Module)") -> ()  [unwired: 9 in, 1 out]
      }
      frame "Commit Config (Pump Module)" {
        # "Save Pump Module Settings"
        n75 = Variant To Data(error in=w244, type=T44 {"GUID"="", "Drop Coords"={"Horizontal"=0, "Vertical"=0}, "Process Name"="", "Queue Name"="", "Settings"={"Cycle Period"=500.0, "Manual Entry"=0.0, "Output Device"=enum."Default", "Ismatech"={"VISA resource name"="", "Simulated?"=TRUE, "Pump Number"=1.0, "Reverse?"=FALSE}, "Ismatech 3 Channel Settings"={"VISA resource name"="", "Pump Number"=1, "Channel Number"=0, "Simulated?"=TRUE, "Reverse?"=FALSE}, "Masterflex"={"VISA resource name"="", "Simulated?"=TRUE, "Pump Number"=1.0, "Reverse?"=FALSE}, "VICI Settings"={"VISA resource name"="", "Simulated?"=TRUE, "Pump Letter"="", "Reverse?"=FALSE}, "Tacmina Settings"={"Analog DAQ Task"="", "Digital DAQ Task"=""}, "KNF SIMDOS Settings"={"VISA resource name"="", "Simulated?"=TRUE}, "ASIA Pump C"={"ASIA Pump #"=0, "channel"=0, "Simulated"=FALSE}, "FLOM Settings"={"VISA resource name"="", "Simulated?"=TRUE, "Pump Number"=0.0}, "SSI PR/LD Settings"={"VISA resource name"="", "Simulated?"=FALSE}, "SSI P40 Settings"={"VISA resource name"="", "Simulated?"=FALSE}, "Masterflex 75211 Settings"={"Analog DAQ Task"="", "Digital DAQ Task"=""}, "Pump Calibration File"=path "", "Calibration Slope"=0.0, "Calibration Y Intercept"=0.0, "Pump Cal Enum"=0}, "Load Count"=0} ("Pump Module Config"), Variant=w245) -> (data=w238:T44, error out=w240:errorcluster)
        n76 = Unbundle By Name(w238) -> ("GUID"=w241:string)
        n77 = Format Into String(format string="Could not save Pump Module config. No matching GUID for \"%s\"." ("error message (\"\")"), w241) -> (resulting string=w242:string)  [unwired: 2 in, 1 out]
        n78 = in-place {
          in-place-border: w242 -> [w252]
          in-place-border: w241 -> [w251]
          in-place-border: w240 -> [w250]
          in-place-border: w238 -> [w249]
          in-place-border: [w248] -> w236
          n79 = in-place-cluster #3(w235) -> ("Main Config.Pump Module Configs"=w247:T44[])
          n80 = Empty Array?(array=w247) -> (empty?=w253:bool)
          n81 = case shown="True" w253 {
            tunnel: w251 -> [w261 _]
            tunnel: w247 -> [w259 w278]
            tunnel: w249 -> [w258 w275]
            tunnel: [w257 w277] -> w246
            tunnel: w252 -> [w256 _]
            tunnel: w250 -> [w255 w276]
            tunnel: [w254 w276] -> w248
            frame False {
              n82 = for {
                tunnel: w259 -> [w274] mode=indexing
                tunnel: [w273] -> w262 mode=indexing
                workers-P: _ -> [_]
                n83 = Unbundle By Name(w274) -> ("GUID"=w273:string)
              }
              n84 = Search 1D Array(1D array=w262, element=w261) -> (index of element=w260:i32)  [unwired: 1 in]
              n85 = case shown="0, Default" w260 {
                selector: w260 -> [w266 _]
                tunnel: w259 -> [w267 w272]
                tunnel: w258 -> [w263 _]
                tunnel: [w265 w272] -> w257
                tunnel: w256 -> [_ w270]
                tunnel: w255 -> [w264 w269]
                tunnel: [w264 w268] -> w254
                frame 0, Default {
                  n86 = Replace Array Subset(array=w267, new element=w263, index=w266) -> (w265:T44[])
                }
                frame -1 {
                  n87 = call <vilib>:"Error Cluster From Error Code.vi"("error in (no error)"=w269, "error message (\"\")"=w270, "error code (0)"=7004) -> ("error out"=w268:errorcluster)  [unwired: 6 in]
                }
              }
            }
            frame True {
              n88 = Build Array (concatenate)(w278, w275) -> (w277:T44[])
            }
          }
          n89 = in-place-cluster #3("Main Config.Pump Module Configs"=w246) -> (w234:T1)
        }
        n90 = call "Write to Log File.vi"("error in"=w236, "text"="Main: Commit Config (Pump Module)") -> ()  [unwired: 9 in, 1 out]
      }
      frame "Commit Config (DO)" {
        # "Save Digital Output Module Settings"
        n91 = Variant To Data(error in=w289, type=T59 {"GUID"="", "Drop Coords"={"Horizontal"=0, "Vertical"=0}, "Process Name"="", "Queue Name"="", "Settings"={"Valve Settings"={"D-O Settings"={"DAQmx Task Name"="", "Output Channel"=0, "Output Channel Names"=[]}, "VICI Electronic Actuator"={"VISA resource name"="", "Mode"=enum."Two Positions With Stops", "Simulated"=FALSE}}, "Valve Type"=enum."Default", "Time On (Sec)"=0.0, "Time Off (Sec)"=0.0, "Run?"=FALSE}, "Load Count"=0} ("D-O Module Config"), Variant=w290) -> (data=w288:T59, error out=w284:errorcluster)
        n92 = Unbundle By Name(w288) -> ("GUID"=w285:string)
        n93 = Format Into String(format string="Could not save Digital Out Module config. No matching GUID for \"%s\"." ("error message (\"\")"), w285) -> (resulting string=w286:string)  [unwired: 2 in, 1 out]
        n94 = in-place {
          in-place-border: w288 -> [w297]
          in-place-border: w286 -> [w296]
          in-place-border: w285 -> [w295]
          in-place-border: w284 -> [w294]
          in-place-border: [w293] -> w281
          n95 = in-place-cluster #4(w280) -> ("Main Config.DO Module Configs"=w292:T59[])
          n96 = Empty Array?(array=w292) -> (empty?=w298:bool)
          n97 = case shown="False" w298 {
            tunnel: w295 -> [w306 _]
            tunnel: w292 -> [w304 w323]
            tunnel: w297 -> [w303 w322]
            tunnel: [w302 w321] -> w291
            tunnel: w296 -> [w301 _]
            tunnel: w294 -> [w300 w320]
            tunnel: [w299 w320] -> w293
            frame False {
              n98 = for {
                tunnel: w304 -> [w319] mode=indexing
                tunnel: [w318] -> w307 mode=indexing
                workers-P: _ -> [_]
                n99 = Unbundle By Name(w319) -> ("GUID"=w318:string)
              }
              n100 = Search 1D Array(1D array=w307, element=w306) -> (index of element=w305:i32)  [unwired: 1 in]
              n101 = case shown="0, Default" w305 {
                selector: w305 -> [w311 _]
                tunnel: w304 -> [w312 w317]
                tunnel: w303 -> [w310 _]
                tunnel: [w309 w317] -> w302
                tunnel: w301 -> [_ w315]
                tunnel: w300 -> [w308 w314]
                tunnel: [w308 w313] -> w299
                frame 0, Default {
                  n102 = Replace Array Subset(array=w312, new element=w310, index=w311) -> (w309:T59[])
                }
                frame -1 {
                  n103 = call <vilib>:"Error Cluster From Error Code.vi"("error in (no error)"=w314, "error message (\"\")"=w315, "error code (0)"=7004) -> ("error out"=w313:errorcluster)  [unwired: 6 in]
                }
              }
            }
            frame True {
              n104 = Build Array (concatenate)(w323, w322) -> (w321:T59[])
            }
          }
          n105 = in-place-cluster #4("Main Config.DO Module Configs"=w291) -> (w279:T1)
        }
        n106 = call "Write to Log File.vi"("error in"=w281, "text"="Main: Commit Config (DO)") -> ()  [unwired: 9 in, 1 out]
      }
      frame "Commit Config (PR Module)" {
        # "Save Pressure Regulator Module Settings"
        n107 = Variant To Data(error in=w331, type=T64 {"GUID"="", "Drop Coords"={"Horizontal"=0, "Vertical"=0}, "Process Name"="", "Queue Name"="", "Settings"={"Cycle Period"=500.0, "PID 2 Parameters"={"Input Device"=enum."Default", "Output Device"=enum."Default", "Setpoint"=0.0, "PID gains"={"proportional gain (Kc)"=1.0, "integral time (Ti, min)"=0.01, "derivative time (Td, min)"=0.0}, "output range"={"output low"=0.0, "output high"=100.0}}, "Manual Entry"=0.0, "Auto?"=TRUE, "4-20mA Input Settings"={"Input Channel "=0}, "4-20mA Out Settings"={"Output DAQ Task"=""}, "Input Channel Tag Name "=""}, "Settings Load Count"=0} ("Feed Module Config"), Variant=w332) -> (data=w330:T64, error out=w329:errorcluster)
        n108 = in-place {
          in-place-border: w330 -> [w340]
          in-place-border: w329 -> [w336]
          in-place-border: [w335] -> w326
          n109 = in-place-cluster #5(w325) -> ("Main Config.PR Module Configs"=w334:T64[])
          n110 = Unbundle By Name(w340) -> ("GUID"=w337:string)
          n111 = Empty Array?(array=w334) -> (empty?=w341:bool)
          n112 = Format Into String(format string="Could not save Digital Out Module config. No matching GUID for \"%s\"." ("error message (\"\")"), w337) -> (resulting string=w338:string)  [unwired: 2 in, 1 out]
          n113 = case shown="True" w341 {
            tunnel: w337 -> [w349 _]
            tunnel: w334 -> [w347 w366]
            tunnel: w340 -> [w346 w363]
            tunnel: [w345 w365] -> w333
            tunnel: w338 -> [w344 _]
            tunnel: w336 -> [w343 w364]
            tunnel: [w342 w364] -> w335
            frame False {
              n114 = for {
                tunnel: w347 -> [w362] mode=indexing
                tunnel: [w361] -> w350 mode=indexing
                workers-P: _ -> [_]
                n115 = Unbundle By Name(w362) -> ("GUID"=w361:string)
              }
              n116 = Search 1D Array(1D array=w350, element=w349) -> (index of element=w348:i32)  [unwired: 1 in]
              n117 = case shown="-1" w348 {
                selector: w348 -> [w354 _]
                tunnel: w347 -> [w355 w360]
                tunnel: w346 -> [w353 _]
                tunnel: [w352 w360] -> w345
                tunnel: w344 -> [_ w358]
                tunnel: w343 -> [w351 w357]
                tunnel: [w351 w356] -> w342
                frame 0, Default {
                  n118 = Replace Array Subset(array=w355, new element=w353, index=w354) -> (w352:T64[])
                }
                frame -1 {
                  n119 = call <vilib>:"Error Cluster From Error Code.vi"("error in (no error)"=w357, "error message (\"\")"=w358, "error code (0)"=7004) -> ("error out"=w356:errorcluster)  [unwired: 6 in]
                }
              }
            }
            frame True {
              n120 = Build Array (concatenate)(w366, w363) -> (w365:T64[])
            }
          }
          n121 = in-place-cluster #5("Main Config.PR Module Configs"=w333) -> (w324:T1)
        }
        n122 = call "Write to Log File.vi"("error in"=w326, "text"="Main: Commit Config (PR Module)") -> ()  [unwired: 9 in, 1 out]
      }
      frame "Commit Config (TCU Module)" {
        # "Save Temperature Control Unit Module Settings"
        n123 = Variant To Data(error in=w374, type=T50 {"GUID"="", "Drop Coords"={"Horizontal"=0, "Vertical"=0}, "Process Name"="", "Queue Name"="", "Settings"={"Cycle Period"=500.0, "Setpoint Entry"=0.0, "Output Device"=enum."Default", "Huber Ministat 230 Settings"={"VISA resource name"="", "Simulated?"=FALSE}, "Lauda Settings"={"VISA resource name"="", "Simulated?"=FALSE, "Pump Power"=2}, "Julabo FP-50 Settings"={"VISA resource name"="", "Simulated?"=FALSE, "Pump Power"=2}, "Internal Control?"=FALSE, "Huber Unistat 410 Settings"={"VISA resource name"="", "Address"=0, "Simulated?"=FALSE}}, "Load Count"=0, "Power Level Changed"=FALSE} ("TCU Module Config"), Variant=w375) -> (data=w373:T50, error out=w372:errorcluster)
        n124 = in-place {
          in-place-border: w373 -> [w383]
          in-place-border: w372 -> [w379]
          in-place-border: [w378] -> w369
          n125 = in-place-cluster #6(w368) -> ("Main Config.TCU Module Configs"=w377:T50[])
          n126 = Unbundle By Name(w383) -> ("GUID"=w380:string)
          n127 = Empty Array?(array=w377) -> (empty?=w384:bool)
          n128 = Format Into String(format string="Could not save TCU Module config. No matching GUID for \"%s\"." ("error message (\"\")"), w380) -> (resulting string=w381:string)  [unwired: 2 in, 1 out]
          n129 = case shown="False" w384 {
            tunnel: w380 -> [w392 _]
            tunnel: w377 -> [w390 w409]
            tunnel: w383 -> [w389 w408]
            tunnel: [w388 w407] -> w376
            tunnel: w381 -> [w387 _]
            tunnel: w379 -> [w386 w406]
            tunnel: [w385 w406] -> w378
            frame False {
              n130 = for {
                tunnel: w390 -> [w405] mode=indexing
                tunnel: [w404] -> w393 mode=indexing
                workers-P: _ -> [_]
                n131 = Unbundle By Name(w405) -> ("GUID"=w404:string)
              }
              n132 = Search 1D Array(1D array=w393, element=w392) -> (index of element=w391:i32)  [unwired: 1 in]
              n133 = case shown="0, Default" w391 {
                selector: w391 -> [w397 _]
                tunnel: w390 -> [w398 w403]
                tunnel: w389 -> [w396 _]
                tunnel: [w395 w403] -> w388
                tunnel: w387 -> [_ w401]
                tunnel: w386 -> [w394 w400]
                tunnel: [w394 w399] -> w385
                frame 0, Default {
                  n134 = Replace Array Subset(array=w398, new element=w396, index=w397) -> (w395:T50[])
                }
                frame -1 {
                  n135 = call <vilib>:"Error Cluster From Error Code.vi"("error in (no error)"=w400, "error message (\"\")"=w401, "error code (0)"=7004) -> ("error out"=w399:errorcluster)  [unwired: 6 in]
                }
              }
            }
            frame True {
              n136 = Build Array (concatenate)(w409, w408) -> (w407:T50[])
            }
          }
          n137 = in-place-cluster #6("Main Config.TCU Module Configs"=w376) -> (w367:T1)
        }
        n138 = call "Write to Log File.vi"("error in"=w369, "text"="Main: Commit Config (TCU)") -> ()  [unwired: 9 in, 1 out]
      }
      frame "Commit Config (Scale Module)" {
        w414 = T42 {"GUID"="", "Drop Coords"={"Horizontal"=0, "Vertical"=0}, "Process Name"="", "Queue Name"="", "Settings"={"Cycle Period"=500.0, "Mettler"={"VISA resource name"="", "Simulated?"=FALSE}, "Scale Type"=""}, "Load Count"=0}  # Scale Module Config
        # "Save Scale Module Settings"
        n139 = Variant To Data(error in=w417, type=w414, Variant=w418) -> (data=w416:T42, error out=w415:errorcluster)
        n140 = in-place {
          in-place-border: w416 -> [w426]
          in-place-border: w415 -> [w422]
          in-place-border: [w421] -> w412
          n141 = in-place-cluster #7(w411) -> ("Main Config.Scale Module Configs"=w420:T42[])
          n142 = Unbundle By Name(w426) -> ("GUID"=w423:string)
          n143 = Empty Array?(array=w420) -> (empty?=w427:bool)
          n144 = Format Into String(format string="Could not save Scale Module config. No matching GUID for \"%s\"." ("error message (\"\")"), w423) -> (resulting string=w424:string)  [unwired: 2 in, 1 out]
          n145 = case shown="True" w427 {
            tunnel: w423 -> [w435 _]
            tunnel: w420 -> [w433 w452]
            tunnel: w426 -> [w432 w451]
            tunnel: [w431 w450] -> w419
            tunnel: w424 -> [w430 _]
            tunnel: w422 -> [w429 w449]
            tunnel: [w428 w449] -> w421
            frame False {
              n146 = for {
                tunnel: w433 -> [w448] mode=indexing
                tunnel: [w447] -> w436 mode=indexing
                workers-P: _ -> [_]
                n147 = Unbundle By Name(w448) -> ("GUID"=w447:string)
              }
              n148 = Search 1D Array(1D array=w436, element=w435) -> (index of element=w434:i32)  [unwired: 1 in]
              n149 = case shown="0, Default" w434 {
                selector: w434 -> [w440 _]
                tunnel: w433 -> [w441 w446]
                tunnel: w432 -> [w439 _]
                tunnel: [w438 w446] -> w431
                tunnel: w430 -> [_ w444]
                tunnel: w429 -> [w437 w443]
                tunnel: [w437 w442] -> w428
                frame 0, Default {
                  n150 = Replace Array Subset(array=w441, new element=w439, index=w440) -> (w438:T42[])
                }
                frame -1 {
                  n151 = call <vilib>:"Error Cluster From Error Code.vi"("error in (no error)"=w443, "error message (\"\")"=w444, "error code (0)"=7004) -> ("error out"=w442:errorcluster)  [unwired: 6 in]
                }
              }
            }
            frame True {
              n152 = Build Array (concatenate)(w452, w451) -> (w450:T42[])
            }
          }
          n153 = in-place-cluster #7("Main Config.Scale Module Configs"=w419) -> (w410:T1)
        }
        n154 = call "Write to Log File.vi"("error in"=w412, "text"="Main: Commit Config (Scale Module)") -> ()  [unwired: 9 in, 1 out]
      }
      frame "Commit Config (Flow Module)" {
        w457 = T48 {"GUID"="", "Drop Coords"={"Horizontal"=0, "Vertical"=0}, "Process Name"="", "Queue Name"="", "Settings"={"Cycle Period"=500.0, "Flow Meter Type"="", "Bronkhorst M13 Settings"={"VISA resource name"="", "Simulated?"=FALSE, "Smoothing Steps"=1}, "Bronkhorst M14 Settings"={"VISA resource name"="", "Simulated?"=FALSE, "Smoothing Steps"=1}}, "Load Count"=0}  # Flow Module Config
        # "Save Flow Module Settings"
        n155 = Variant To Data(error in=w460, type=w457, Variant=w461) -> (data=w459:T48, error out=w458:errorcluster)
        n156 = in-place {
          in-place-border: w459 -> [w469]
          in-place-border: w458 -> [w465]
          in-place-border: [w464] -> w455
          n157 = in-place-cluster #8(w454) -> ("Main Config.Flow Module Configs"=w462:T48[])
          n158 = Unbundle By Name(w469) -> ("GUID"=w466:string)
          n159 = Empty Array?(array=w462) -> (empty?=w470:bool)
          n160 = Format Into String(format string="Could not save Scale Module config. No matching GUID for \"%s\"." ("error message (\"\")"), w466) -> (resulting string=w467:string)  [unwired: 2 in, 1 out]
          n161 = case shown="True" w470 {
            tunnel: w466 -> [w478 _]
            tunnel: w462 -> [w476 w495]
            tunnel: w469 -> [w475 w494]
            tunnel: [w474 w493] -> w463
            tunnel: w467 -> [w473 _]
            tunnel: w465 -> [w472 w492]
            tunnel: [w471 w492] -> w464
            frame False {
              n162 = for {
                tunnel: w476 -> [w491] mode=indexing
                tunnel: [w490] -> w479 mode=indexing
                workers-P: _ -> [_]
                n163 = Unbundle By Name(w491) -> ("GUID"=w490:string)
              }
              n164 = Search 1D Array(1D array=w479, element=w478) -> (index of element=w477:i32)  [unwired: 1 in]
              n165 = case shown="0, Default" w477 {
                selector: w477 -> [w483 _]
                tunnel: w476 -> [w484 w489]
                tunnel: w475 -> [w482 _]
                tunnel: [w481 w489] -> w474
                tunnel: w473 -> [_ w487]
                tunnel: w472 -> [w480 w486]
                tunnel: [w480 w485] -> w471
                frame 0, Default {
                  n166 = Replace Array Subset(array=w484, new element=w482, index=w483) -> (w481:T48[])
                }
                frame -1 {
                  n167 = call <vilib>:"Error Cluster From Error Code.vi"("error in (no error)"=w486, "error message (\"\")"=w487, "error code (0)"=7004) -> ("error out"=w485:errorcluster)  [unwired: 6 in]
                }
              }
            }
            frame True {
              n168 = Build Array (concatenate)(w495, w494) -> (w493:T48[])
            }
          }
          n169 = in-place-cluster #8("Main Config.Flow Module Configs"=w463) -> (w453:T1)
        }
        n170 = call "Write to Log File.vi"("error in"=w455, "text"="Main: Commit Config (Flow Module)") -> ()  [unwired: 9 in, 1 out]
      }
      frame "Commit Config (TT)" {
        # "Save Temperature Transmitter Module Settings"
        n171 = Variant To Data(error in=w502, type=T37 {"GUID"="", "Drop Coords"={"Horizontal"=0, "Vertical"=0}, "Input Channel Tag Name "="", "Process Name"="", "Queue Name"="", "Input Channel Numeric Alarm Settings"=[]} ("TT Module Config"), Variant=w503) -> (data=w501:T37, error out=w500:errorcluster)
        n172 = in-place {
          in-place-border: w501 -> [w512]
          in-place-border: w500 -> [w508]
          in-place-border: [w507] -> w498
          n173 = in-place-cluster #9(w497) -> ("Main Config.TT Module Configs"=w505:T37[])
          n174 = Unbundle By Name(w512) -> ("GUID"=w509:string)
          n175 = Empty Array?(array=w505) -> (empty?=w513:bool)
          n176 = Format Into String(format string="Could not save TT Module config. No matching GUID for \"%s\"." ("error message (\"\")"), w509) -> (resulting string=w510:string)  [unwired: 2 in, 1 out]
          n177 = case shown="True" w513 {
            tunnel: w509 -> [w521 _]
            tunnel: w505 -> [w519 w538]
            tunnel: w512 -> [w518 w537]
            tunnel: [w517 w536] -> w506
            tunnel: w510 -> [w516 _]
            tunnel: w508 -> [w515 w535]
            tunnel: [w514 w535] -> w507
            frame False {
              n178 = for {
                tunnel: w519 -> [w534] mode=indexing
                tunnel: [w533] -> w522 mode=indexing
                workers-P: _ -> [_]
                n179 = Unbundle By Name(w534) -> ("GUID"=w533:string)
              }
              n180 = Search 1D Array(1D array=w522, element=w521) -> (index of element=w520:i32)  [unwired: 1 in]
              n181 = case shown="0, Default" w520 {
                selector: w520 -> [w526 _]
                tunnel: w519 -> [w527 w532]
                tunnel: w518 -> [w525 _]
                tunnel: [w524 w532] -> w517
                tunnel: w516 -> [_ w530]
                tunnel: w515 -> [w523 w529]
                tunnel: [w523 w528] -> w514
                frame 0, Default {
                  n182 = Replace Array Subset(array=w527, new element=w525, index=w526) -> (w524:T37[])
                }
                frame -1 {
                  n183 = call <vilib>:"Error Cluster From Error Code.vi"("error in (no error)"=w529, "error message (\"\")"=w530, "error code (0)"=7003) -> ("error out"=w528:errorcluster)  [unwired: 6 in]
                }
              }
            }
            frame True {
              n184 = Build Array (concatenate)(w538, w537) -> (w536:T37[])
            }
          }
          n185 = in-place-cluster #9("Main Config.TT Module Configs"=w506) -> (w496:T1)
        }
        n186 = call "Write to Log File.vi"("error in"=w498, "text"="Main: Commit Config (TT)") -> ()  [unwired: 9 in, 1 out]
      }
      frame "Commit Config (PT)" {
        # "Save Pressure Transmitter Module Settings"
        n187 = Variant To Data(error in=w545, type=T41 {"GUID"="", "Drop Coords"={"Horizontal"=0, "Vertical"=0}, "Input Channel Tag Name "="", "Process Name"="", "Queue Name"="", "Input Channel Numeric Alarm Settings"=[]} ("TT Module Config"), Variant=w546) -> (data=w544:T41, error out=w543:errorcluster)
        n188 = in-place {
          in-place-border: w544 -> [w555]
          in-place-border: w543 -> [w551]
          in-place-border: [w550] -> w541
          n189 = in-place-cluster #10(w540) -> ("Main Config.PT Module Configs"=w549:T41[])
          n190 = Unbundle By Name(w555) -> ("GUID"=w552:string)
          n191 = Empty Array?(array=w549) -> (empty?=w556:bool)
          n192 = Format Into String(format string="Could not save PT Module config. No matching GUID for \"%s\"." ("error message (\"\")"), w552) -> (resulting string=w553:string)  [unwired: 2 in, 1 out]
          n193 = case shown="True" w556 {
            tunnel: w552 -> [w564 _]
            tunnel: w549 -> [w562 w581]
            tunnel: w555 -> [w561 w580]
            tunnel: [w560 w579] -> w548
            tunnel: w553 -> [w559 _]
            tunnel: w551 -> [w558 w578]
            tunnel: [w557 w578] -> w550
            frame False {
              n194 = for {
                tunnel: w562 -> [w577] mode=indexing
                tunnel: [w576] -> w565 mode=indexing
                workers-P: _ -> [_]
                n195 = Unbundle By Name(w577) -> ("GUID"=w576:string)
              }
              n196 = Search 1D Array(1D array=w565, element=w564) -> (index of element=w563:i32)  [unwired: 1 in]
              n197 = case shown="0, Default" w563 {
                selector: w563 -> [w569 _]
                tunnel: w562 -> [w570 w575]
                tunnel: w561 -> [w568 _]
                tunnel: [w567 w575] -> w560
                tunnel: w559 -> [_ w573]
                tunnel: w558 -> [w566 w572]
                tunnel: [w566 w571] -> w557
                frame 0, Default {
                  n198 = Replace Array Subset(array=w570, new element=w568, index=w569) -> (w567:T41[])
                }
                frame -1 {
                  n199 = call <vilib>:"Error Cluster From Error Code.vi"("error in (no error)"=w572, "error message (\"\")"=w573, "error code (0)"=7005) -> ("error out"=w571:errorcluster)  [unwired: 6 in]
                }
              }
            }
            frame True {
              n200 = Build Array (concatenate)(w581, w580) -> (w579:T41[])
            }
          }
          n201 = in-place-cluster #10("Main Config.PT Module Configs"=w548) -> (w539:T1)
        }
        n202 = call "Write to Log File.vi"("error in"=w541, "text"="Main: Commit Config (PT)") -> ()  [unwired: 9 in, 1 out]
      }
      frame "Commit Config (U3)" {
        # "Save LabJack U3 Module Settings"
        n203 = Variant To Data(error in=w588, type=T46 {"GUID"="", "Drop Coords"={"Horizontal"=0, "Vertical"=0}, "AI Channel Number"=enum."Default", "Process Name"="", "Queue Name"="", "Input Channel Numeric Alarm Settings"=[]} ("TT Module Config"), Variant=w589) -> (data=w587:T46, error out=w586:errorcluster)
        n204 = in-place {
          in-place-border: w587 -> [w598]
          in-place-border: w586 -> [w594]
          in-place-border: [w593] -> w584
          n205 = in-place-cluster #11(w583) -> ("Main Config.U3 Module Configs"=w592:T46[])
          n206 = Unbundle By Name(w598) -> ("GUID"=w595:string)
          n207 = Empty Array?(array=w592) -> (empty?=w599:bool)
          n208 = Format Into String(format string="Could not save U3 Module config. No matching GUID for \"%s\"." ("error message (\"\")"), w595) -> (resulting string=w596:string)  [unwired: 2 in, 1 out]
          n209 = case shown="True" w599 {
            tunnel: w595 -> [w607 _]
            tunnel: w592 -> [w605 w624]
            tunnel: w598 -> [w604 w623]
            tunnel: [w603 w622] -> w591
            tunnel: w596 -> [w602 _]
            tunnel: w594 -> [w601 w621]
            tunnel: [w600 w621] -> w593
            frame False {
              n210 = for {
                tunnel: w605 -> [w620] mode=indexing
                tunnel: [w619] -> w608 mode=indexing
                workers-P: _ -> [_]
                n211 = Unbundle By Name(w620) -> ("GUID"=w619:string)
              }
              n212 = Search 1D Array(1D array=w608, element=w607) -> (index of element=w606:i32)  [unwired: 1 in]
              n213 = case shown="-1" w606 {
                selector: w606 -> [w612 _]
                tunnel: w605 -> [w613 w618]
                tunnel: w604 -> [w611 _]
                tunnel: [w610 w618] -> w603
                tunnel: w602 -> [_ w616]
                tunnel: w601 -> [w609 w615]
                tunnel: [w609 w614] -> w600
                frame 0, Default {
                  n214 = Replace Array Subset(array=w613, new element=w611, index=w612) -> (w610:T46[])
                }
                frame -1 {
                  n215 = call <vilib>:"Error Cluster From Error Code.vi"("error in (no error)"=w615, "error message (\"\")"=w616, "error code (0)"=7005) -> ("error out"=w614:errorcluster)  [unwired: 6 in]
                }
              }
            }
            frame True {
              n216 = Build Array (concatenate)(w624, w623) -> (w622:T46[])
            }
          }
          n217 = in-place-cluster #11("Main Config.U3 Module Configs"=w591) -> (w582:T1)
        }
        n218 = call "Write to Log File.vi"("error in"=w584, "text"="Main: Commit Config (U3)") -> ()  [unwired: 9 in, 1 out]
      }
      frame "Commit Config (SC)" {
        # "Save LabJack U3 Module Settings"
        n219 = Variant To Data(error in=w632, type=T68 {"GUID"="", "Drop Coords"={"Horizontal"=0, "Vertical"=0}, "Process Name"="", "Queue Name"="", "Settings"={"Cycle Period"=500.0, "Mettler"={"VISA resource name"="", "Simulated?"=FALSE}, "Scale Type"=""}, "Load Count"=0} ("Scale Module Config"), Variant=w633) -> (data=w631:T68, error out=w630:errorcluster)
        n220 = in-place {
          in-place-border: w631 -> [w641]
          in-place-border: w630 -> [w637]
          in-place-border: [w636] -> w628
          n221 = in-place-cluster #12(w627) -> ("Main Config.SC Module Configs"=w635:T68[])
          n222 = Unbundle By Name(w641) -> ("GUID"=w638:string)
          n223 = Empty Array?(array=w635) -> (empty?=w642:bool)
          n224 = Format Into String(format string="Could not save SC Module config. No matching GUID for \"%s\"." ("error message (\"\")"), w638) -> (resulting string=w639:string)  [unwired: 2 in, 1 out]
          n225 = case shown="True" w642 {
            tunnel: w638 -> [w650 _]
            tunnel: w635 -> [w648 w667]
            tunnel: w641 -> [w647 w666]
            tunnel: [w646 w665] -> w634
            tunnel: w639 -> [w645 _]
            tunnel: w637 -> [w644 w664]
            tunnel: [w643 w664] -> w636
            frame False {
              n226 = for {
                tunnel: w648 -> [w663] mode=indexing
                tunnel: [w662] -> w651 mode=indexing
                workers-P: _ -> [_]
                n227 = Unbundle By Name(w663) -> ("GUID"=w662:string)
              }
              n228 = Search 1D Array(1D array=w651, element=w650) -> (index of element=w649:i32)  [unwired: 1 in]
              n229 = case shown="-1" w649 {
                selector: w649 -> [w655 _]
                tunnel: w648 -> [w656 w661]
                tunnel: w647 -> [w654 _]
                tunnel: [w653 w661] -> w646
                tunnel: w645 -> [_ w659]
                tunnel: w644 -> [w652 w658]
                tunnel: [w652 w657] -> w643
                frame 0, Default {
                  n230 = Replace Array Subset(array=w656, new element=w654, index=w655) -> (w653:T68[])
                }
                frame -1 {
                  n231 = call <vilib>:"Error Cluster From Error Code.vi"("error in (no error)"=w658, "error message (\"\")"=w659, "error code (0)"=7005) -> ("error out"=w657:errorcluster)  [unwired: 6 in]
                }
              }
            }
            frame True {
              n232 = Build Array (concatenate)(w667, w666) -> (w665:T68[])
            }
          }
          n233 = in-place-cluster #12("Main Config.SC Module Configs"=w634) -> (w626:T1)
        }
        n234 = call "Write to Log File.vi"("error in"=w628, "text"="Main: Commit Config (SC)") -> ()  [unwired: 9 in, 1 out]
      }
      frame "Delete Module" {
        w678 = ""  # GUID
        # "This message is called when a user deletes a module from the canvas. The GUID for the module is passed here and we delete it from the list."
        n235 = Variant To Data(error in=w676, type=w678, Variant=w677) -> (data=w673:string, error out=w675:errorcluster)
        n236 = in-place {
          in-place-border: w675 -> [w683]
          in-place-border: w673 -> [w682]
          in-place-border: [w681] -> w670
          n237 = in-place-cluster #13(w669) -> ("Main Config"=w680:T7)
          n238 = call "Delete GUID Module.vi"("error in (no error)"=w683, "GUID"=w682, "Main Config in"=w680) -> ("error out"=w681:errorcluster, "Main Config out"=w679:T7)  [unwired: 7 in]
          n239 = in-place-cluster #13("Main Config"=w679) -> (w668:T1)
        }
        n240 = Concatenate Strings("Main: GUID " ("string"), w673, " Deleted" ("string")) -> (w674:string)
        n241 = call "Write to Log File.vi"("error in"=w670, "text"=w674) -> ()  [unwired: 9 in, 1 out]
      }
      frame "Update Config (DAQ)" {
        n242 = Unbundle By Name(w688) -> ("Main Config.DAQ Config"=w687:T39)
        n243 = call-poly "Enqueue Message.vi"("error in (no error)"=w686, "Message Data"=w687, "Message"="DAQ-Update Settings", "Message Queue"=w689) -> ("error out"=w684:errorcluster)  [unwired: 6 in, 1 out]
        n244 = call "Write to Log File.vi"("error in"=w684, "text"="Main: Update Config (DAQ)") -> ()  [unwired: 9 in, 1 out]
      }
      frame "Update Config (TT)" {
        # "Create TT Modules and \"drop\" them on the Picture Control and assign configs"
        n245 = Unbundle By Name(w697) -> ("Main Config.TT Module Configs"=w696:T37[])
        n246 = property class="VI"() -> ("Front Panel.Title"=w695:string)  [unwired: 2 in, 2 out]
        n247 = for {
          shift-right: [w714] -> w698
          shift-left: w697 -> [w713]
          tunnel: w696 -> [w710] mode=indexing
          tunnel: w695 -> [w707]
          tunnel: w694 -> [w705]
          shift-right: [w704] -> w691
          shift-left: w693 -> [w703]
          # "TT (Main).vit"
          n248 = vi-ref "TT (Main).vi"() -> (w702:refnum<vi>)
          n249 = Unbundle By Name(w710) -> ("Process Name"=w709:string, "Drop Coords"=w706:T10)
          n250 = To Variant(anything=w710) -> (Variant=w711:variant)
          n251 = property class="VI"(reference=w702) -> ("Path"=w701:path)  [unwired: 1 in, 2 out]
          n252 = Bundle By Name(cluster=T82 {"Module VI Filepath"=path "", "Process Name"="", "Main UI Message Queue"=refnum, "Drop Coords"={"Horizontal"=0, "Vertical"=0}, "Module Parameters"=variant, "Name of Parent Window"=""} ("Drop Parameters"), "Module VI Filepath"=w701, "Module Parameters"=w711, "Process Name"=w709, "Main UI Message Queue"=w705, "Drop Coords"=w706, "Name of Parent Window"=w707) -> (w708:T82)
          n253 = call "Next Instance Number.vi"("Module Type"=Module_Type_Enum."TT", "Operation"=Module_Instance_Number_Operation_Enum."Next Instance Number") -> ()  [unwired: 8 in, 2 out]
          n254 = call "Drop Start VI.vi"("error in (no error)"=w703, "Drop Parameters"=w708, "State in"=w713) -> ("error out"=w704:errorcluster, "State out"=w714:T1)  [unwired: 7 in]
        }
        n255 = call "Write to Log File.vi"("error in"=w691, "text"="Main: Update Config (TT)") -> ()  [unwired: 9 in, 1 out]
      }
      frame "Update Config (PT)" {
        # "Create PT Modules and \"drop\" them on the Picture Control and assign configs"
        n256 = Unbundle By Name(w721) -> ("Main Config.PT Module Configs"=w720:T41[])
        n257 = property class="VI"() -> ("Front Panel.Title"=w719:string)  [unwired: 2 in, 2 out]
        n258 = for {
          shift-right: [w738] -> w722
          shift-left: w721 -> [w737]
          tunnel: w720 -> [w734] mode=indexing
          tunnel: w719 -> [w731]
          tunnel: w718 -> [w729]
          shift-right: [w728] -> w715
          shift-left: w717 -> [w727]
          n259 = vi-ref "PT (Main).vi"() -> (w726:refnum<vi>)
          n260 = To Variant(anything=w734) -> (Variant=w735:variant)
          n261 = Unbundle By Name(w734) -> ("Process Name"=w733:string, "Drop Coords"=w730:T10)
          n262 = property class="VI"(reference=w726) -> ("Path"=w725:path)  [unwired: 1 in, 2 out]
          n263 = Bundle By Name(cluster=T82 {"Module VI Filepath"=path "", "Process Name"="", "Main UI Message Queue"=refnum, "Drop Coords"={"Horizontal"=0, "Vertical"=0}, "Module Parameters"=variant, "Name of Parent Window"=""} ("Drop Parameters"), "Module VI Filepath"=w725, "Module Parameters"=w735, "Process Name"=w733, "Main UI Message Queue"=w729, "Drop Coords"=w730, "Name of Parent Window"=w731) -> (w732:T82)
          n264 = call "Drop Start VI.vi"("error in (no error)"=w727, "Drop Parameters"=w732, "State in"=w737) -> ("error out"=w728:errorcluster, "State out"=w738:T1)  [unwired: 7 in]
          n265 = call "Next Instance Number.vi"("Module Type"=Module_Type_Enum."PT", "Operation"=Module_Instance_Number_Operation_Enum."Next Instance Number") -> ()  [unwired: 8 in, 2 out]
        }
        n266 = call "Write to Log File.vi"("error in"=w715, "text"="Main: Update Config (PT)") -> ()  [unwired: 9 in, 1 out]
      }
      frame "Update Config (U3)" {
        # "Create U3 Modules and \"drop\" them on the Picture Control and assign configs"
        n267 = Unbundle By Name(w745) -> ("Main Config.U3 Module Configs"=w744:T46[])
        n268 = property class="VI"() -> ("Front Panel.Title"=w743:string)  [unwired: 2 in, 2 out]
        n269 = for {
          shift-right: [w762] -> w746
          shift-left: w745 -> [w761]
          tunnel: w744 -> [w758] mode=indexing
          tunnel: w743 -> [w755]
          tunnel: w742 -> [w753]
          shift-right: [w752] -> w739
          shift-left: w741 -> [w751]
          n270 = vi-ref "U3 Module.lvlib:U3 (Main).vit"() -> (w750:refnum<vi>)
          n271 = Unbundle By Name(w758) -> ("Process Name"=w757:string, "Drop Coords"=w754:T10)
          n272 = To Variant(anything=w758) -> (Variant=w759:variant)
          n273 = property class="VI"(reference=w750) -> ("Path"=w749:path)  [unwired: 1 in, 2 out]
          n274 = Bundle By Name(cluster=T82 {"Module VI Filepath"=path "", "Process Name"="", "Main UI Message Queue"=refnum, "Drop Coords"={"Horizontal"=0, "Vertical"=0}, "Module Parameters"=variant, "Name of Parent Window"=""} ("Drop Parameters"), "Module VI Filepath"=w749, "Module Parameters"=w759, "Process Name"=w757, "Main UI Message Queue"=w753, "Drop Coords"=w754, "Name of Parent Window"=w755) -> (w756:T82)
          n275 = call "Drop Start VI.vi"("error in (no error)"=w751, "Drop Parameters"=w756, "State in"=w761) -> ("error out"=w752:errorcluster, "State out"=w762:T1)  [unwired: 7 in]
          n276 = call "Next Instance Number.vi"("Module Type"=Module_Type_Enum."U3", "Operation"=Module_Instance_Number_Operation_Enum."Next Instance Number") -> ()  [unwired: 8 in, 2 out]
        }
        n277 = call "Write to Log File.vi"("error in"=w739, "text"="Main: Update Config (U3)") -> ()  [unwired: 9 in, 1 out]
      }
      frame "Update Config (Feed)" {
        # "Create Feed Modules and \"drop\" them on the Picture Control and assign configs"
        n278 = Unbundle By Name(w769) -> ("Main Config.Feed Module Configs"=w768:T18[])
        n279 = property class="VI"() -> ("Front Panel.Title"=w767:string)  [unwired: 2 in, 2 out]
        n280 = for {
          shift-right: [w786] -> w770
          shift-left: w769 -> [w785]
          tunnel: w768 -> [w782] mode=indexing
          tunnel: w767 -> [w779]
          tunnel: w766 -> [w777]
          shift-right: [w776] -> w763
          shift-left: w765 -> [w775]
          # "Feed Module (Main.vit"
          n281 = vi-ref "Feed Module (Main).vi"() -> (w774:refnum<vi>)
          n282 = To Variant(anything=w782) -> (Variant=w783:variant)
          n283 = Unbundle By Name(w782) -> ("Process Name"=w781:string, "Drop Coords"=w778:T10)
          n284 = property class="VI"(reference=w774) -> ("Path"=w773:path)  [unwired: 1 in, 2 out]
          n285 = Bundle By Name(cluster=T82 {"Module VI Filepath"=path "", "Process Name"="", "Main UI Message Queue"=refnum, "Drop Coords"={"Horizontal"=0, "Vertical"=0}, "Module Parameters"=variant, "Name of Parent Window"=""} ("Drop Parameters"), "Module VI Filepath"=w773, "Module Parameters"=w783, "Process Name"=w781, "Main UI Message Queue"=w777, "Drop Coords"=w778, "Name of Parent Window"=w779) -> (w780:T82)
          n286 = call "Drop Start VI.vi"("error in (no error)"=w775, "Drop Parameters"=w780, "State in"=w785) -> ("error out"=w776:errorcluster, "State out"=w786:T1)  [unwired: 7 in]
          n287 = call "Next Instance Number.vi"("Module Type"=Module_Type_Enum."Feed", "Operation"=Module_Instance_Number_Operation_Enum."Next Instance Number") -> ()  [unwired: 8 in, 2 out]
        }
        n288 = call "Write to Log File.vi"("error in"=w763, "text"="Main: Update Config (Feed)") -> ()  [unwired: 9 in, 1 out]
      }
      frame "Update Config (OPC)" {
        # "Create Feed Modules and \"drop\" them on the Picture Control and assign configs"
        n289 = Unbundle By Name(w793) -> ("Main Config.OPC Module Configs"=w792:T8[])
        n290 = property class="VI"() -> ("Front Panel.Title"=w791:string)  [unwired: 2 in, 2 out]
        n291 = for {
          shift-right: [w810] -> w794
          shift-left: w793 -> [w809]
          tunnel: w792 -> [w806] mode=indexing
          tunnel: w791 -> [w803]
          tunnel: w790 -> [w801]
          shift-right: [w800] -> w787
          shift-left: w789 -> [w799]
          # "OPC Module (Main).vit"
          n292 = vi-ref "OPC Main.vi"() -> (w798:refnum<vi>)
          n293 = To Variant(anything=w806) -> (Variant=w807:variant)
          n294 = Unbundle By Name(w806) -> ("Process Name"=w805:string, "Drop Coords"=w802:T10)
          n295 = property class="VI"(reference=w798) -> ("Path"=w797:path)  [unwired: 1 in, 2 out]
          n296 = Bundle By Name(cluster=T82 {"Module VI Filepath"=path "", "Process Name"="", "Main UI Message Queue"=refnum, "Drop Coords"={"Horizontal"=0, "Vertical"=0}, "Module Parameters"=variant, "Name of Parent Window"=""} ("Drop Parameters"), "Module VI Filepath"=w797, "Module Parameters"=w807, "Process Name"=w805, "Main UI Message Queue"=w801, "Drop Coords"=w802, "Name of Parent Window"=w803) -> (w804:T82)
          n297 = call "Drop Start VI.vi"("error in (no error)"=w799, "Drop Parameters"=w804, "State in"=w809) -> ("error out"=w800:errorcluster, "State out"=w810:T1)  [unwired: 7 in]
          n298 = call "Next Instance Number.vi"("Module Type"=Module_Type_Enum."OPC", "Operation"=Module_Instance_Number_Operation_Enum."Next Instance Number") -> ()  [unwired: 8 in, 2 out]
        }
        n299 = call "Write to Log File.vi"("error in"=w787, "text"="Main: Update Config (Feed)") -> ()  [unwired: 9 in, 1 out]
      }
      frame "Update Config (Pump)" {
        # "Create Pump Modules and \"drop\" them on the Picture Control and assign configs"
        n300 = Unbundle By Name(w817) -> ("Main Config.Pump Module Configs"=w816:T44[])
        n301 = property class="VI"() -> ("Front Panel.Title"=w815:string)  [unwired: 2 in, 2 out]
        n302 = for {
          shift-right: [w834] -> w818
          shift-left: w817 -> [w833]
          tunnel: w816 -> [w830] mode=indexing
          tunnel: w815 -> [w827]
          tunnel: w814 -> [w825]
          shift-right: [w824] -> w811
          shift-left: w813 -> [w823]
          # "Pump Module (Main).vit"
          n303 = vi-ref "Pump Module (Main).vi"() -> (w822:refnum<vi>)
          n304 = To Variant(anything=w830) -> (Variant=w831:variant)
          n305 = Unbundle By Name(w830) -> ("Process Name"=w829:string, "Drop Coords"=w826:T10)
          n306 = property class="VI"(reference=w822) -> ("Path"=w821:path)  [unwired: 1 in, 2 out]
          n307 = Bundle By Name(cluster=T82 {"Module VI Filepath"=path "", "Process Name"="", "Main UI Message Queue"=refnum, "Drop Coords"={"Horizontal"=0, "Vertical"=0}, "Module Parameters"=variant, "Name of Parent Window"=""} ("Drop Parameters"), "Module VI Filepath"=w821, "Module Parameters"=w831, "Process Name"=w829, "Main UI Message Queue"=w825, "Drop Coords"=w826, "Name of Parent Window"=w827) -> (w828:T82)
          n308 = call "Drop Start VI.vi"("error in (no error)"=w823, "Drop Parameters"=w828, "State in"=w833) -> ("error out"=w824:errorcluster, "State out"=w834:T1)  [unwired: 7 in]
          n309 = call "Next Instance Number.vi"("Module Type"=Module_Type_Enum."Pump", "Operation"=Module_Instance_Number_Operation_Enum."Next Instance Number") -> ()  [unwired: 8 in, 2 out]
        }
        n310 = call "Write to Log File.vi"("error in"=w811, "text"="Main: Update Config (Pump)") -> ()  [unwired: 9 in, 1 out]
      }
      frame "Update Config (DO)" {
        # "Create DO Modules and \"drop\" them on the Picture Control and assign configs"
        n311 = Unbundle By Name(w841) -> ("Main Config.DO Module Configs"=w840:T59[])
        n312 = property class="VI"() -> ("Front Panel.Title"=w839:string)  [unwired: 2 in, 2 out]
        n313 = for {
          shift-right: [w858] -> w842
          shift-left: w841 -> [w857]
          tunnel: w840 -> [w854] mode=indexing
          tunnel: w839 -> [w851]
          tunnel: w838 -> [w849]
          shift-right: [w848] -> w835
          shift-left: w837 -> [w847]
          # "DO Module (Main).vit"
          n314 = vi-ref "D-O Module.lvlib:D-O Module (Main).vi"() -> (w846:refnum<vi>)
          n315 = To Variant(anything=w854) -> (Variant=w855:variant)
          n316 = Unbundle By Name(w854) -> ("Process Name"=w853:string, "Drop Coords"=w850:T10)
          n317 = property class="VI"(reference=w846) -> ("Path"=w845:path)  [unwired: 1 in, 2 out]
          n318 = Bundle By Name(cluster=T82 {"Module VI Filepath"=path "", "Process Name"="", "Main UI Message Queue"=refnum, "Drop Coords"={"Horizontal"=0, "Vertical"=0}, "Module Parameters"=variant, "Name of Parent Window"=""} ("Drop Parameters"), "Module VI Filepath"=w845, "Module Parameters"=w855, "Process Name"=w853, "Main UI Message Queue"=w849, "Drop Coords"=w850, "Name of Parent Window"=w851) -> (w852:T82)
          n319 = call "Drop Start VI.vi"("error in (no error)"=w847, "Drop Parameters"=w852, "State in"=w857) -> ("error out"=w848:errorcluster, "State out"=w858:T1)  [unwired: 7 in]
          n320 = call "Next Instance Number.vi"("Module Type"=Module_Type_Enum."Pump", "Operation"=Module_Instance_Number_Operation_Enum."Next Instance Number") -> ()  [unwired: 8 in, 2 out]
        }
        n321 = call "Write to Log File.vi"("error in"=w835, "text"="Main: Update Config (DO)") -> ()  [unwired: 9 in, 1 out]
      }
      frame "Update Config (PR)" {
        # "Create Pressure Regulator Modules and \"drop\" them on the Picture Control and assign configs"
        n322 = Unbundle By Name(w865) -> ("Main Config.PR Module Configs"=w864:T64[])
        n323 = property class="VI"() -> ("Front Panel.Title"=w863:string)  [unwired: 2 in, 2 out]
        n324 = for {
          shift-right: [w882] -> w866
          shift-left: w865 -> [w881]
          tunnel: w864 -> [w878] mode=indexing
          tunnel: w863 -> [w875]
          tunnel: w862 -> [w873]
          shift-right: [w872] -> w859
          shift-left: w861 -> [w871]
          # "PR Module (Main).vit"
          n325 = vi-ref "4-20mA Module (Main).vi"() -> (w870:refnum<vi>)
          n326 = To Variant(anything=w878) -> (Variant=w879:variant)
          n327 = Unbundle By Name(w878) -> ("Process Name"=w877:string, "Drop Coords"=w874:T10)
          n328 = property class="VI"(reference=w870) -> ("Path"=w869:path)  [unwired: 1 in, 2 out]
          n329 = Bundle By Name(cluster=T82 {"Module VI Filepath"=path "", "Process Name"="", "Main UI Message Queue"=refnum, "Drop Coords"={"Horizontal"=0, "Vertical"=0}, "Module Parameters"=variant, "Name of Parent Window"=""} ("Drop Parameters"), "Module VI Filepath"=w869, "Module Parameters"=w879, "Process Name"=w877, "Main UI Message Queue"=w873, "Drop Coords"=w874, "Name of Parent Window"=w875) -> (w876:T82)
          n330 = call "Drop Start VI.vi"("error in (no error)"=w871, "Drop Parameters"=w876, "State in"=w881) -> ("error out"=w872:errorcluster, "State out"=w882:T1)  [unwired: 7 in]
          n331 = call "Next Instance Number.vi"("Module Type"=Module_Type_Enum."Pump", "Operation"=Module_Instance_Number_Operation_Enum."Next Instance Number") -> ()  [unwired: 8 in, 2 out]
        }
        n332 = call "Write to Log File.vi"("error in"=w859, "text"="Main: Update Config (PR)") -> ()  [unwired: 9 in, 1 out]
      }
      frame "Update Config (TCU)" {
        # "Create TCU Modules and \"drop\" them on the Picture Control and assign configs"
        n333 = Unbundle By Name(w889) -> ("Main Config.TCU Module Configs"=w888:T50[])
        n334 = property class="VI"() -> ("Front Panel.Title"=w887:string)  [unwired: 2 in, 2 out]
        n335 = for {
          shift-right: [w906] -> w890
          shift-left: w889 -> [w905]
          tunnel: w888 -> [w902] mode=indexing
          tunnel: w887 -> [w899]
          tunnel: w886 -> [w897]
          shift-right: [w896] -> w883
          shift-left: w885 -> [w895]
          # "TCU Module (Main).vit"
          n336 = vi-ref "TCU Module.lvlib:TCU Module (Main).vi"() -> (w894:refnum<vi>)
          n337 = To Variant(anything=w902) -> (Variant=w903:variant)
          n338 = Unbundle By Name(w902) -> ("Process Name"=w901:string, "Drop Coords"=w898:T10)
          n339 = property class="VI"(reference=w894) -> ("Path"=w893:path)  [unwired: 1 in, 2 out]
          n340 = Bundle By Name(cluster=T82 {"Module VI Filepath"=path "", "Process Name"="", "Main UI Message Queue"=refnum, "Drop Coords"={"Horizontal"=0, "Vertical"=0}, "Module Parameters"=variant, "Name of Parent Window"=""} ("Drop Parameters"), "Module VI Filepath"=w893, "Module Parameters"=w903, "Process Name"=w901, "Main UI Message Queue"=w897, "Drop Coords"=w898, "Name of Parent Window"=w899) -> (w900:T82)
          n341 = call "Drop Start VI.vi"("error in (no error)"=w895, "Drop Parameters"=w900, "State in"=w905) -> ("error out"=w896:errorcluster, "State out"=w906:T1)  [unwired: 7 in]
          n342 = call "Next Instance Number.vi"("Module Type"=Module_Type_Enum."TCU", "Operation"=Module_Instance_Number_Operation_Enum."Next Instance Number") -> ()  [unwired: 8 in, 2 out]
        }
        n343 = call "Write to Log File.vi"("error in"=w883, "text"="Main: Update Config (TCU)") -> ()  [unwired: 9 in, 1 out]
      }
      frame "Update Config (Scale)" {
        # "Create Scale Modules and \"drop\" them on the Picture Control and assign configs"
        n344 = Unbundle By Name(w913) -> ("Main Config.Scale Module Configs"=w912:T42[])
        n345 = property class="VI"() -> ("Front Panel.Title"=w911:string)  [unwired: 2 in, 2 out]
        n346 = for {
          shift-right: [w930] -> w914
          shift-left: w913 -> [w929]
          tunnel: w912 -> [w926] mode=indexing
          tunnel: w911 -> [w923]
          tunnel: w910 -> [w921]
          shift-right: [w920] -> w907
          shift-left: w909 -> [w919]
          # "Scale Module (Main).vit"
          n347 = vi-ref "Scale Module (Main).vi"() -> (w918:refnum<vi>)
          n348 = To Variant(anything=w926) -> (Variant=w927:variant)
          n349 = Unbundle By Name(w926) -> ("Process Name"=w925:string, "Drop Coords"=w922:T10)
          n350 = property class="VI"(reference=w918) -> ("Path"=w917:path)  [unwired: 1 in, 2 out]
          n351 = Bundle By Name(cluster=T82 {"Module VI Filepath"=path "", "Process Name"="", "Main UI Message Queue"=refnum, "Drop Coords"={"Horizontal"=0, "Vertical"=0}, "Module Parameters"=variant, "Name of Parent Window"=""} ("Drop Parameters"), "Module VI Filepath"=w917, "Module Parameters"=w927, "Process Name"=w925, "Main UI Message Queue"=w921, "Drop Coords"=w922, "Name of Parent Window"=w923) -> (w924:T82)
          n352 = call "Drop Start VI.vi"("error in (no error)"=w919, "Drop Parameters"=w924, "State in"=w929) -> ("error out"=w920:errorcluster, "State out"=w930:T1)  [unwired: 7 in]
          n353 = call "Next Instance Number.vi"("Module Type"=Module_Type_Enum."Scale", "Operation"=Module_Instance_Number_Operation_Enum."Next Instance Number") -> ()  [unwired: 8 in, 2 out]
        }
        n354 = call "Write to Log File.vi"("error in"=w907, "text"="Main: Update Config (Scale)") -> ()  [unwired: 9 in, 1 out]
      }
      frame "Update Config (Flow)" {
        # "Create Flow Modules and \"drop\" them on the Picture Control and assign configs"
        n355 = Unbundle By Name(w937) -> ("Main Config.Flow Module Configs"=w936:T48[])
        n356 = property class="VI"() -> ("Front Panel.Title"=w935:string)  [unwired: 2 in, 2 out]
        n357 = for {
          shift-right: [w954] -> w938
          shift-left: w937 -> [w953]
          tunnel: w936 -> [w950] mode=indexing
          tunnel: w935 -> [w947]
          tunnel: w934 -> [w945]
          shift-right: [w944] -> w931
          shift-left: w933 -> [w943]
          # "Flow Module (Main).vit"
          n358 = vi-ref "Flow Module.lvlib:Flow Module (Main).vi"() -> (w942:refnum<vi>)
          n359 = To Variant(anything=w950) -> (Variant=w951:variant)
          n360 = Unbundle By Name(w950) -> ("Process Name"=w949:string, "Drop Coords"=w946:T10)
          n361 = property class="VI"(reference=w942) -> ("Path"=w941:path)  [unwired: 1 in, 2 out]
          n362 = Bundle By Name(cluster=T82 {"Module VI Filepath"=path "", "Process Name"="", "Main UI Message Queue"=refnum, "Drop Coords"={"Horizontal"=0, "Vertical"=0}, "Module Parameters"=variant, "Name of Parent Window"=""} ("Drop Parameters"), "Module VI Filepath"=w941, "Module Parameters"=w951, "Process Name"=w949, "Main UI Message Queue"=w945, "Drop Coords"=w946, "Name of Parent Window"=w947) -> (w948:T82)
          n363 = call "Drop Start VI.vi"("error in (no error)"=w943, "Drop Parameters"=w948, "State in"=w953) -> ("error out"=w944:errorcluster, "State out"=w954:T1)  [unwired: 7 in]
          n364 = call "Next Instance Number.vi"("Module Type"=Module_Type_Enum."Flow", "Operation"=Module_Instance_Number_Operation_Enum."Next Instance Number") -> ()  [unwired: 8 in, 2 out]
        }
        n365 = call "Write to Log File.vi"("error in"=w931, "text"="Main: Update Config (Flow)") -> ()  [unwired: 9 in, 1 out]
      }
      frame "Update Config (SC)" {
        # "Create Sonicator Modules and \"drop\" them on the Picture Control and assign configs"
        n366 = Unbundle By Name(w961) -> ("Main Config.SC Module Configs"=w960:T68[])
        n367 = property class="VI"() -> ("Front Panel.Title"=w959:string)  [unwired: 2 in, 2 out]
        n368 = for {
          shift-right: [w978] -> w962
          shift-left: w961 -> [w977]
          tunnel: w960 -> [w974] mode=indexing
          tunnel: w959 -> [w971]
          tunnel: w958 -> [w969]
          shift-right: [w968] -> w955
          shift-left: w957 -> [w967]
          # "Sonicator Module (Main).vit"
          n369 = vi-ref "Sonicator Module.lvlib:Sonicator Module (Main).vi"() -> (w966:refnum<vi>)
          n370 = To Variant(anything=w974) -> (Variant=w975:variant)
          n371 = Unbundle By Name(w974) -> ("Process Name"=w973:string, "Drop Coords"=w970:T10)
          n372 = property class="VI"(reference=w966) -> ("Path"=w965:path)  [unwired: 1 in, 2 out]
          n373 = Bundle By Name(cluster=T82 {"Module VI Filepath"=path "", "Process Name"="", "Main UI Message Queue"=refnum, "Drop Coords"={"Horizontal"=0, "Vertical"=0}, "Module Parameters"=variant, "Name of Parent Window"=""} ("Drop Parameters"), "Module VI Filepath"=w965, "Module Parameters"=w975, "Process Name"=w973, "Main UI Message Queue"=w969, "Drop Coords"=w970, "Name of Parent Window"=w971) -> (w972:T82)
          n374 = call "Drop Start VI.vi"("error in (no error)"=w967, "Drop Parameters"=w972, "State in"=w977) -> ("error out"=w968:errorcluster, "State out"=w978:T1)  [unwired: 7 in]
          n375 = call "Next Instance Number.vi"("Module Type"=Module_Type_Enum."Flow", "Operation"=Module_Instance_Number_Operation_Enum."Next Instance Number") -> ()  [unwired: 8 in, 2 out]
        }
        n376 = call "Write to Log File.vi"("error in"=w955, "text"="Main: Update Config (Flow)") -> ()  [unwired: 9 in, 1 out]
      }
      frame "Update Config (Decoration)" {
        # "Display all decorations (e.g. arrows, lines) that are in the campaign. Get the image path for the decoration and raw them on the canvas."
        n377 = Unbundle By Name(w982) -> ("Main Config.Decoration Module Configs"=w983:T47[])
        n378 = property class="VI"() -> ("Front Panel.Title"=w984:string)  [unwired: 2 in, 2 out]
        n379 = Current VI's Path() -> (path=w985:path)
        n380 = call "Image Folder.vi"("Main VI path"=w985) -> ("Image Folder path"=w986:path)  [unwired: 10 in]
        n381 = for "For every decoration (e.g. arrows, lines)" {
          tunnel: w983 -> [w997] mode=indexing
          tunnel: w984 -> [_]
          shift-right: [w987] -> w979
          shift-left: w981 -> [w987]
          tunnel: w986 -> [w990]
          # "Use relative path of\nthe image in case\nthe image folder has\nchanged."
          n382 = Unbundle By Name(w997) -> ("Decoration Filepath"=w991:path, "Drop Coords"=w992:T10)
          n383 = Strip Path(path=w991) -> (name=w989:string)  [unwired: 1 out]
          n384 = Build Path(base path=w990, name or relative path=w989) -> (appended path=w988:path)
          n385 = Unbundle By Name(w992) -> ("Horizontal"=w994:i32, "Vertical"=w993:i32)
          n386 = local read "Canvas"() -> (w996:picture)
          n387 = call "Draw BMP at Location.vi"("top"=w993, "left"=w994, "selected path"=w988, "picture in"=w996) -> ("picture out"=w995:picture)  [unwired: 5 in, 2 out]
          n388 = local write "Canvas"(w995) -> ()
        }
        n389 = call "Write to Log File.vi"("error in"=w979, "text"="Main: Update Config (Decoration)") -> ()  [unwired: 9 in, 1 out]
      }
      frame "Drag Start" {
        n390 = Variant To Data(error in=w1012, type=T73 {"Mouse Position"={"X"=0, "Y"=0}, "Mouse Modifiers"={"Button Down"=FALSE, "Shift Mod"=FALSE, "Menu Mod"=FALSE, "Option Mod"=FALSE}} ("Mouse"), Variant=w1011) -> (data=w1006:T73, error out=w1010:errorcluster)
        n391 = Unbundle By Name(w1006) -> ("Mouse Position"=w1005:cluster{"X":i32, "Y":i32})
        n392 = Unbundle By Name(w1003) -> ("[Thumbnails]"=w1009:T2[])
        n393 = call "Which Thumbnail.vi"("error in (no error)"=w1010, "Coords"=w1005, "[Thumbnails]"=w1009) -> ("error out"=w1000:errorcluster, "Path"=→"Path":path, "index of element"=w999:i32)  [unwired: 6 in]
        "index of element" <- w999
        n394 = call "Palette Cursors.vi"("error in (no error)"=w1000, "Index"=w999) -> ("error out"=w1001:errorcluster, "cursor ID"=w1002:refnum<k1>)  [unwired: 7 in, 1 out]
        n395 = Bundle By Name(cluster=w1003, "Drag Object Idx"=w999) -> (w1004:T1)
        n396 = call-poly <vilib>:"Set Cursor.vi"("error in (no error)"=w1001, "cursor ID"=w1002) -> ("error out"=w998:errorcluster)  [unwired: 8 in, 1 out]
      }
      frame "Drop" {
        (unwired) T73 {"Mouse Position"={"X"=0, "Y"=0}, "Mouse Modifiers"={"Button Down"=FALSE, "Shift Mod"=FALSE, "Menu Mod"=FALSE, "Option Mod"=FALSE}} ("Mouse")
        n397 = Variant To Data(error in=w1027, type=cluster{"Coords":T10, "Mouse":T73} {"Coords"={"Horizontal"=0, "Vertical"=0}, "Mouse"={"Mouse Position"={"X"=0, "Y"=0}, "Mouse Modifiers"={"Button Down"=FALSE, "Shift Mod"=FALSE, "Menu Mod"=FALSE, "Option Mod"=FALSE}}} ("output cluster"), Variant=w1029) -> (data=w1024:cluster{"Coords":T10, "Mouse":T73}, error out=w1028:errorcluster)
        n398 = Unbundle By Name(w1026) -> ("Drag Object Idx"=w1025:i32, "Drop Offset"=w1022:T6)
        n399 = Unbundle By Name(w1024) -> ("Mouse.Mouse Position"=w1023:cluster{"X":i32, "Y":i32})
        "Mouse Position" <- w1023
        n400 = case shown="Default" w1025 {
          selector: w1025 -> [_ w1039]
          tunnel: w1026 -> [w1032 w1037]
          tunnel: [w1032 w1042] -> w1014
          tunnel: [w1031 w1041] -> w1019
          tunnel: w1028 -> [w1031 w1040]
          tunnel: w1023 -> [_ w1036]
          tunnel: w1022 -> [_ _]
          tunnel: w1020 -> [_ w1035]
          tunnel: [T82 {"Module VI Filepath"=path "", "Process Name"="Error", "Main UI Message Queue"=refnum, "Drop Coords"={"Horizontal"=0, "Vertical"=0}, "Module Parameters"=variant, "Name of Parent Window"=""} ("Drop Parameters") w1033] -> w1013
          frame -1 {
          }
          frame Default {
            n401 = call "Thumbnail Path.vi"("Drag Object Idx"=w1039, "Cluster"=w1037) -> ("Module Type"=w1034:T80, "Thumbnail Path"=w1038:path)  [unwired: 8 in]
            n402 = case "Module Type?" shown="\"Feed\"..\"SC\"" w1034 {
              selector: w1034 -> [_ w1056]
              tunnel: [w1046 w1065] -> w1042
              tunnel: [w1050 w1064] -> w1041
              tunnel: w1040 -> [w1050 w1061]
              tunnel: w1036 -> [w1048 w1060]
              tunnel: w1038 -> [w1045 _]
              tunnel: w1037 -> [w1047 w1058]
              tunnel: w1035 -> [w1044 w1059]
              tunnel: [T82 {"Module VI Filepath"=path "", "Process Name"="Error", "Main UI Message Queue"=refnum, "Drop Coords"={"Horizontal"=0, "Vertical"=0}, "Module Parameters"=variant, "Name of Parent Window"=""} ("Drop Parameters") w1055] -> w1033
              frame "<unknown module>" {
                # "Non functional module (i.e. decoration like an arrow or line) has been dropped\nby the user. Save the filepath of the image being drawn and the coordinates into the\ncampaign configuration so it can be saved and recalled later."
                n403 = property class="VI"() -> ("Front Panel.Title"=w1049:string)  [unwired: 2 in, 2 out]
                n404 = call "Drop Decoration Parameters.vi"("Main UI Message Queue"=w1044, "Mouse Position"=w1048, "Parent Window Title"=w1049, "Path to Decoration image"=w1045, "State in"=w1047) -> ("State out"=w1046:T1)  [unwired: 4 in, 2 out]
                n405 = local read "Canvas"() -> (w1054:picture)
                n406 = Unbundle By Name(w1048) -> ("X"=w1052:i32, "Y"=w1051:i32)
                n407 = call "Draw BMP at Location.vi"("top"=w1051, "left"=w1052, "selected path"=w1045, "picture in"=w1054) -> ("picture out"=w1053:picture)  [unwired: 5 in, 2 out]
                n408 = local write "Canvas"(w1053) -> ()
              }
              frame "Feed".."SC" {
                n409 = property class="VI"() -> ("Front Panel.Title"=w1057:string)  [unwired: 2 in, 2 out]
                n410 = call "Drop Parameters.vi"("Main UI Message Queue"=w1059, "Mouse Position"=w1060, "error in (no error)"=w1061, "Parent Window Title"=w1057, "Module Type"=w1056, "State in"=w1058) -> ("error out"=w1062:errorcluster, "Drop Parameters"=w1055:T82, "State out"=w1063:T1)  [unwired: 3 in]
                n411 = call "Drop Start VI.vi"("error in (no error)"=w1062, "Drop Parameters"=w1055, "State in"=w1063) -> ("error out"=w1064:errorcluster, "State out"=w1065:T1)  [unwired: 7 in]
              }
            }
          }
        }
        n412 = Unbundle By Name(w1013) -> ("Process Name"=w1016:string)
        n413 = Concatenate Strings("Main: " ("string"), w1016, " Dropped" ("text")) -> (w1018:string)
        n414 = call "Write to Log File.vi"("error in"=w1019, "text"=w1018) -> ()  [unwired: 9 in, 1 out]
      }
      frame "E-Stop" {
        # "Stop the VI?"
        # "Tell all the modules to do E-Stop"
        n415 = call "E-Stop.vi"("State in"=w1071) -> ("error out"=w1069:errorcluster, "State out"=w1070:T1)  [unwired: 9 in]
        n416 = Merge Errors(w1069, w1068) -> (w1066:errorcluster)
        n417 = call "Write to Log File.vi"("error in"=w1066, "text"="Main: E-STOP Activated") -> ()  [unwired: 9 in, 1 out]
      }
      frame "Error" {
        w1082 = T90 1 items=["no dialog", "OK message", "continue or stop message", "OK message + warnings", "continue/stop + warnings"] ("type of dialog (OK msg:1)")
        # "Error - Check the error message data and respond accordingly. This message is sent by the \"Error Handler\" VIs at the end of each loop in this application."
        n418 = Variant To Data(type=errorcluster {"status"=FALSE, "code"=0, "source"=""} ("error out"), Variant=w1087) -> (data=w1081:errorcluster, error out=w1080:errorcluster)  [unwired: 1 in]
        n419 = Merge Errors(w1081, w1080) -> (w1079:errorcluster)
        "data" <- w1079
        n420 = call <vilib>:"General Error Handler.vi"("type of dialog (OK msg:1)"=w1082, "error in (no error)"=w1079) -> ("message"=w1073:string, "error out"=w1075:errorcluster)  [unwired: 9 in, 3 out]
        n421 = disable-structure shown="Enabled" {
          disable-tunnel: w1085 -> [w1091 _]
          disable-tunnel: [w1088 _] -> w1084
          disable-tunnel: w1075 -> [_ _]
          frame Disabled {
            n422 = call-poly "Enqueue Message.vi"("Priority Message? (F)"=TRUE, "Message"="Exit", "Message Queue"=w1091) -> ("error out"=w1088:errorcluster)  [unwired: 7 in, 1 out]
          }
          frame Enabled {
            # "If infinite error loop, slow it down\nso user can exit"
            n423 = Wait (ms)(milliseconds to wait=u32 2000) -> ()  [unwired: 1 out]
          }
        }
        n424 = Merge Errors(w1084, w1080) -> (w1078:errorcluster)
        n425 = call <vilib>:"Clear Errors.vi"("error in (no error)"=w1078) -> ("error out"=w1077:errorcluster)  [unwired: 5 in, 1 out]
        n426 = Concatenate Strings("Main: Error in Main: " ("text"), w1073) -> (w1074:string)
        n427 = call "Write to Log File.vi"("error in"=w1077, "text"=w1074) -> ()  [unwired: 9 in, 1 out]
        "Message Data" <- w1087
      }
      frame "Exit" {
        # "Stop and close the dynamically launched modules\n(e.g. Feed Modules)"
        # "Don't stop the VI quite yet. Wait for the DAQ to\nstop so we can delete the tags/shared variables."
        # "Exit - Fire the User Event to stop the Event Handling Loop.  Also send Exit messages to the Acquisition and Logging loops."
        n428 = call "Fire User Event - Stop.vi"("User Event - Stop"=w1123) -> ("error out"=w1102:errorcluster)  [unwired: 10 in]
        n429 = Unbundle By Name(w1122) -> ("Waveform Loop"=w1118:refnum<queue>, "CSV Log"=w1121:refnum<queue>, "TDMS Log"=w1120:refnum<queue>, "Graphs"=w1105:refnum<queue>[], "DAQ"=w1108:refnum<queue>, "Sequence"=w1104:refnum<queue>)
        n430 = call "Palette Cursors.vi"() -> ("error out"=w1115:errorcluster, "Cursor IDs out"=w1116:refnum<k1>[])  [unwired: 9 in, 1 out]
        n431 = for {
          tunnel: w1116 -> [w1129] mode=indexing
          shift-right: [w1126] -> w1114
          shift-left: w1115 -> [w1128]
          n432 = call <vilib>:"Destroy Cursor.vi"("cursor ID"=w1129, "error in (no error)"=w1128) -> ("error out"=w1127:errorcluster)  [unwired: 8 in]
          n433 = call <vilib>:"Clear Errors.vi"("error in (no error)"=w1127) -> ("error out"=w1126:errorcluster)  [unwired: 5 in, 1 out]
        }
        n434 = Build Array (concatenate)(w1118, w1121, w1120, w1105, w1104) -> (w1119:refnum<queue>[])
        n435 = for "stop and close support VIs" {
          tunnel: w1119 -> [w1134] mode=indexing
          tunnel: [w1132] -> w1113 mode=indexing
          tunnel: w1102 -> [w1130]
          n436 = call-poly "Enqueue Message.vi"("error in (no error)"=w1130, "Message"="Stop", "Message Queue"=w1134) -> ("error out"=w1131:errorcluster, "dup Message Queue"=w1135:refnum<queue>)  [unwired: 7 in]
          n437 = call-poly "Enqueue Message.vi"("error in (no error)"=w1131, "Message"="Exit", "Message Queue"=w1135) -> ("error out"=w1132:errorcluster)  [unwired: 7 in, 1 out]
        }
        n438 = call-poly "Enqueue Message.vi"("Priority Message? (F)"=TRUE, "Message"="DAQ-Exit", "Message Queue"=w1108) -> ("error out"=w1110:errorcluster)  [unwired: 7 in, 1 out]
        n439 = Merge Errors(w1102, w1113, w1110) -> (w1112:errorcluster)
        n440 = call "Close VIs.vi"("error in (no error)"=w1112, "State in"=w1111) -> ("error out"=w1106:errorcluster, "State out"=w1093:T1)  [unwired: 8 in]
        n441 = flat-sequence {
          tunnel: w1106 -> [_]
          frame #0 {
            n442 = call "Tag FGV.vi"("Operation"=Tag_FGV_Operation_Enum."Delete All Tags") -> ()  [unwired: 7 in, 8 out]
          }
        }
        n443 = local read "CSV Log File"() -> (w1101:path)
        n444 = Strip Path(path=w1101) -> (stripped path=w1098:path, name=w1094:string)
        n445 = Strip Path(path=w1098) -> (stripped path=w1097:path)  [unwired: 1 out]
        n446 = Build Path(base path=w1097, name or relative path="SDC") -> (appended path=w1095:path)
        n447 = Merge Errors(w1107, w1106, w1114) -> (w1099:errorcluster)
        n448 = Build Path(base path=w1095, name or relative path=w1094) -> (appended path=w1100:path)
        n449 = Copy(10:w1100, 11:w1101) -> ()  [unwired: 3 in, 3 out]
        n450 = call "Write to Log File.vi"("error in"=w1099, "text"="Main: Exited") -> ()  [unwired: 9 in, 1 out]
      }
      frame "File-Settings" {
        # "Get the Process Name from the settings dialog"
        n451 = call "File-Settings-Dialog.vi"("error in (no error)"=w1142) -> ("error out"=w1138:errorcluster, "Process Name Out"=w1140:string)  [unwired: 9 in]
        n452 = Bundle By Name(cluster=w1141, "Process Name"=w1140) -> (w1137:T1)
        n453 = call "Write to Log File.vi"("error in"=w1138, "text"="Main: File-Settings") -> ()  [unwired: 9 in, 1 out]
      }
      frame "Initialize" {
        (unwired) "Thumbnail (Feed Module).bmp" ("name or relative path")
        # "Initialize - Get configuration settings, then message the UI to initialize, and broadcast the settings to the other message loops."
        n454 = call "Empty Picture"() -> ("empty picture"=w1175:picture)
        n455 = local write "Canvas"(w1175) -> ()
        n456 = call-poly "Enqueue Message.vi"("error in (no error)"=w1154, "Message"="New Document", "Message Queue"=w1155) -> ("error out"=w1147:errorcluster)  [unwired: 7 in, 1 out]
        n457 = property on="Start Log" class="Bool"("DisabledEnum"=T83."Enabled" ("Disabled")) -> ()  [unwired: 2 in, 2 out]
        n458 = property on="Pause Log Button" class="Bool (strict)"("DisabledEnum"=T83."Disabled and Grayed Out" ("Disabled")) -> ()  [unwired: 2 in, 2 out]
        n459 = property on="Palette" class="Pict"("DisabledEnum"=T83."Enabled" ("Disabled")) -> ()  [unwired: 2 in, 2 out]
        n460 = property class="VI"() -> ("Front Panel.PanelBounds"=w1167:T4, "Front Panel.WinBounds"=w1166:T4)  [unwired: 2 in, 2 out]
        "Front Panel Window:Panel Bounds" <- w1167
        n461 = property class="VI"() -> ("Panel"=w1160:refnum<vi>)  [unwired: 2 in, 2 out]
        n462 = Current VI's Path() -> (path=w1179:path)
        n463 = property on="Canvas" class="Pict"() -> ("Position"=w1165:T6)  [unwired: 2 in, 2 out]
        "Position" <- w1165
        n464 = property class="Pnl"(reference=w1160) -> ("Panes[]"=w1161:refnum<vi>[])  [unwired: 1 in, 2 out]
        n465 = call "Next Instance Number.vi"("Operation"=Module_Instance_Number_Operation_Enum."Init") -> ()  [unwired: 9 in, 2 out]
        n466 = disable-structure shown="Default" {
          disable-tunnel: w1179 -> [w1183 _]
          disable-tunnel: [w1182 w1184] -> w1148
          frame condition #0 (active) {
            n467 = Strip Path(path=w1183) -> (stripped path=w1182:path)  [unwired: 1 out]
          }
          frame condition #1 {
            n468 = Default Directory() -> (w1184:path)
          }
        }
        n469 = Index Array(array=w1161) -> (element=w1162:refnum<vi>)  [unwired: 1 in]
        n470 = property class="Pane"(reference=w1162) -> ("Origin"=w1163:T72)  [unwired: 1 in, 2 out]
        "Origin" <- w1163
        n471 = Build Path(base path=w1148, name or relative path="Images") -> (appended path=w1180:path)
        n472 = Subtract(x=w1166, y=w1167) -> (x-y=w1168:T4)
        "x-y" <- w1168
        n473 = Negate(x=w1163) -> (-x=w1164:T72)
        n474 = call "Load Palette Images.vi"("Palette Image Folder"=w1180) -> ("error out"=w1152:errorcluster, "Cursor IDs"=w1151:refnum<k1>[], "[Thumbnails]"=w1176:T2[], "new picture"=→"Palette":picture)  [unwired: 7 in]
        n475 = Unbundle By Name(w1168) -> ("Top"=w1169:i16)
        n476 = Add(x=w1164, y=w1165) -> (x+y=w1172:T6)
        n477 = Unbundle By Name(w1172) -> ("Top"=w1170:i32)
        n478 = Negate(x=w1169) -> (-x=w1173:i16)
        n479 = Add(x=w1173, y=w1170) -> (x+y=w1171:i32)
        n480 = Bundle By Name(cluster=w1172, "Top"=w1171) -> (w1159:T6)
        "Drop Offset" <- w1159
        n481 = call "Palette Cursors.vi"("error in (no error)"=w1152, "Initialize"=TRUE, "Cursor IDs in"=w1151) -> ()  [unwired: 6 in, 3 out]
        n482 = Bundle By Name(cluster=w1143, "[Thumbnails]"=w1176, "Active Object"=-1, "Drop Offset"=w1159, "Main Config.Cycle Period"=1.0) -> (w1177:T1)
        n483 = call "Write to Log File.vi"("error in"=w1147, "text"="Main: Initialized") -> ("error out"=w1146:errorcluster)  [unwired: 9 in]
      }
      frame "New Document" {
        # "Start DAQ. Don't wait for Start Log"
        # "DAQ task is cleared here"
        # "Reset all the tags."
        # "Called from initialize at the start of a run"
        n484 = call "Tag FGV.vi"("Operation"=Tag_FGV_Operation_Enum."Read All Tags", "error in (no error)"=w1191) -> ("error out"=w1192:errorcluster)  [unwired: 6 in, 7 out]
        n485 = call "Empty Picture"() -> ("empty picture"=w1194:picture)
        n486 = call "Tag FGV.vi"("Operation"=Tag_FGV_Operation_Enum."Init", "error in (no error)"=w1192) -> ("error out"=w1196:errorcluster)  [unwired: 6 in, 7 out]
        n487 = local write "Canvas"(w1194) -> ()
        n488 = call-poly "Enqueue Message.vi"("error in (no error)"=w1196, "Message"="DAQ-Initialize", "Message Queue"=w1195) -> ("error out"=w1188:errorcluster, "dup Message Queue"=w1189:refnum<queue>)  [unwired: 7 in]
        n489 = call-poly "Enqueue Message.vi"("error in (no error)"=w1188, "Message"="DAQ-Start", "Message Queue"=w1189) -> ("error out"=w1186:errorcluster)  [unwired: 7 in, 1 out]
        n490 = call "Write to Log File.vi"("error in"=w1186, "text"="Main: New Document") -> ("error out"=w1185:errorcluster)  [unwired: 9 in]
      }
      frame "Open Campaign" {
        # "Choose a saved campaign to load"
        # "Load a Campaign from a previous save"
        n491 = Unbundle By Name(w1205) -> ("Main Config"=w1216:T7, "Campaign Filepath"=w1209:path)
        n492 = call "Application Data Folder.vi"() -> ("Campaign Folder"=w1208:path)  [unwired: 7 in, 4 out]
        n493 = Empty String/Path?(string/path=w1209) -> (empty?=w1210:bool)
        n494 = Select(t=w1208, s=w1210, f=w1209) -> (s? t:f=w1207:path)
        n495 = call "File Dialog3"("start path"=w1207, "prompt"="Open campaign", "error in"=w1215, "pattern (all files)"="*.cfg") -> ("selected path"=w1213:path, "cancelled"=w1214:bool, "error out"=w1204:errorcluster)  [unwired: 8 in, 1 out]
        n496 = call <vilib>:"Clear Errors.vi"("error in (no error)"=w1204) -> ("error out"=w1203:errorcluster)  [unwired: 5 in, 1 out]
        n497 = case shown="False" w1214 {
          tunnel: w1216 -> [w1226 _]
          tunnel: w1203 -> [w1220 w1244]
          tunnel: [w1233 w1244] -> w1200
          tunnel: w1213 -> [w1237 _]
          tunnel: w1205 -> [w1228 w1243]
          tunnel: [w1235 w1243] -> w1206
          tunnel: w1202 -> [w1231 _]
          tunnel: w1201 -> [w1219 _]
          frame False {
            # "After the DAQ has executed its configuration, it will call the next case,\ni.e. Open Campaign-DAQ Commited\"\nwhich queues additional messages."
            # "close previously\nopened dynamic VIs"
            n498 = call "Empty Picture"() -> ("empty picture"=w1223:picture)
            n499 = call-poly "Enqueue Message.vi"("error in (no error)"=w1220, "Message"="DAQ-Stop", "Message Queue"=w1219) -> ("error out"=w1221:errorcluster)  [unwired: 7 in, 1 out]
            n500 = local write "Canvas"(w1223) -> ()
            n501 = call "Close VIs.vi"("error in (no error)"=w1221, "State in"=w1228) -> ("error out"=w1225:errorcluster, "State out"=w1229:T1)  [unwired: 8 in]
            n502 = call <vilib>:"Clear Errors.vi"("error in (no error)"=w1225) -> ("error out"=w1224:errorcluster)  [unwired: 5 in, 1 out]
            n503 = call "Clear Dynamic Module Configs.vi"("Main Config in"=w1226) -> ("Main Config out"=w1227:T7)  [unwired: 8 in, 1 out]
            n504 = call "Read-Write Config File.vi"("configuration file path"=w1237, "Main Config in"=w1227, "Mode"=Config_File_Operation_Enum."Read", "error in"=w1224) -> ("Config File Path"=w1236:path, "Main Config out"=w1218:T7, "error out"=w1234:errorcluster)  [unwired: 4 in]
            n505 = Unbundle By Name(w1218) -> ("Notebook"=w1217:string)
            n506 = Bundle By Name(cluster=w1229, "Campaign Filepath"=w1236, "Config Changed?"=FALSE, "Main Config"=w1218) -> (w1235:T1)
            n507 = for {
              tunnel: w1231 -> [w1240]
              shift-right: [w1241] -> w1233
              shift-left: w1234 -> [w1242]
              tunnel: string[] ["New Document", "Update Config (DAQ)"] -> [w1239] mode=indexing
              n508 = call-poly "Enqueue Message.vi"("error in (no error)"=w1242, "Message"=w1239, "Message Queue"=w1240) -> ("error out"=w1241:errorcluster)  [unwired: 7 in, 1 out]
            }
            n509 = property on="Notebook" class="Str"("Val(Sgnl)"=w1217) -> ()  [unwired: 2 in, 2 out]
          }
          frame True {
          }
        }
      }
      frame "Open Campaign-DAQ Commited" {
        # "Wait for DAQ Message Loop to commit its tags/shared variables before starting up the dynamic modules so that the dynamic modules that bind to tags/shared variables in the DAQ task will not error."
        n510 = for {
          tunnel: w1249 -> [w1251]
          shift-right: [w1252] -> w1245
          shift-left: _ -> [w1253]
          tunnel: string[] ["Update Config (TT)", "Update Config (Feed)", "Update Config (PT)", "Update Config (Pump)", "Update Config (Scale)", "Update Config (Flow)", "Update Config (U3)", "Update Config (Decoration)", "Update Config (TCU)", "Update Config (DO)", "Update Config (PR)", "Update Config (OPC)", "Update Config (SC)"] -> [w1250] mode=indexing
          n511 = call-poly "Enqueue Message.vi"("error in (no error)"=w1253, "Message"=w1250, "Message Queue"=w1251) -> ("error out"=w1252:errorcluster)  [unwired: 7 in, 1 out]
        }
        n512 = call "Write to Log File.vi"("error in"=w1245, "text"="Main: Campaign Opened") -> ()  [unwired: 9 in, 1 out]
      }
      frame "Read Config" {
        n513 = call "Read Main Config File.vi"("error in (no error)"=w1259) -> ("Main Config out"=w1256:T7, "error out"=w1254:errorcluster)  [unwired: 7 in, 1 out]
        n514 = Bundle By Name(cluster=w1257, "Main Config"=w1256) -> (w1258:T1)
        n515 = call "Write to Log File.vi"("error in"=w1254, "text"="Main: Read Config Completed") -> ()  [unwired: 9 in, 1 out]
      }
      frame "Save Campaign", "Save Campaign As" {
        n516 = local read "Notebook"() -> (w1261:string)
        n517 = Bundle By Name(cluster=w1262, "Main Config.Notebook"=w1261) -> (w1260:T1)
        n518 = Equal?(x=w1269, y="Save Campaign As") -> (x = y?=w1267:bool)
        n519 = call "Application Data Folder.vi"() -> ("Campaign Folder"=w1276:path)  [unwired: 7 in, 4 out]
        n520 = Unbundle By Name(w1260) -> ("Main Config"=w1277:T7, "Campaign Filepath"=w1271:path)
        n521 = Empty String/Path?(string/path=w1271) -> (empty?=w1266:bool)
        n522 = Or(x=w1266, y=w1267) -> (x .or. y?=w1265:bool)
        n523 = case shown="True" w1265 {
          tunnel: w1276 -> [_ w1288]
          tunnel: w1275 -> [w1280 w1285]
          tunnel: [w1280 w1281] -> w1274
          tunnel: [FALSE ("cancelled") w1284] -> w1273
          tunnel: [w1278 w1283] -> w1272
          tunnel: w1271 -> [w1278 _]
          frame False {
          }
          frame True {
            # "Choose a file name to save"
            n524 = call "File Dialog2"("start path"=w1288, "prompt"="Save campaign as", "error in"=w1285, "pattern (all files)"="*.cfg") -> ("selected path"=w1283:path, "cancelled"=w1284:bool, "error out"=w1282:errorcluster)  [unwired: 8 in, 1 out]
            n525 = call <vilib>:"Clear Errors.vi"("error in (no error)"=w1282) -> ("error out"=w1281:errorcluster)  [unwired: 5 in, 1 out]
          }
        }
        n526 = case shown="False" w1273 {
          tunnel: w1277 -> [w1295 _]
          tunnel: w1274 -> [w1294 w1298]
          tunnel: [w1293 w1298] -> w1263
          tunnel: w1272 -> [w1292 _]
          tunnel: w1260 -> [w1291 w1297]
          tunnel: [w1289 w1297] -> w1270
          frame False {
            n527 = call "Read-Write Config File.vi"("configuration file path"=w1292, "Main Config in"=w1295, "Mode"=Config_File_Operation_Enum."Write", "error in"=w1294) -> ("Config File Path"=w1290:path, "error out"=w1293:errorcluster)  [unwired: 4 in, 1 out]
            n528 = Bundle By Name(cluster=w1291, "Campaign Filepath"=w1290) -> (w1289:T1)
          }
          frame True {
          }
        }
        n529 = call "Write to Log File.vi"("error in"=w1263, "text"="Main: Campaign Saved") -> ()  [unwired: 9 in, 1 out]
      }
      frame "Start Log" {
        # "Set up the alarms, create the data and graphing files, create the data tags, and start the logging"
        n530 = Unbundle By Name(w1301) -> ("Process Name"=w1314:string)
        n531 = Unbundle By Name(w1315) -> ("Waveform Loop"=w1311:refnum<queue>, "CSV Log"=w1307:refnum<queue>)
        n532 = Unbundle By Name(w1301) -> ("Queues"=w1310:refnum<queue>[])
        n533 = Empty String/Path?(string/path=w1314) -> (empty?=w1313:bool)
        n534 = case "Is there a process name" shown="True" w1313 {
          tunnel: [w1376 w1381] -> w1306
          tunnel: w1314 -> [w1376 _]
          tunnel: [TRUE w1377] -> w1300
          frame False {
          }
          frame True {
            n535 = Empty String/Path?(string/path="Notebook") -> (empty?=w1378:bool)
            n536 = Concatenate Strings("Notebook", "" ("string")) -> (w1381:string)
            n537 = Not(x=w1378) -> (.not. x?=w1377:bool)
          }
        }
        n538 = Unbundle By Name(w1301) -> ("Main Config.Cycle Period"=w1299:dbl)
        n539 = Max & Min(x=w1299, y=1.0) -> (max(x,y)=w1304:dbl)  [unwired: 1 out]
        n540 = case shown="False" w1300 {
          tunnel: w1312 -> [w1316 w1343]
          tunnel: w1311 -> [_ w1339]
          tunnel: w1310 -> [_ w1338]
          tunnel: w1309 -> [_ w1337]
          tunnel: w1308 -> [_ w1336]
          tunnel: w1307 -> [_ w1332]
          tunnel: w1306 -> [_ w1331]
          tunnel: w1304 -> [_ w1326]
          tunnel: [w1316 w1325] -> w1303
          tunnel: w1302 -> [_ w1324]
          tunnel: w1301 -> [_ w1323]
          frame False {
            n541 = One Button Dialog(message="Enter a Notebook #") -> ()  [unwired: 1 in, 1 out]
          }
          frame True {
            w1320 = "Add Note" ("item name")
            w1328 = "Set Data Rate" ("item tag")
            # "Add the menu item when the Log is Started"
            # "The Cycle Rate cannot be changed mid run"
            n542 = call-poly "Enqueue Message.vi"("Message Data"=w1331, "Message"="Notebook", "Message Queue"=w1332) -> ()  [unwired: 7 in, 2 out]
            n543 = call "Logfile Paths.vi"("File Name"=w1331) -> ("Alarm CSV Logfile path"=w1340:path, "TDMS Logfile path"=w1349:path, "CSV Logfile path"=w1347:path)  [unwired: 8 in]
            "CSV Log File" <- w1347
            n544 = call-poly "Enqueue Message.vi"("Message Data"=w1323, "Message"="Start", "Message Queue"=w1324) -> ()  [unwired: 7 in, 2 out]
            n545 = Bundle By Name(cluster=T86 {"dt (seconds)"=0.1, "CSV Logfile path"=path "", "TDMS Logfile path"=path ""} ("Start Params"), "dt (seconds)"=w1326, "CSV Logfile path"=w1347, "TDMS Logfile path"=w1349) -> (w1348:T86)
            n546 = call "Log Alarm FGV.vi"("error in (no error)"=w1343, "Path"=w1340, "Operation"=Alarm_Log_Operation_Enum."Create Log") -> ("error out"=w1341:errorcluster)  [unwired: 8 in]
            n547 = flat-sequence {
              tunnel: w1338 -> [w1354]
              tunnel: w1341 -> [w1353]
              tunnel: [w1355] -> w1352
              tunnel: w1352 -> [w1364]
              tunnel: [w1363] -> w1351
              tunnel: w1337 -> [w1365]
              tunnel: w1323 -> [w1362]
              tunnel: w1351 -> [w1368]
              tunnel: w1348 -> [w1374]
              tunnel: w1339 -> [w1372]
              tunnel: [w1366] -> w1334
              tunnel: w1323 -> [w1370]
              tunnel: w1336 -> [w1369]
              frame #0 {
                n548 = for {
                  tunnel: w1354 -> [w1360] mode=indexing
                  tunnel: w1353 -> [w1359]
                  tunnel: [w1358] -> w1356 mode=indexing
                  n549 = call-poly "Enqueue Message.vi"("error in (no error)"=w1359, "Message"="Start Log", "Message Queue"=w1360) -> ("error out"=w1358:errorcluster)  [unwired: 7 in, 1 out]
                  n550 = Wait (ms)(milliseconds to wait=u32 250) -> ()  [unwired: 1 out]
                }
                n551 = Merge Errors(w1353, w1356) -> (w1355:errorcluster)
              }
              frame #1 {
                n552 = call "Check Module Tag Creation.vi"("error in (no error)"=w1364, "Cluster"=w1362, "UI"=w1365) -> ("error out"=w1363:errorcluster)  [unwired: 8 in]
              }
              frame #2 {
                n553 = call-poly "Enqueue Message.vi"("error in (no error)"=w1368, "Message Data"=w1370, "Message"="Log Settings", "Message Queue"=w1369) -> ("error out"=w1367:errorcluster)  [unwired: 6 in, 1 out]
                n554 = call-poly "Enqueue Message.vi"("error in (no error)"=w1367, "Message Data"=w1374, "Message"="Start", "Message Queue"=w1372) -> ("error out"=w1366:errorcluster)  [unwired: 6 in, 1 out]
              }
            }
            n555 = property on="Pause Log Button" class="Bool (strict)"("Val(Sgnl)"=FALSE ("Pause Log Button")) -> ()  [unwired: 2 in, 2 out]
            n556 = property on="Palette" class="Pict"("DisabledEnum"=T83."Disabled and Grayed Out" ("Disabled")) -> ()  [unwired: 2 in, 2 out]
            n557 = property on="Pause Log Button" class="Bool (strict)"("DisabledEnum"=T83."Enabled" ("Disabled")) -> ()  [unwired: 2 in, 2 out]
            n558 = property on="Start Log" class="Bool"("DisabledEnum"=T83."Disabled and Grayed Out" ("Disabled")) -> ()  [unwired: 2 in, 2 out]
            n559 = Current VI's Menubar() -> (w1321:refnum<k9>)
            n560 = Set Menu Item Info(7:w1320, 9:TRUE ("enabled"), 10:w1320, 11:w1321) -> ()  [unwired: 3 in, 2 out]
            n561 = Current VI's Menubar() -> (w1329:refnum<k9>)
            n562 = call "Tag FGV.vi"("Operation"=Tag_FGV_Operation_Enum."Enable All Alarms", "error in (no error)"=w1334) -> ("error out"=w1325:errorcluster)  [unwired: 6 in, 7 out]
            n563 = Set Menu Item Info(7:w1328, 9:FALSE ("enabled"), 10:w1328, 11:w1329) -> ()  [unwired: 3 in, 2 out]
            n564 = call "Write to Log File.vi"("error in"=w1325, "text"="Main: Data Log Started") -> ()  [unwired: 9 in, 1 out]
          }
        }
      }
      frame "Stop Log" {
        # "Stop Waveform loop,\nwhich stops the\nCSV Log and\nTDMS Log."
        # "Stop the logging"
        n565 = Unbundle By Name(w1393) -> ("Waveform Loop"=w1392:refnum<queue>)
        n566 = property on="Palette" class="Pict"("DisabledEnum"=T83."Enabled" ("Disabled")) -> ()  [unwired: 2 in, 2 out]
        n567 = call-poly "Enqueue Message.vi"("error in (no error)"=w1390, "Message"="Stop", "Message Queue"=w1392) -> ("error out"=w1388:errorcluster)  [unwired: 7 in, 1 out]
        n568 = property on="Start Log" class="Bool"("DisabledEnum"=T83."Enabled" ("Disabled")) -> ()  [unwired: 2 in, 2 out]
        n569 = property on="Pause Log Button" class="Bool (strict)"("DisabledEnum"=T83."Disabled and Grayed Out" ("Disabled")) -> ()  [unwired: 2 in, 2 out]
        n570 = call "Log Alarm FGV.vi"("error in (no error)"=w1388, "Operation"=Alarm_Log_Operation_Enum."Close Log") -> ("error out"=w1382:errorcluster)  [unwired: 9 in]
        n571 = call "Write to Log File.vi"("error in"=w1382, "text"="Main: Data Log Stopped") -> ()  [unwired: 9 in, 1 out]
      }
      frame "Timeout" {
        # "Prevent CPU from overloading in the case that this is called too often."
        n572 = Wait (ms)(milliseconds to wait=u32 5) -> ()  [unwired: 1 out]
      }
      frame "Launch Sequence Dialog" {
        # "Control the execution of the Sequencer"
        n573 = call "Sequence Dialog.vi"("error in (no error)"=w1408, "Sequence UI"=w1397, "State Cluster In"=w1401) -> ("error out"=w1404:errorcluster, "Start"=w1402:bool, "cancelled"=w1407:bool, "State Cluster Out"=w1406:T1, "Pause"=w1400:bool)  [unwired: 3 in, 1 out]
        n574 = case "Is it Cancelled?" shown="False" w1407 {
          tunnel: w1406 -> [w1415 _]
          tunnel: [w1415 w1435] -> w1405
          tunnel: w1404 -> [w1419 w1436]
          tunnel: w1403 -> [w1417 _]
          tunnel: [w1409 w1436] -> w1398
          tunnel: w1402 -> [w1416 _]
          tunnel: w1401 -> [_ w1435]
          tunnel: w1400 -> [w1414 _]
          frame False {
            n575 = call-poly "Enqueue Message.vi"("error in (no error)"=w1419, "Message Data"=w1415, "Message"="Update Sequence", "Message Queue"=w1417) -> ("error out"=w1410:errorcluster, "dup Message Queue"=w1411:refnum<queue>)  [unwired: 6 in]
            n576 = case "Is it Paused?" shown="True" w1414 {
              tunnel: w1410 -> [w1423 w1429]
              tunnel: [w1422 w1428] -> w1413
              tunnel: w1411 -> [w1421 w1427]
              tunnel: [w1420 w1425] -> w1412
              frame False {
                n577 = call-poly "Enqueue Message.vi"("error in (no error)"=w1423, "Message"="Resume Sequence", "Message Queue"=w1421) -> ("error out"=w1422:errorcluster, "dup Message Queue"=w1420:refnum<queue>)  [unwired: 7 in]
              }
              frame True {
                n578 = call-poly "Enqueue Message.vi"("error in (no error)"=w1429, "Message"="Pause Sequence", "Message Queue"=w1427) -> ("error out"=w1428:errorcluster, "dup Message Queue"=w1425:refnum<queue>)  [unwired: 7 in]
              }
            }
            n579 = case "Start?" shown="True" w1416 {
              tunnel: w1413 -> [w1430 w1434]
              tunnel: [w1430 w1433] -> w1409
              tunnel: w1412 -> [_ w1432]
              frame False {
              }
              frame True {
                n580 = call-poly "Enqueue Message.vi"("error in (no error)"=w1434, "Message"="Start Sequence", "Message Queue"=w1432) -> ("error out"=w1433:errorcluster)  [unwired: 7 in, 1 out]
              }
            }
          }
          frame True {
          }
        }
        n581 = call "Write to Log File.vi"("error in"=w1398, "text"="Main: Sequencer Opened") -> ()  [unwired: 9 in, 1 out]
      }
      frame "Launch Data Rate Dialog" {
        # "Control the execution of the Sequencer"
        n582 = call "Data Rate Dialog.vi"("error in (no error)"=w1440, 11:w1437) -> ("error out"=w1439:errorcluster, 3:w1438:T1)  [unwired: 8 in]
        n583 = call "Write to Log File.vi"("error in"=w1439, "text"="Main: Data Rate Dialog Opened") -> ()  [unwired: 9 in, 1 out]
      }
      frame "Launch TCP Setup Dialog" {
        # "Control the execution of the Sequencer"
        n584 = call "TCP Settings Dialog.vi"("Message Queues out"=w1445) -> ()  [unwired: 11 in]
        n585 = call "Write to Log File.vi"("error in"=w1444, "text"="Main: TCP Dialog Opened") -> ("error out"=w1443:errorcluster)  [unwired: 9 in]
      }
      frame "Reset Global Variables" {
        n586 = flat-sequence {
          tunnel: [w1465] -> w1454
          tunnel: w1449 -> [w1464]
          tunnel: w1454 -> [w1467]
          tunnel: [w1467] -> w1453
          tunnel: w1453 -> [w1469]
          tunnel: [w1468] -> w1450
          frame #0 {
            n587 = shared-variable ".\\Support Library.lvlib\\Globals.lvlib\\Ismatec 4083 Global"(T87 [{"Busy"=FALSE, "ChannelCnt"=0.0, "Initialized"=FALSE, "Current Channel"=0.0, "Initialized Channels"=[]}, {"Busy"=FALSE, "ChannelCnt"=0.0, "Initialized"=FALSE, "Current Channel"=0.0, "Initialized Channels"=[]}, {"Busy"=FALSE, "ChannelCnt"=0.0, "Initialized"=FALSE, "Current Channel"=0.0, "Initialized Channels"=[]}, {"Busy"=FALSE, "ChannelCnt"=0.0, "Initialized"=FALSE, "Current Channel"=0.0, "Initialized Channels"=[]}, {"Busy"=FALSE, "ChannelCnt"=0.0, "Initialized"=FALSE, "Current Channel"=0.0, "Initialized Channels"=[]}, {"Busy"=FALSE, "ChannelCnt"=0.0, "Initialized"=FALSE, "Current Channel"=0.0, "Initialized Channels"=[]}, {"Busy"=FALSE, "ChannelCnt"=0.0, "Initialized"=FALSE, "Current Channel"=0.0, "Initialized Channels"=[]}, {"Busy"=FALSE, "ChannelCnt"=0.0, "Initialized"=FALSE, "Current Channel"=0.0, "Initialized Channels"=[]}, {"Busy"=FALSE, "ChannelCnt"=0.0, "Initialized"=FALSE, "Current Channel"=0.0, "Initialized Channels"=[]}, {"Busy"=FALSE, "ChannelCnt"=0.0, "Initialized"=FALSE, "Current Channel"=0.0, "Initialized Channels"=[]}, {"Busy"=FALSE, "ChannelCnt"=0.0, "Initialized"=FALSE, "Current Channel"=0.0, "Initialized Channels"=[]}, {"Busy"=FALSE, "ChannelCnt"=0.0, "Initialized"=FALSE, "Current Channel"=0.0, "Initialized Channels"=[]}, {"Busy"=FALSE, "ChannelCnt"=0.0, "Initialized"=FALSE, "Current Channel"=0.0, "Initialized Channels"=[]}, {"Busy"=FALSE, "ChannelCnt"=0.0, "Initialized"=FALSE, "Current Channel"=0.0, "Initialized Channels"=[]}, {"Busy"=FALSE, "ChannelCnt"=0.0, "Initialized"=FALSE, "Current Channel"=0.0, "Initialized Channels"=[]}, {"Busy"=FALSE, "ChannelCnt"=0.0, "Initialized"=FALSE, "Current Channel"=0.0, "Initialized Channels"=[]}, {"Busy"=FALSE, "ChannelCnt"=0.0, "Initialized"=FALSE, "Current Channel"=0.0, "Initialized Channels"=[]}, {"Busy"=FALSE, "ChannelCnt"=0.0, "Initialized"=FALSE, "Current Channel"=0.0, "Initialized Channels"=[]}, {"Busy"=FALSE, "ChannelCnt"=0.0, "Initialized"=FALSE, "Current Channel"=0.0, "Initialized Channels"=[]}, {"Busy"=FALSE, "ChannelCnt"=0.0, "Initialized"=FALSE, "Current Channel"=0.0, "Initialized Channels"=[]}, {"Busy"=FALSE, "ChannelCnt"=0.0, "Initialized"=FALSE, "Current Channel"=0.0, "Initialized Channels"=[]}] ("Array"), error in=w1464) -> (error out=w1465:errorcluster)
          }
          frame #1 {
            n588 = Wait (ms)(milliseconds to wait=u32 100) -> ()  [unwired: 1 out]
          }
          frame #2 {
            n589 = shared-variable ".\\Support Library.lvlib\\Globals.lvlib\\Ismatec 4083 Global"(error in=w1469) -> (error out=w1468:errorcluster)  [unwired: 1 out]
          }
        }
        n590 = flat-sequence {
          tunnel: [w1458] -> w1452
          tunnel: w1449 -> [w1457]
          tunnel: w1452 -> [w1460]
          tunnel: [w1460] -> w1451
          tunnel: w1451 -> [w1462]
          tunnel: [w1461] -> w1448
          frame #0 {
            n591 = shared-variable ".\\Support Library.lvlib\\Globals.lvlib\\ASIA Pump Global"(T77 [{"Busy"=FALSE, "PumpCnt"=0.0, "RemoteEntered"=FALSE, "OverpressureSet"=FALSE}, {"Busy"=FALSE, "PumpCnt"=0.0, "RemoteEntered"=FALSE, "OverpressureSet"=FALSE}, {"Busy"=FALSE, "PumpCnt"=0.0, "RemoteEntered"=FALSE, "OverpressureSet"=FALSE}, {"Busy"=FALSE, "PumpCnt"=0.0, "RemoteEntered"=FALSE, "OverpressureSet"=FALSE}, {"Busy"=FALSE, "PumpCnt"=0.0, "RemoteEntered"=FALSE, "OverpressureSet"=FALSE}, {"Busy"=FALSE, "PumpCnt"=0.0, "RemoteEntered"=FALSE, "OverpressureSet"=FALSE}, {"Busy"=FALSE, "PumpCnt"=0.0, "RemoteEntered"=FALSE, "OverpressureSet"=FALSE}, {"Busy"=FALSE, "PumpCnt"=0.0, "RemoteEntered"=FALSE, "OverpressureSet"=FALSE}, {"Busy"=FALSE, "PumpCnt"=0.0, "RemoteEntered"=FALSE, "OverpressureSet"=FALSE}, {"Busy"=FALSE, "PumpCnt"=0.0, "RemoteEntered"=FALSE, "OverpressureSet"=FALSE}, {"Busy"=FALSE, "PumpCnt"=0.0, "RemoteEntered"=FALSE, "OverpressureSet"=FALSE}, {"Busy"=FALSE, "PumpCnt"=0.0, "RemoteEntered"=FALSE, "OverpressureSet"=FALSE}, {"Busy"=FALSE, "PumpCnt"=0.0, "RemoteEntered"=FALSE, "OverpressureSet"=FALSE}] ("ASIA Pump Global"), error in=w1457) -> (error out=w1458:errorcluster)
          }
          frame #1 {
            n592 = Wait (ms)(milliseconds to wait=u32 100) -> ()  [unwired: 1 out]
          }
          frame #2 {
            n593 = shared-variable ".\\Support Library.lvlib\\Globals.lvlib\\ASIA Pump Global"(error in=w1462) -> (error out=w1461:errorcluster)  [unwired: 1 out]
          }
        }
        n594 = Merge Errors(w1450, w1449, w1448) -> (w1447:errorcluster)
      }
      frame "Launch Calibration Dialog" {
        # "Run the Calibration Program"
        n595 = call "Calibration Main.vi"("error in (no error)"=w1474, "Pump Calibration Config in"=T89 {"Settings"={"Cycle Period"=500.0, "Ismatech"={"VISA resource name"="", "Simulated?"=TRUE, "Pump Number"=1.0, "Reverse?"=FALSE}, "Masterflex"={"VISA resource name"="", "Simulated?"=TRUE, "Pump Number"=1.0, "Reverse?"=FALSE}, "Bronkhorst M13 Settings"={"VISA resource name"="", "Simulated?"=TRUE, "Smoothing Steps"=1}, "PID 2 Parameters"={"Input Device"=enum."Default", "Output Device"=enum."Default"}, "Tacmina Settings"={"Analog DAQ Task"="", "Digital DAQ Task"=""}, "KNF SIMDOS Settings"={"VISA resource name"="", "Simulated?"=TRUE}, "VICI M50 Settings"={"VISA resource name"="", "Simulated?"=TRUE, "Pump Letter"="", "Reverse?"=FALSE}, "FLOM Settings"={"VISA resource name"="", "Simulated?"=TRUE, "Pump Number"=0.0}, "Calibration Limits"={"Minimum (ml/min)"=0.0, "Maximum (ml/min)"=0.0, "Steps"=0.0}, "SSI PR Settings"={"VISA resource name"="", "Simulated?"=FALSE}, "Ismatech 4308 Settings"={"VISA resource name"="", "Pump Number"=1, "Channel Number"=0, "Simulated?"=TRUE, "Reverse?"=FALSE}, "Bronkhorst M14 Settings"={"VISA resource name"="", "Simulated?"=FALSE, "Smoothing Steps"=1}}, "Flowmeter Output"=0.0, "Density"=0.0, "FL Temp"=0.0, "Speed %"=0.0, "File Refnum"=refnum, "Pump On?"=enum."Not Initialized"}) -> ("error out"=w1473:errorcluster)  [unwired: 8 in, 1 out]
        n596 = call "Write to Log File.vi"("error in"=w1473, "text"="Main: Calibration Opened") -> ("error out"=w1472:errorcluster)  [unwired: 9 in]
      }
      frame "Launch Note Dialog" {
        # "Open the dialog for adding notes to the data file"
        n597 = call-poly "Enqueue Message.vi"("error in (no error)"=w1480, "Message"="Add Note", "Message Queue"=w1481) -> ("error out"=w1476:errorcluster)  [unwired: 7 in, 1 out]
        n598 = call "Write to Log File.vi"("error in"=w1476, "text"="Main: Note Dialog Opened") -> ()  [unwired: 9 in, 1 out]
      }
      frame Default {
        # "'Default' case only runs if there is a message that isn't defined in any of the other cases.  Output a programming error."
        n599 = Concatenate Strings("The invalid message string " ("string"), w1483, " was received in Main." ("string")) -> (w1484:string)
        n600 = Bundle By Name(cluster=errorcluster {"status"=TRUE, "code"=1, "source"=""} ("error constant"), "source"=w1484) -> (w1482:errorcluster)
        n601 = call <vilib>:"General Error Handler.vi"("error in (no error)"=w1482) -> ("message"=w1488:string)  [unwired: 10 in, 4 out]
        n602 = Concatenate Strings("Main: Note Dialog Opened" ("text"), w1488) -> (w1489:string)
        n603 = call "Write to Log File.vi"("text"=w1489) -> ()  [unwired: 10 in, 1 out]
      }
      frame "Tags Created" {
        n604 = call "Write to Log File.vi"("error in"=w1492, "text"="Main: Tags Created") -> ()  [unwired: 9 in, 1 out]
      }
    }
    "Cluster" <- w111
    n605 = call "Error Handler - Message Handling Loop.vi"("error in (no error)"=w117, "Message Queue"=w115) -> ("dup error in"=w116:errorcluster, "dup Message Queue"=w109:refnum<queue>)  [unwired: 8 in]
  }
  n606 = Build Path(base path=w66, name or relative path="History Graph Message Loop.vi") -> (appended path=w65:path)
  n607 = Open VI Reference(vi path=w65) -> (vi reference=w72:refnum<vi>, error out=w70:errorcluster)  [unwired: 5 in]
  n608 = while {
    tunnel: w82 -> [w1497]
    tunnel: [w1506] -> w86
    shift-right: [w1504] -> w83
    shift-left: w47 -> [w1508]
    tunnel: w64 -> [w1496]
    shift-right: [w1502] -> _
    shift-left: T76 {"Down"=FALSE, "Mouse"={"Mouse Position"={"X"=0, "Y"=0}, "Mouse Modifiers"={"Button Down"=FALSE, "Shift Mod"=FALSE, "Menu Mod"=FALSE, "Option Mod"=FALSE}}, "Drag"=FALSE, "Canvas"=FALSE} -> [w1503]
    tunnel: w52 -> [w1500]
    tunnel: w51 -> [w1499]
    tunnel: w42 -> [w1495]
    stop <- w1505 stop-if-true
    # "Event Handling Loop"
    n609 = event shown="[12] Menu Selection (User)" {
      selector: w1508 -> [_ _ _ _ _ _ _ _ _ _ _ _ _ _ _ _ _]
      dyn-events: [_ _ _ _ _ _ _ _ _ _ _ _ _ _ _ _ _] -> w1504
      timeout: 1000 -> [_ _ _ _ _ _ _ _ _ _ _ _ _ _ _ _ _]
      tunnel: w1497 -> [w1512 w1519 w1527 w1545 w1563 w1598 w1608 w1629 w1633 w1639 w1646 w1657 w1664 w1711 w1719 w1730 w1741]
      tunnel: [w1515 w1518 w1524 w1543 _ w1583 w1609 _ w1635 w1636 w1645 w1656 w1661 _ _ w1727 w1736] -> w1507
      tunnel: [TRUE _ _ _ _ _ _ _ _ _ FALSE FALSE w1663 _ _ TRUE TRUE] -> w1505
      tunnel: w1496 -> [_ _ _ _ _ _ _ _ _ _ _ _ w1662 _ _ _ _]
      tunnel: w1503 -> [w1509 w1516 w1522 w1547 w1574 w1599 w1607 w1630 w1631 w1637 w1641 w1653 w1660 w1713 w1721 w1729 w1737]
      tunnel: [w1509 w1516 w1521 w1546 w1574 w1599 w1607 w1630 w1631 w1637 w1641 w1653 w1660 w1712 w1722 w1729 w1737] -> w1502
      tunnel: [w1511 w1517 w1527 w1544 w1562 w1598 w1608 w1629 w1632 w1638 w1644 w1655 w1664 w1711 w1719 w1728 w1735] -> w1501
      tunnel: w1500 -> [_ _ _ _ _ _ _ w1625 _ _ _ _ _ _ _ _ _]
      tunnel: w1499 -> [_ _ _ _ _ _ _ w1624 _ _ _ _ _ _ _ _ _]
      tunnel: w1495 -> [_ _ _ _ w1560 _ _ _ _ _ _ _ _ _ _ _ _]
      event "Exit": Value Change {
        w1513 = TRUE  # Priority Message
        # "The UI Message Loop handles sending the Exit message to other loops."
        n610 = event-data() -> ()  [unwired: 1 in, 1 out]
        n611 = call-poly "Enqueue Message.vi"("Priority Message? (F)"=w1513, "Message"="Exit", "Message Queue"=w1512) -> ("error out"=w1515:errorcluster, "dup Message Queue"=w1511:refnum<queue>)  [unwired: 7 in]
      }
      event "Force Trigger": Value Change {
        n612 = event-data() -> ()  [unwired: 1 in, 1 out]
        n613 = call-poly "Enqueue Message.vi"("Message"="Force Trigger", "Message Queue"=w1519) -> ("error out"=w1518:errorcluster, "dup Message Queue"=w1517:refnum<queue>)  [unwired: 8 in]
      }
      event Mouse Up {
        # "If we are draging a module and we are over the canvas"
        n614 = event-data() -> ("Coords"=w1526:T10)  [unwired: 1 in]
        n615 = in-place {
          in-place-border: w1527 -> [w1534]
          in-place-border: w1526 -> [w1533]
          in-place-border: [w1532] -> w1525
          w1528 = FALSE ("Down")
          n616 = in-place-cluster #14(w1522) -> ("Drag"=w1530:bool, "Canvas"=w1529:bool)  [unwired: 1 out]
          n617 = Compound Arithmetic op=AND(w1530, w1529) -> (w1531:bool)
          n618 = case shown="False" w1531 {
            tunnel: [_ w1535] -> w1532
            tunnel: w1534 -> [_ w1538]
            tunnel: w1533 -> [_ w1537]
            frame False {
            }
            frame True {
              n619 = property on="Canvas" class="Pict"() -> ("Mouse"=w1540:T73)  [unwired: 2 in, 2 out]
              n620 = Bundle("Coords"=w1537, "Mouse"=w1540) -> (w1536:cluster{"Coords":T10, "Mouse":T73})  [unwired: 1 in]
              "output cluster" <- w1536
              n621 = call-poly "Enqueue Message.vi"("Message Data"=w1536, "Message"="Drop", "Message Queue"=w1538) -> ("error out"=w1535:errorcluster)  [unwired: 7 in, 1 out]
            }
          }
          n622 = in-place-cluster #14("Down"=w1528, "Drag"=w1528, "Canvas"=w1528) -> (w1521:T76)
        }
        n623 = call-poly <vilib>:"Set Cursor.vi"("error in (no error)"=w1525, "icon"=u16 0) -> ("error out"=w1524:errorcluster)  [unwired: 8 in, 1 out]
      }
      event "Palette": Mouse Down {
        n624 = event-data() -> ()  [unwired: 1 in, 1 out]
        n625 = property on="Palette" class="Pict"() -> ("DisabledEnum"=w1542:T83)  [unwired: 2 in, 2 out]
        n626 = call "Enable Disable Enum to Enabled.vi"("Disabled"=w1542) -> ("Enabled"=w1541:bool)
        n627 = case "Is the palette enabled?" shown="True" w1541 {
          tunnel: w1547 -> [w1548 w1559]
          tunnel: [w1548 w1557] -> w1546
          tunnel: w1545 -> [w1549 w1553]
          tunnel: [w1549 w1552] -> w1544
          tunnel: [_ w1551] -> w1543
          frame False {
          }
          frame True {
            # "Select a module"
            n628 = property on="Palette" class="Pict"() -> ("Mouse"=w1550:T73)  [unwired: 2 in, 2 out]
            n629 = Bundle By Name(cluster=w1559, "Down"=TRUE, "Mouse"=w1550, "Drag"=TRUE, "Canvas"=FALSE) -> (w1557:T76)
            n630 = call-poly "Enqueue Message.vi"("Message Data"=w1550, "Message"="Drag Start", "Message Queue"=w1553) -> ("error out"=w1551:errorcluster, "dup Message Queue"=w1552:refnum<queue>)  [unwired: 7 in]
          }
        }
      }
      event Timeout {
        # "Poll for alarm status and display on UI. This could be changed\nto an alarm Event if necessary."
        n631 = event-data() -> ()  [unwired: 1 in, 1 out]
        n632 = call "Tag FGV.vi"("Operation"=Tag_FGV_Operation_Enum."Read Alarms") -> ("alarms"=w1568:T92)  [unwired: 7 in, 7 out]
        n633 = property on="UI Alarms" class="Arr (strict)"() -> ("Number of Columns"=w1571:u32)  [unwired: 2 in, 2 out]
        n634 = call "Is Critical Alarm Set.vi"("alarms"=w1568) -> ("critical alarm?"=w1566:bool)  [unwired: 10 in]
        n635 = call "Alarm UI.vi"("alarms"=w1568) -> ("UI Alarms"=w1573:T71[], "Alarm Model"=→"Alarm Model":T70[])  [unwired: 9 in]
        n636 = Array Size(array=w1573) -> (size(s)=w1572:i32)
        n637 = Greater?(x=w1572, y=w1571) -> (0:w1570:bool)
        n638 = feedback #15() -> (w1567:bool)  [unwired: 1 in]
        n639 = feedback-in #15(w1566) -> ()
        n640 = local write "UI Alarms"(w1573) -> ()
        n641 = property on="UI Alarms" class="Arr (strict)"("HorizScroll"=w1570) -> ()  [unwired: 2 in, 2 out]
        n642 = property on="Alarm Model" class="Arr (strict)"("Visible"=TRUE) -> ()  [unwired: 2 in, 2 out]
        n643 = Compound Arithmetic op=AND(w1566, invert w1567) -> (w1565:bool)
        n644 = case "critical alarm just occured?" shown="False" w1565 {
          tunnel: [w1575 w1579] -> w1562
          tunnel: w1563 -> [w1575 w1578]
          tunnel: w1560 -> [_ w1576]
          frame False {
          }
          frame True {
            n645 = call-poly "Enqueue Message.vi"("Message"="E-Stop", "Message Queue"=w1578) -> ("dup Message Queue"=w1579:refnum<queue>)  [unwired: 8 in, 1 out]
            n646 = call-poly "Enqueue Message.vi"("Message"="Pause", "Message Queue"=w1576) -> ()  [unwired: 8 in, 2 out]
          }
        }
      }
      event User Event {
        w1596 = T93 {"alarm URL"="", "set time"=timestamp(0 s since 1904-01-01), "set user"="", "ack time"=timestamp(0 s since 1904-01-01), "ack user"="", "clear time"=timestamp(0 s since 1904-01-01), "clear user"="", "setpoint"=0.0, "value"=0.0, "priority"=0, "alarm area"="", "alarm description"="", "ack comment"="", "event?"=FALSE, "Refnum"=0}  # Alarm
        # "NI Example on how this works: .. \\LabVIEW 2018\\examples\\lvdsc\\Data and Alarm Historical Logging\\DSC Alarms Demo\\component\\DSC Alarms Event Structure Support.vi"
        # "critical alarm?"
        n647 = event-data() -> ("alarm URL"=w1595:string, "set time"=w1594:timestamp, "set user"=w1593:string, "ack time"=w1592:timestamp, "ack user"=w1591:string, "clear time"=w1590:timestamp, "clear user"=w1589:string, "setpoint"=w1588:dbl, "value"=w1587:dbl, "priority"=w1584:u32, "alarm area"=w1586:string, "alarm description"=w1585:string)  [unwired: 1 in]
        n648 = Bundle By Name(cluster=w1596, "alarm URL"=w1595, "set time"=w1594, "set user"=w1593, "ack time"=w1592, "ack user"=w1591, "clear time"=w1590, "clear user"=w1589, "setpoint"=w1588, "value"=w1587, "priority"=w1584, "alarm area"=w1586, "alarm description"=w1585) -> (w1582:T93)
        n649 = Greater?(x=w1594, y=timestamp(2272129200 s since 1904-01-01)) -> (0:w1581:bool)
        n650 = case "valid time stamp?" shown="True" w1581 {
          tunnel: [w1600 w1605] -> w1583
          tunnel: w1582 -> [_ w1601]
          frame False {
            n651 = call <vilib>:"Clear Errors.vi"() -> ("error out"=w1600:errorcluster)  [unwired: 6 in, 1 out]
          }
          frame True {
            # "Log alarm to alarm\nCSV file."
            n652 = call "Log Alarm FGV.vi"("Alarm"=w1601, "Operation"=Alarm_Log_Operation_Enum."Log Alarm") -> ("error out"=w1605:errorcluster)  [unwired: 9 in]
            n653 = Flatten To XML(anything=w1601) -> (xml string=w1602:string)
            n654 = Concatenate Strings("ALARM: " ("text"), w1602) -> (w1603:string)
            n655 = call "Write to Log File.vi"("error in"=w1605, "text"=w1603) -> ()  [unwired: 9 in, 1 out]
          }
        }
        n656 = disable-structure shown="Disabled" {
          frame Disabled {
            # "Example of\nalarm events using\nsame low level VIs."
            n657 = call "DSC Alarm Event Example.vi"() -> ()  [unwired: 12 in]
          }
          frame Enabled {
          }
        }
      }
      event "UI Alarms": Value Change {
        # "Acknowlege the alarms when it's button is clicked"
        n658 = event-data() -> ()  [unwired: 1 in, 1 out]
        n659 = local read "Alarm Model"() -> (w1611:T70[])
        n660 = call <vilib>:"Clear Errors.vi"() -> ("error out"=w1610:errorcluster)  [unwired: 6 in, 1 out]
        n661 = for {
          shift-right: [w1617] -> w1609
          shift-left: w1610 -> [w1618]
          tunnel: "UI Alarms" -> [w1616] mode=indexing
          tunnel: w1611 -> [w1614] mode=indexing
          n662 = Unbundle By Name(w1614) -> ("Alarm"=w1613:T93)
          n663 = Unbundle By Name(w1616) -> ("Ack"=w1615:bool)
          n664 = case shown="True" w1615 {
            tunnel: w1618 -> [w1619 w1623]
            tunnel: [w1619 w1622] -> w1617
            tunnel: w1613 -> [_ w1620]
            frame False {
            }
            frame True {
              n665 = call "Tag FGV.vi"("Operation"=Tag_FGV_Operation_Enum."Ack Alarm", "Data"=w1620, "error in (no error)"=w1623) -> ("error out"=w1622:errorcluster)  [unwired: 5 in, 7 out]
            }
          }
        }
      }
      event "Alarm History Button": Value Change {
        # "Open Alarm History VI"
        # "Don't care if VI is\nalready running."
        n666 = event-data() -> ()  [unwired: 1 in, 1 out]
        n667 = call-by-ref "Start Asynchronous Call"(reference=w1625, "user event"=w1624) -> (reference out=w1627:refnum<vi>, error out=w1626:errorcluster)  [unwired: 12 in]
        n668 = call <vilib>:"Clear Errors.vi"("error in (no error)"=w1626) -> ()  [unwired: 5 in, 2 out]
        n669 = invoke class="VI (strict)" method="FP.Open"(reference=w1627, "State"=T91."Standard") -> ()  [unwired: 3 in, 5 out]
        n670 = disable-structure shown="Disabled" {
          frame Disabled {
            n671 = call "Alarm History.vi"() -> ()  [unwired: 12 in]
          }
          frame Enabled {
          }
        }
      }
      event "Settings": Value Change {
        n672 = event-data() -> ()  [unwired: 1 in, 1 out]
        n673 = call-poly "Enqueue Message.vi"("Message"="Launch Settings Dialog", "Message Queue"=w1633) -> ("error out"=w1635:errorcluster, "dup Message Queue"=w1632:refnum<queue>)  [unwired: 8 in]
      }
      event "Start Log": Value Change {
        n674 = event-data() -> ()  [unwired: 1 in, 1 out]
        n675 = call-poly "Enqueue Message.vi"("Message"="Start Log", "Message Queue"=w1639) -> ("error out"=w1636:errorcluster, "dup Message Queue"=w1638:refnum<queue>)  [unwired: 8 in]
      }
      event "Pause Log Button": Value Change {
        n676 = event-data() -> ()  [unwired: 1 in, 1 out]
        n677 = global write "Main Globals.vi" "Pause Log"("Pause Log Button") -> ()
        n678 = disable-structure shown="Enabled" {
          disable-tunnel: w1646 -> [w1651 w1652]
          disable-tunnel: [w1650 _] -> w1645
          disable-tunnel: [w1649 w1652] -> w1644
          disable-tunnel: "Pause Log Button" -> [w1647 _]
          frame Disabled {
            n679 = call-poly "Enqueue Message.vi"("Message Data"=w1647, "Message"="Pause Log", "Message Queue"=w1651) -> ("error out"=w1650:errorcluster, "dup Message Queue"=w1649:refnum<queue>)  [unwired: 7 in]
          }
          frame Enabled {
          }
        }
      }
      event "E-Stop": Value Change {
        n680 = event-data() -> ()  [unwired: 1 in, 1 out]
        n681 = call-poly "Enqueue Message.vi"("Message"="E-Stop", "Message Queue"=w1657) -> ("error out"=w1656:errorcluster, "dup Message Queue"=w1655:refnum<queue>)  [unwired: 8 in]
      }
      event Menu Selection (User) {
        n682 = event-data() -> ("ItemTag"=w1659:string)  [unwired: 1 in]
        n683 = case shown="\"TCP Setup\"" w1659 {
          tunnel: w1664 -> [_ _ _ w1676 w1679 w1682 w1686 w1688 w1691 w1694 w1698 w1701 w1704 w1709]
          tunnel: [_ _ _ _ _ _ _ _ _ _ _ _ _ TRUE] -> w1663
          tunnel: w1662 -> [_ _ w1674 _ _ _ _ _ _ _ _ _ _ _]
          tunnel: [w1665 w1666 w1673 w1677 w1680 w1683 w1687 w1689 w1692 w1695 w1697 w1700 w1703 w1708] -> w1661
          frame Default {
            n684 = call <vilib>:"Clear Errors.vi"() -> ("error out"=w1665:errorcluster)  [unwired: 6 in, 1 out]
          }
          frame "Open BMP" {
            n685 = call "File Dialog"() -> ("selected path"=w1667:path, "cancelled"=w1668:bool)  [unwired: 12 in, 2 out]
            n686 = case shown="False" w1668 {
              tunnel: w1667 -> [w1670 _]
              frame False {
                n687 = call "Empty Picture"() -> ("empty picture"=w1669:picture)
                n688 = call "Draw BMP at Location.vi"("selected path"=w1670, "picture in"=w1669) -> ("image data"=→"image data":T74, "picture out"=→"Canvas":picture)  [unwired: 7 in, 1 out]
              }
              frame True {
              }
            }
            n689 = call <vilib>:"Clear Errors.vi"() -> ("error out"=w1666:errorcluster)  [unwired: 6 in, 1 out]
          }
          frame "DAQSettings" {
            # "Open the DAQ Settings dialog"
            n690 = call-poly "Enqueue Message.vi"("Message"="DAQ-Settings", "Message Queue"=w1674) -> ("error out"=w1673:errorcluster)  [unwired: 8 in, 1 out]
          }
          frame "Open Campaign" {
            n691 = call-poly "Enqueue Message.vi"("Message"="Open Campaign", "Message Queue"=w1676) -> ("error out"=w1677:errorcluster)  [unwired: 8 in, 1 out]
          }
          frame "Save Campaign" {
            n692 = call-poly "Enqueue Message.vi"("Message"="Save Campaign", "Message Queue"=w1679) -> ("error out"=w1680:errorcluster)  [unwired: 8 in, 1 out]
          }
          frame "Save Campaign As..." {
            n693 = call-poly "Enqueue Message.vi"("Message"="Save Campaign As", "Message Queue"=w1682) -> ("error out"=w1683:errorcluster)  [unwired: 8 in, 1 out]
          }
          frame "FileSettings" {
            # "Open the File Settings dialog"
            n694 = call-poly "Enqueue Message.vi"("Message"="File-Settings", "Message Queue"=w1686) -> ("error out"=w1687:errorcluster)  [unwired: 8 in, 1 out]
          }
          frame "Set Sequence" {
            n695 = call-poly "Enqueue Message.vi"("Message"="Launch Sequence Dialog", "Message Queue"=w1688) -> ("error out"=w1689:errorcluster)  [unwired: 8 in, 1 out]
          }
          frame "Set Data Rate" {
            n696 = call-poly "Enqueue Message.vi"("Message"="Launch Data Rate Dialog", "Message Queue"=w1691) -> ("error out"=w1692:errorcluster)  [unwired: 8 in, 1 out]
          }
          frame "TCP Setup" {
            n697 = call-poly "Enqueue Message.vi"("Message"="Launch TCP Setup Dialog", "Message Queue"=w1694) -> ("error out"=w1695:errorcluster)  [unwired: 8 in, 1 out]
          }
          frame "Reset Global Variables" {
            n698 = call-poly "Enqueue Message.vi"("Message"="Reset Global Variables", "Message Queue"=w1698) -> ("error out"=w1697:errorcluster)  [unwired: 8 in, 1 out]
          }
          frame "Launch Calibration Dialog" {
            n699 = call-poly "Enqueue Message.vi"("Message"="Launch Calibration Dialog", "Message Queue"=w1701) -> ("error out"=w1700:errorcluster)  [unwired: 8 in, 1 out]
          }
          frame "Add Note" {
            n700 = call-poly "Enqueue Message.vi"("Message"="Launch Note Dialog", "Message Queue"=w1704) -> ("error out"=w1703:errorcluster)  [unwired: 8 in, 1 out]
          }
          frame "Exit" {
            w1706 = TRUE  # Priority Message
            n701 = call-poly "Enqueue Message.vi"("Priority Message? (F)"=w1706, "Message"="Exit", "Message Queue"=w1709) -> ("error out"=w1708:errorcluster)  [unwired: 7 in, 1 out]
          }
        }
      }
      event "Canvas": Mouse Enter {
        n702 = event-data() -> ()  [unwired: 1 in, 1 out]
        n703 = Unbundle By Name(w1713) -> ("Drag"=w1714:bool)
        n704 = case shown="False" w1714 {
          tunnel: w1713 -> [w1715 w1718]
          tunnel: [w1715 w1717] -> w1712
          frame False {
          }
          frame True {
            n705 = Bundle By Name(cluster=w1718, "Canvas"=TRUE) -> (w1717:T76)
          }
        }
      }
      event "Canvas": Mouse Leave {
        n706 = event-data() -> ()  [unwired: 1 in, 1 out]
        n707 = Unbundle By Name(w1721) -> ("Canvas"=w1720:bool)
        n708 = case shown="False" w1720 {
          tunnel: w1721 -> [w1723 w1726]
          tunnel: [w1723 w1725] -> w1722
          frame False {
          }
          frame True {
            n709 = Bundle By Name(cluster=w1726, "Canvas"=FALSE) -> (w1725:T76)
          }
        }
      }
      event Panel Close? {
        w1731 = TRUE  # Priority Message
        # "Send the 'Confirm Quit' message if the user closes the panel of the VI. Discard the event so the 'Confirm Quit' message has a chance to run."
        n710 = event-data() -> ()  [unwired: 1 in, 1 out]
        n711 = invoke class="VI" method="FP.Close"() -> ()  [unwired: 3 in, 3 out]
        n712 = call-poly "Enqueue Message.vi"("Priority Message? (F)"=w1731, "Message"="Exit", "Message Queue"=w1730) -> ("error out"=w1727:errorcluster, "dup Message Queue"=w1728:refnum<queue>)  [unwired: 7 in]
        n713 = event-data("Discard?"=TRUE) -> ()  [unwired: 1 in, 1 out]
      }
      event "End Program": Value Change {
        w1738 = FALSE  # Priority Message
        # "Send the 'Confirm Quit' message if the user closes the panel of the VI. Discard the event so the 'Confirm Quit' message has a chance to run."
        n714 = event-data() -> ()  [unwired: 1 in, 1 out]
        n715 = call-poly "Enqueue Message.vi"("Priority Message? (F)"=w1738, "Message"="Exit", "Message Queue"=w1741) -> ("error out"=w1736:errorcluster, "dup Message Queue"=w1735:refnum<queue>)  [unwired: 7 in]
      }
    }
    n716 = call "Error Handler - Event Handling Loop.vi"("error in (no error)"=w1507, "Message Queue"=w1501) -> ("dup error in"=w1506:errorcluster)  [unwired: 8 in, 1 out]
  }
  n717 = invoke class="VI" method="Ctrl Val.Set"(reference=w72, error in=w70, "Control Name"="Message Queues", "Value"=w29) -> (reference out=w71:refnum<vi>, error out=w69:errorcluster)  [unwired: 1 in, 3 out]
  n718 = invoke class="VI" method="Run VI"(reference=w71, error in=w69, "Wait until done"=FALSE ("Wait Until Done"), "Auto Dispose Ref"=FALSE ("Auto Dispose Reference")) -> (reference out=w74:refnum<vi>)  [unwired: 1 in, 4 out]
  n719 = invoke on="Sub Panel" class="SubPnl" method="Insert VI"("VI Ref"=w74) -> (error out=→"error out":errorcluster)  [unwired: 3 in, 3 out]
  n720 = Unregister For Events(event registration refnum=w83, error in=w86) -> (error out=w53:errorcluster)
  n721 = disable-structure shown="Enabled" {
    frame Disabled {
      n722 = call "Feed Module (Main).vi"() -> ()  [unwired: 12 in]
      n723 = call "Tag FGV.vi"() -> ()  [unwired: 6 in, 6 out]
      n724 = call "TT (Main).vi"() -> ()  [unwired: 12 in]
      n725 = call "PT (Main).vi"() -> ()  [unwired: 12 in]
      n726 = call "History Graph Message Loop.vi"() -> ()  [unwired: 11 in, 1 out]
      n727 = call "Scale Module (Main).vi"() -> ()  [unwired: 12 in]
      n728 = call "Log Alarm FGV.vi"() -> ()  [unwired: 11 in, 1 out]
      n729 = call "Pump Module (Main).vi"() -> ()  [unwired: 12 in]
    }
    frame Enabled {
    }
  }
  n730 = Generate User Event(user event=w51, event data cluster=w50, error in=w53) -> (error out=w56:errorcluster)  [unwired: 1 in, 1 out]
  n731 = invoke class="VI (strict)" method="FP.Close"(reference=w52, error in=w56) -> (error out=w55:errorcluster)  [unwired: 1 in, 2 out]
  n732 = call <vilib>:"Clear Errors.vi"("error in (no error)"=w55) -> ("error out"=w54:errorcluster)  [unwired: 5 in, 1 out]
  n733 = Close Reference(reference=w52, error in (no error)=w54) -> ()  [unwired: 1 out]
  n734 = Merge Errors(w53, w87, w36, w35, w34, w33, w32) -> (w85:errorcluster)
  n735 = call "Destroy User Event - Stop.vi"("error in (no error)"=w85, "User Event - Stop"=w84) -> ("error out"=w38:errorcluster)  [unwired: 9 in]
  n736 = call "Close File.vi"("error in"=w38) -> ("error out"=w12:errorcluster)  [unwired: 10 in]
  n737 = Release Queue(queue=w13, error in (no error)=w12) -> (error out=w11:errorcluster)  [unwired: 1 in, 2 out]
  n738 = Release Queue(queue=w14, error in (no error)=w11) -> (error out=w10:errorcluster)  [unwired: 1 in, 2 out]
  n739 = Release Queue(queue=w15, error in (no error)=w10) -> (error out=w9:errorcluster)  [unwired: 1 in, 2 out]
  n740 = for {
    tunnel: w16 -> [w1744] mode=indexing
    tunnel: w9 -> [w1743]
    tunnel: [w1742] -> _ mode=indexing
    tunnel: [w1742] -> w8
    n741 = Release Queue(queue=w1744, error in (no error)=w1743) -> (error out=w1742:errorcluster)  [unwired: 1 in, 2 out]
  }
  n742 = Merge Errors(w8) -> (w7:errorcluster)
  n743 = Release Queue(queue=w17, error in (no error)=w7) -> (error out=w6:errorcluster)  [unwired: 1 in, 2 out]
  n744 = Release Queue(queue=w18, error in (no error)=w6) -> (error out=w5:errorcluster)  [unwired: 1 in, 2 out]
  n745 = Release Queue(queue=w26, error in (no error)=w5) -> (error out=w4:errorcluster)  [unwired: 1 in, 2 out]
  n746 = Release Queue(queue=w27, error in (no error)=w4) -> (error out=w3:errorcluster)  [unwired: 1 in, 2 out]
  n747 = Release Queue(queue=w25, error in (no error)=w3) -> (error out=w2:errorcluster)  [unwired: 1 in, 2 out]
  n748 = Release Queue(queue=w28, error in (no error)=w2) -> (error out=w1:errorcluster)  [unwired: 1 in, 2 out]
  n749 = disable-structure shown="Default" {
    disable-tunnel: w1 -> [_ _]
    frame condition #0 {
      # "Call Quit LabVIEW if running as a built application."
      n750 = Quit LabVIEW() -> ()  [unwired: 1 in]
    }
    frame condition #1 (active) {
    }
  }
